vi "TLB Native Dynamic Events ver 0.17g.vi"() -> ()   [LabVIEW 2018]
uses:
  Labview Training Phase 2/Enum Controls/States for Action Engine.ctl
  TLB Type Definitions/State Type Definitions.ctl
  TLB Type Definitions/Intruction Type Definitions.ctl
  TLB Type Definitions/Encoder cluster.ctl
  TLB Type Definitions/PING CLUSTER.ctl
  <vilib>/Studica/Studica Toolkit/NavX/NavX.lvlib
  <vilib>/Studica/Studica Toolkit/Background/DIO Channel.ctl
  Underlying VI's/NavX VI/navX type def.ctl
  <vilib>/Studica/Studica Toolkit/Background/I2C Channel.ctl
  TLB Type Definitions/Vision cluster.ctl
  <vilib>/NI_Real-Time Target Support.lvlib
  TLB Type Definitions/Stepper cluster.ctl
  Experimental VI's/Archived VI's/MOTOR CONTROL NO PID Type Def.ctl
  Underlying VI's/I2C Master VI/I2C MASTER Type Def.ctl
  Underlying VI's/I2C Master VI/I2C_MASTER_WRITE_NEW Type Def.ctl
  <vilib>/userdefined/High Color/IMAQdx.ctl
  Underlying VI's/I2C Master VI/Arduino_Interfacing.ctl
  TLB Type Definitions/Yaw Cluster.ctl
  TLB Type Definitions/Time cluster.ctl
  TLB Type Definitions/Y Stepper cluster.ctl
  Underlying VI's/Modified webcam FGV/Webcam AE.ctl
  Underlying VI's/Elasped Timer/Elapsed timer control.ctl
  Underlying VI's/Motor Control VI with PID/MOTOR CONTROL WITH PID AE DATA MODE TYPE DEF.ctl
  Underlying VI's/Motor Control VI with PID/MOTOR CONTROL WITH PID AE DIRECTION TYPE DEF.ctl
  TLB Type Definitions/IR Sensor Type Def.ctl
  <vilib>/myRIO/Common/Instrument Driver Framework/myRIO v1.0/AI/typedefs/AI Channels Enum.ctl
  <vilib>/myRIO/Common/Instrument Driver Framework/myRIO v1.0/AI/typedefs/AI Channels List.ctl
  TLB Type Definitions/Motor Speed Cluster.ctl
  <vilib>/Utility/RT CPU Load.ctl
panel:
  out "x-y":dbl
  out "Left IR Sensor":dbl
  out "Obstacle detected":bool
  out "Speed & distance":T1
  out "Object Center Coordinates":cluster{"x":sgl, "y":sgl}
  out "Object detection cluster":T2
  out "Time up flag":bool
  out "Task selection":u8
  in  "Object recognition mode":enum16{"Ball", "Soap", "Gel", "Pipe", "None"}(ring)
  out "NavX Readings":T3
  out "Arduino Data":T4
  out "CPU loads":T5[](array[typedef]) {"ISR (%)" format="%#.2f"; "Idle (%)" format="%#.2f"; "Background (%)" format="%#.2f"; "Normal (%)" format="%#.2f"; "Above Normal (%)" format="%#.2f"; "High (%)" format="%#.2g"; "Timed Structures (%)" format="%#.2g"; "Time Critical (%)" format="%#.2g"; "Total (%)" format="%#.2g"}
  out "TASK ENABLE":bool
  out "Rising Edge":bool
  in  "Green LED":bool
  out "I2C Error":errorcluster
  out "State Logic":T6=enum."Startup"
  out "elements":T7[](array[typedef])
  in  "STOP TASK":bool
  in  "OK Button":bool
  in  "STOP":bool
  out "error out":errorcluster
  out "Action Queue Items":i32
  out "State Logic Queue Items":i32
  out "Action Queues items":string[](array[string])=["Hardware reset", "Software reset", ""]
  out "Action State":string
  # "System Health Status Update"
  # "VISION"
  # "TLB FRAMEWORK STATUS"
  # "Test Programme written by Calvin Loke    Dated: 28 Aug 2019\nTest Programme revised by Dr Alex See   Dated 30 Aug 2019\n\nRevision date: 20/03/2020\nProgramme version:   TLB Native Dynamic Events ver 0.14a"
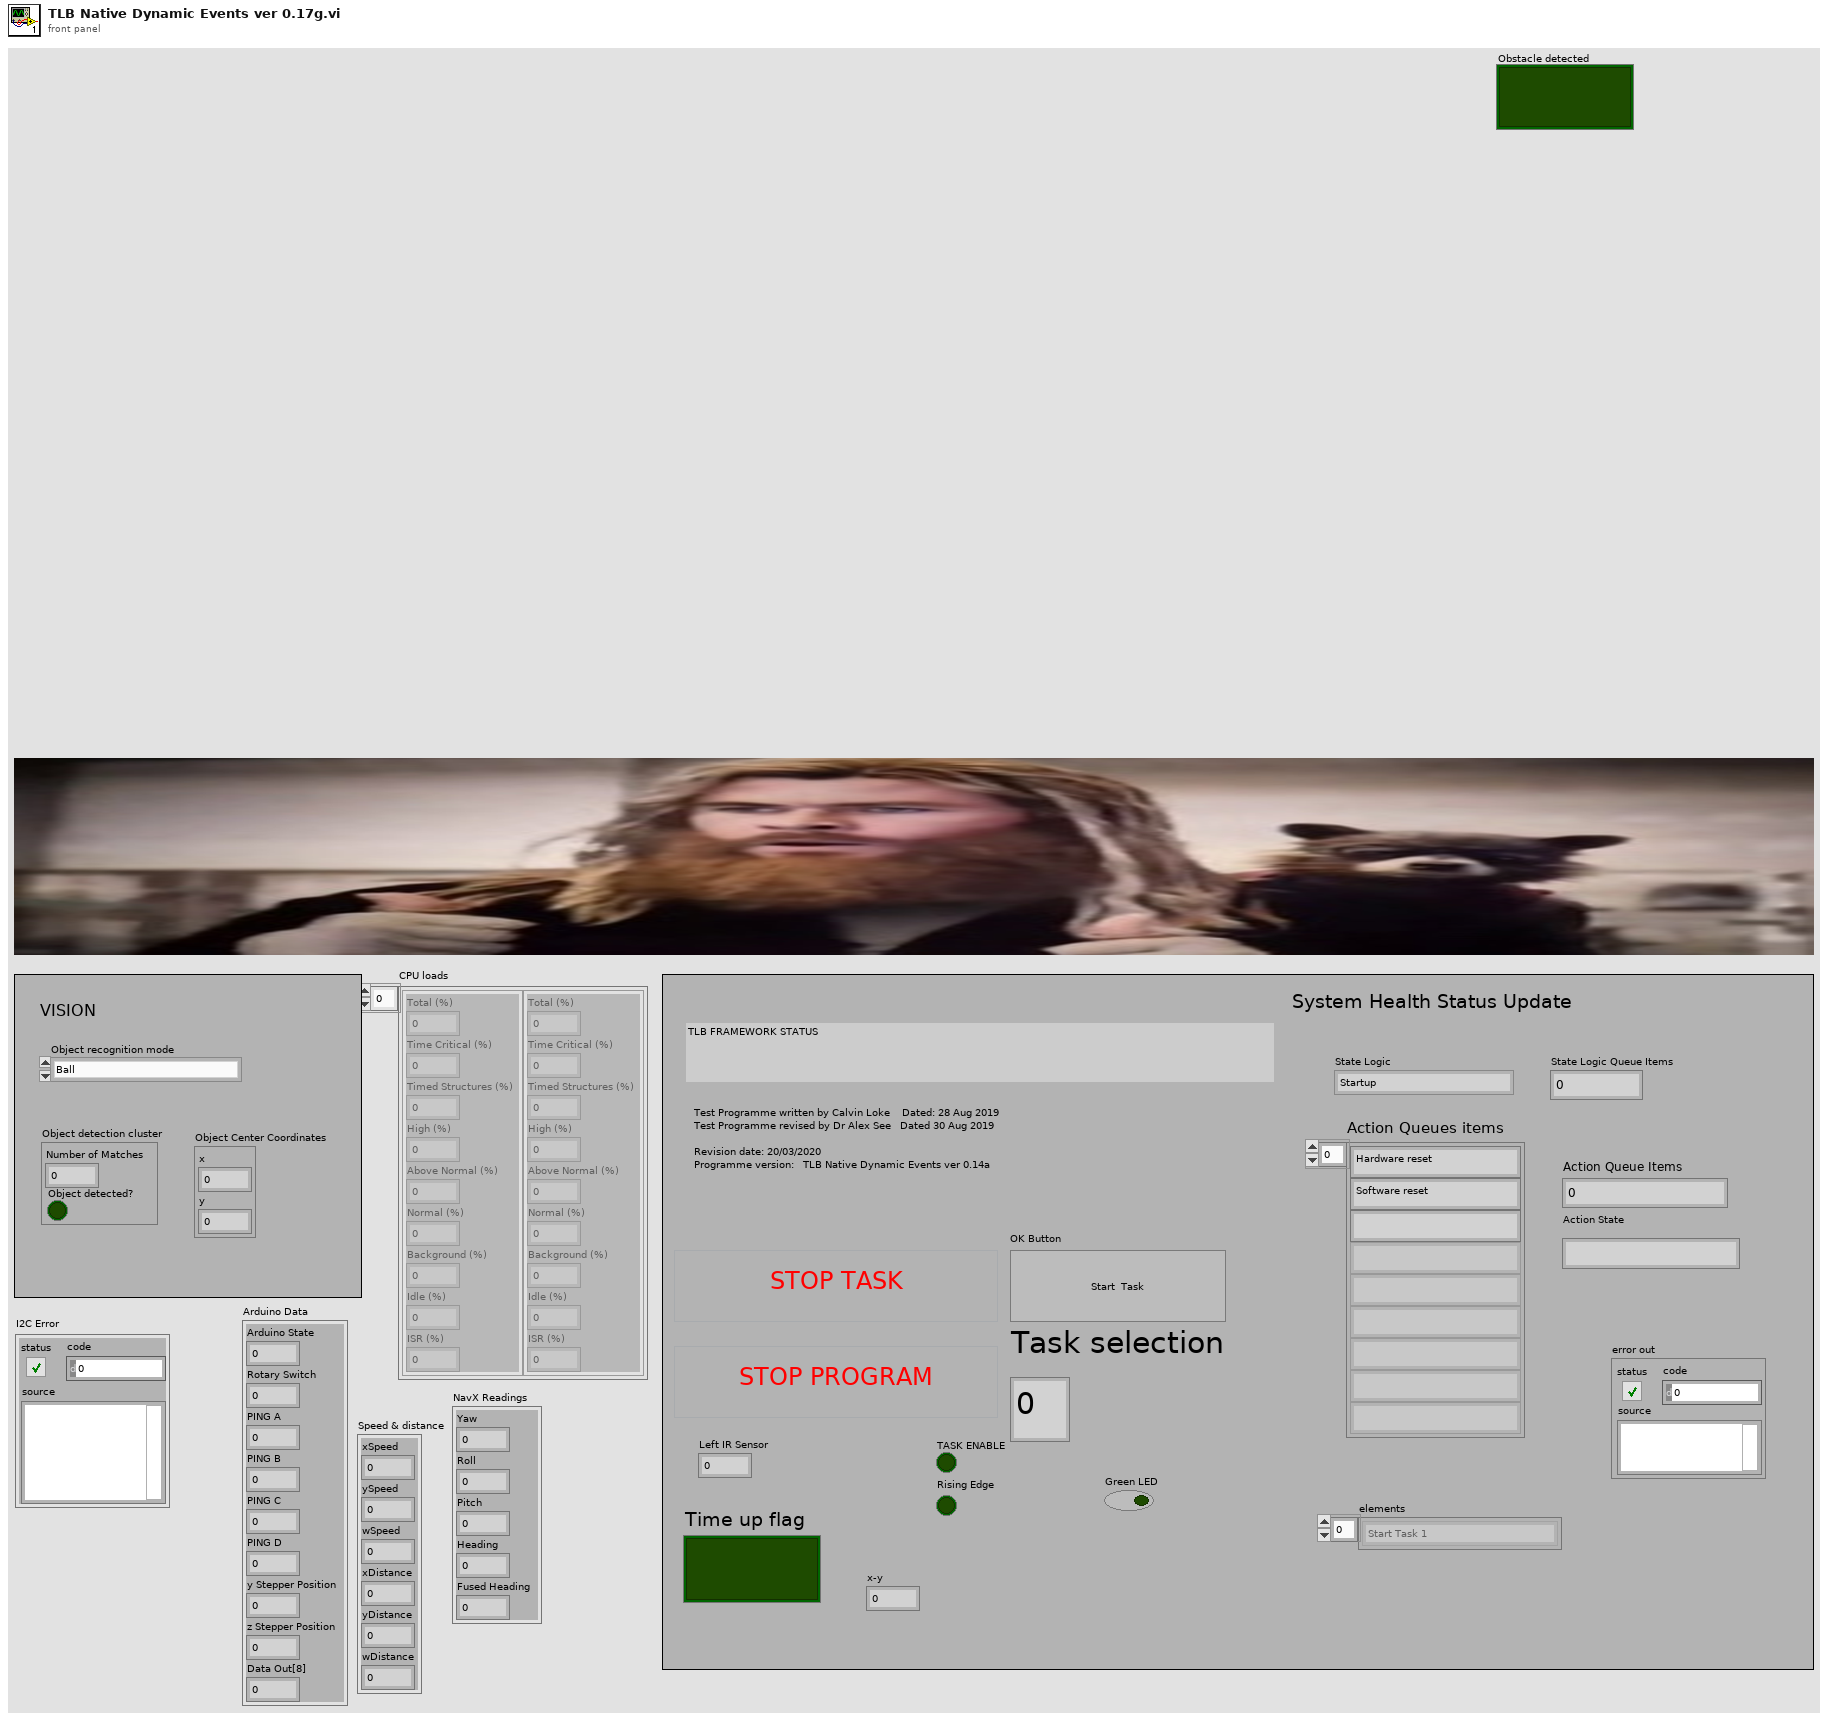
[diagram p1: front panel]
types:
  T1 = cluster{"xSpeed":dbl, "ySpeed":dbl, "wSpeed":dbl, "xDistance":dbl, "yDistance":dbl, "wDistance":dbl}
  T2 = cluster{"Number of Matches":i32, "Object detected?":bool}
  T3 = cluster{"Yaw":dbl, "Roll":dbl, "Pitch":dbl, "Heading":dbl, "Fused Heading":dbl}
  T4 = cluster{"Arduino State":u8, "Rotary Switch":u8, "PING A":u8, "PING B":u8, "PING C":u8, "PING D":u8, "y Stepper Position":u8, "z Stepper Position":u8, "Data Out[8]":u8}
  T5 = typedef "NI_Real-Time Target Support.lvlib/RT CPU Load.ctl" = cluster{"Total (%)":dbl, "Time Critical (%)":dbl, "Timed Structures (%)":dbl, "High (%)":dbl, "Above Normal (%)":dbl, "Normal (%)":dbl, "Background (%)":dbl, "Idle (%)":dbl, "ISR (%)":dbl}
  T6 = typedef "State Type Definitions.ctl" = enum16{"None", "Startup", "Move to Angle", "True Stop", "Idle", "Shutdown", "Task 1A", "Task 1B", "Task 2:Raise Arm", "Task 2:Sensor Mode", "Task 2:Reverse Mode", "Task 3", "Task 4_A", "Task 4_B", "Task 4_C", "Task 4_D", "Task 5A", "Task 5B", "Task 5C", "Task 5D", "Task 5E: POSITION ARM", "Task 5F: ARM GRAB HEIGHT", "Task 5G: CLOSE CLAW", "Task 5H: RAISE ARM", "Task 6_A", "Task 6_B", "Task 7", "Task 8A: RAISE ARM", "Task 8B: MOVE TO BOX", "Task 8C: CAM BURST", "Task 8D: PROCESS IMAGE", "Task 8E: ROBOT ADJUST", "Task 8F: CAM BURST 2", "Task 8G: PROCESS IMAGE 2", "Task 8H: ARM ADJUST", "Task 8I: ARM GRAB HEIGHT", "Task 8J: CLOSE CLAW", "Task 8K: RAISE MY SWORD", "Task 9A: Raise Arm", "Task 9B: Rotate to Angle", "Task 9C: Detect Box", "Task 9D: MOVE FORWARD", "Task 9E: MOVE LEFT", "Task 9F: SCAN IMAGE", "Task 9G: PROCESS COLOUR", "Task 9H: MOVE RIGHT", "Task 9I: SCAN IMAGE", "Task 9J: PROCESS COLOUR", "Task 9K: ROTATE 90 CW", "Task 9L: MOVE FORWARD", "Task 9M: MOVE RIGHT", "Task 9N: SCAN IMAGE", "Task 9O: PROCESS COLOUR", "Task 9P: MOVE RIGHT", "Task 9Q: SCAN IMAGE", "Task 9R: PROCESS COLOUR", "Task A1: Raise Arm", "Task A2: Rotate to Angle", "Task A3: Move Forward", "Task A4: Rotate CW 90"}
  T7 = typedef "Intruction Type Definitions.ctl" = enum16{"None", "Start Task 1", "Start Task 2", "Start Task 3", "Start Task 4", "Start Task 5", "Start Task 6", "Start Task 7", "Start Task 8 - BALL", "Start Task 8 - Gel", "Start Task 8 - Pipe", "Start Task 8 - Soap", "Start Task 9", "Start Task A", "Start Task B", "Exit"}
  T8 = typedef "Motor Speed Cluster.ctl" = cluster{"ySpeed":dbl, "xSpeed":dbl, "wSpeed":dbl}
  T9 = typedef "IR Sensor Type Def.ctl" = cluster{"Left IR Sensor":dbl, "Arm IR Sensor":dbl, "Bottom IR Sensor":dbl}
  T10 = typedef "Y Stepper cluster.ctl" = cluster{"yStepper desired":u8}
  T11 = typedef "Time cluster.ctl" = cluster{"Time up flag":bool, "SET TIME TO CHECK":dbl}
  T12 = typedef "Yaw Cluster.ctl" = cluster{"Yaw":dbl, "Compass":dbl}
  T13 = typedef "Stepper cluster.ctl" = cluster{"y Stepper Position":u8, "z Stepper Position":u8}
  T14 = typedef "DIO Channel.ctl" = enum16{"Not Connected", "A/DIO1", "A/DIO2", "A/DIO3", "A/DIO4", "A/DIO5", "A/DIO6", "A/DIO7", "A/DIO13", "B/DIO1", "B/DIO2", "B/DIO3", "B/DIO4", "B/DIO5", "B/DIO6", "B/DIO7", "B/DIO13", "C/DIO0", "C/DIO1", "C/DIO2", "C/DIO3", "C/DIO4", "C/DIO5", "C/DIO6", "C/DIO7"}
  T15 = typedef "Vision cluster.ctl" = cluster{"Recognized Object":bool, "Object X coordinate":dbl, "Object Y coordinate":dbl}
  T16 = typedef "PING CLUSTER.ctl" = cluster{"PING_A":u8, "PING_B":u8, "PING_C":u8, "PING_D":u8}
  T17 = typedef "Encoder cluster.ctl" = cluster{"xDistance":dbl, "yDistance":dbl, "wDistance":dbl}
  T18 = cluster{"DIO Channel":T14, "FPGA VI Reference Out":refnum<k20>}
  T19 = typedef "navX type def.ctl" = enum16{"Get i2C reference", "Read Values", "Zero Yaw"}
  T20 = typedef "Arduino_Interfacing.ctl" = enum16{"Initialize", "Write to Arduino", "Read From Arduino"}
  T21 = typedef "I2C Channel.ctl" = enum16{"Not Connected", "A", "B"}
  T22 = typedef "States for Action Engine.ctl" = enum16{"Initialize", "Write", "Read"}
  T23 = cluster{"I2C Ref Out":cluster{"I2C Channel":T21, "FPGA VI Reference Out":refnum<k20>}, "Connected":bool, "Slave Address (7-bit)":u8, "Registry":u8[]}
  T24 = typedef "Intruction Type Definitions.ctl" = enum16{"None", "Start Task 1", "Start Task 2", "Start Task 3", "Start Task 4", "Start Task 5", "Start Task 6", "Start Task 7", "Start Task 8", "Start Task 9", "Start Task A", "Start Task B", "Exit"}
  T25 = typedef "IMAQ Image.ctl" = refnum<image>
  T26 = typedef "State Type Definitions.ctl" = enum16{"None", "Startup", "Move to Angle", "True Stop", "Idle", "Shutdown", "Task 1", "Task 2:Raise Arm", "Task 2:Sensor Mode", "Task 2:Reverse Mode", "Task 3", "Task 4_A", "Task 4_B", "Task 4_C", "Task 4_D", "Task 5A: ARM CAM HEIGHT", "Task 5B: MOVE TO BOX", "Task 5C: CAM BURST", "Task 5D: PROCESS IMAGE", "Task 5E: POSITION ARM", "Task 5F: ARM GRAB HEIGHT", "Task 5G: CLOSE CLAW", "Task 5H: RAISE ARM", "Task 6_A", "Task 6_B", "Task 7", "Task 8A: RAISE ARM", "Task 8B: MOVE TO BOX", "Task 8C: CAM BURST", "Task 8D: PROCESS IMAGE", "Task 8E: ROBOT ADJUST", "Task 9A: Raise Arm", "Task 9B: Rotate to Angle", "Task 9C: Rotation alignmnet", "Task B"}
  T27 = typedef "MOTOR CONTROL WITH PID AE DIRECTION TYPE DEF.ctl" = enum16{"y-axis movement", "x-axis movement", "rotation", "stop", "reset encoders"}
  T28 = typedef "MOTOR CONTROL WITH PID AE DATA MODE TYPE DEF.ctl" = enum16{"Init AE", "Write to AE", "Read from AE"}
  T29 = typedef "Elapsed timer control.ctl" = enum16{"Start", "Pause", "Initialize"}
  T30 = typedef "I2C_MASTER_WRITE_NEW Type Def.ctl" = enum16{"Ultrasonic sensors", "Stepper origin", "zStepper 13.3k", "zStepper 13k", "zStepper 12k", "zStepper 11k", "zStepper 10k", "zStepper 9k", "zStepper 8k", "zStepper 7k", "zStepper 6k", "zStepper 5k", "zStepper 4k", "zStepper 3k", "zStepper 2k", "zStepper 1k", "zStepper 900", "zStepper 800", "zStepper 700", "zStepper 600", "zStepper 500", "zStepper 400", "zStepper 300", "zStepper 200", "zStepper 100", "zStepper 0", "yStepper control", "Open Claw", "Close Claw", "Soft Reset"}
  T31 = typedef "Webcam AE.ctl" = enum16{"Initialize Camera", "Open Camera", "Continuous Acquisition", "Close Camera", "Retrieve Image", "Dispose Camera Image Buffer"}
  T32 = typedef "IMAQdx.ctl" = refnum<k21>
  T33 = typedef "Webcam AE.ctl" = enum16{"Initialize Camera", "Open Camera", "Continuous Acquisition", "Close Camera", "Retrieve Image", "Dispose Image Buffers"}
  T34 = typedef "MOTOR CONTROL NO PID Type Def.ctl" = enum16{"Init", "Front Back", "Left Right", "Rotate", "Stop", "Latch"}
  T35 = typedef "AI Channels List.ctl" = T36[]
  T36 = typedef "AI Channels Enum.ctl" = enum16{"Not Connected", "AudioIn/Left", "AudioIn/Right", "C/AI0", "C/AI1", "A/AI0", "A/AI1", "A/AI2", "A/AI3", "A/AI4", "A/AI5", "A/AI6", "A/AI7", "B/AI0", "B/AI1", "B/AI2", "B/AI3", "B/AI4", "B/AI5", "B/AI6", "B/AI7", "AI/AI0", "AI/AI1", "AI/AI2", "AI/AI3", "A/AI0 (DIFF)", "A/AI1 (DIFF)", "A/AI2 (DIFF)", "A/AI3 (DIFF)", "B/AI0 (DIFF)", "B/AI1 (DIFF)", "B/AI2 (DIFF)", "B/AI3 (DIFF)"}
  T37 = typedef "I2C MASTER Type Def.ctl" = enum16{"Last State", "Mode 0", "Mode 1", "Mode 2", "Mode 3", "Mode 4", "Mode 5", "Mode 6", "Mode 7", "Mode 8", "Mode 9", "Mode 10"}
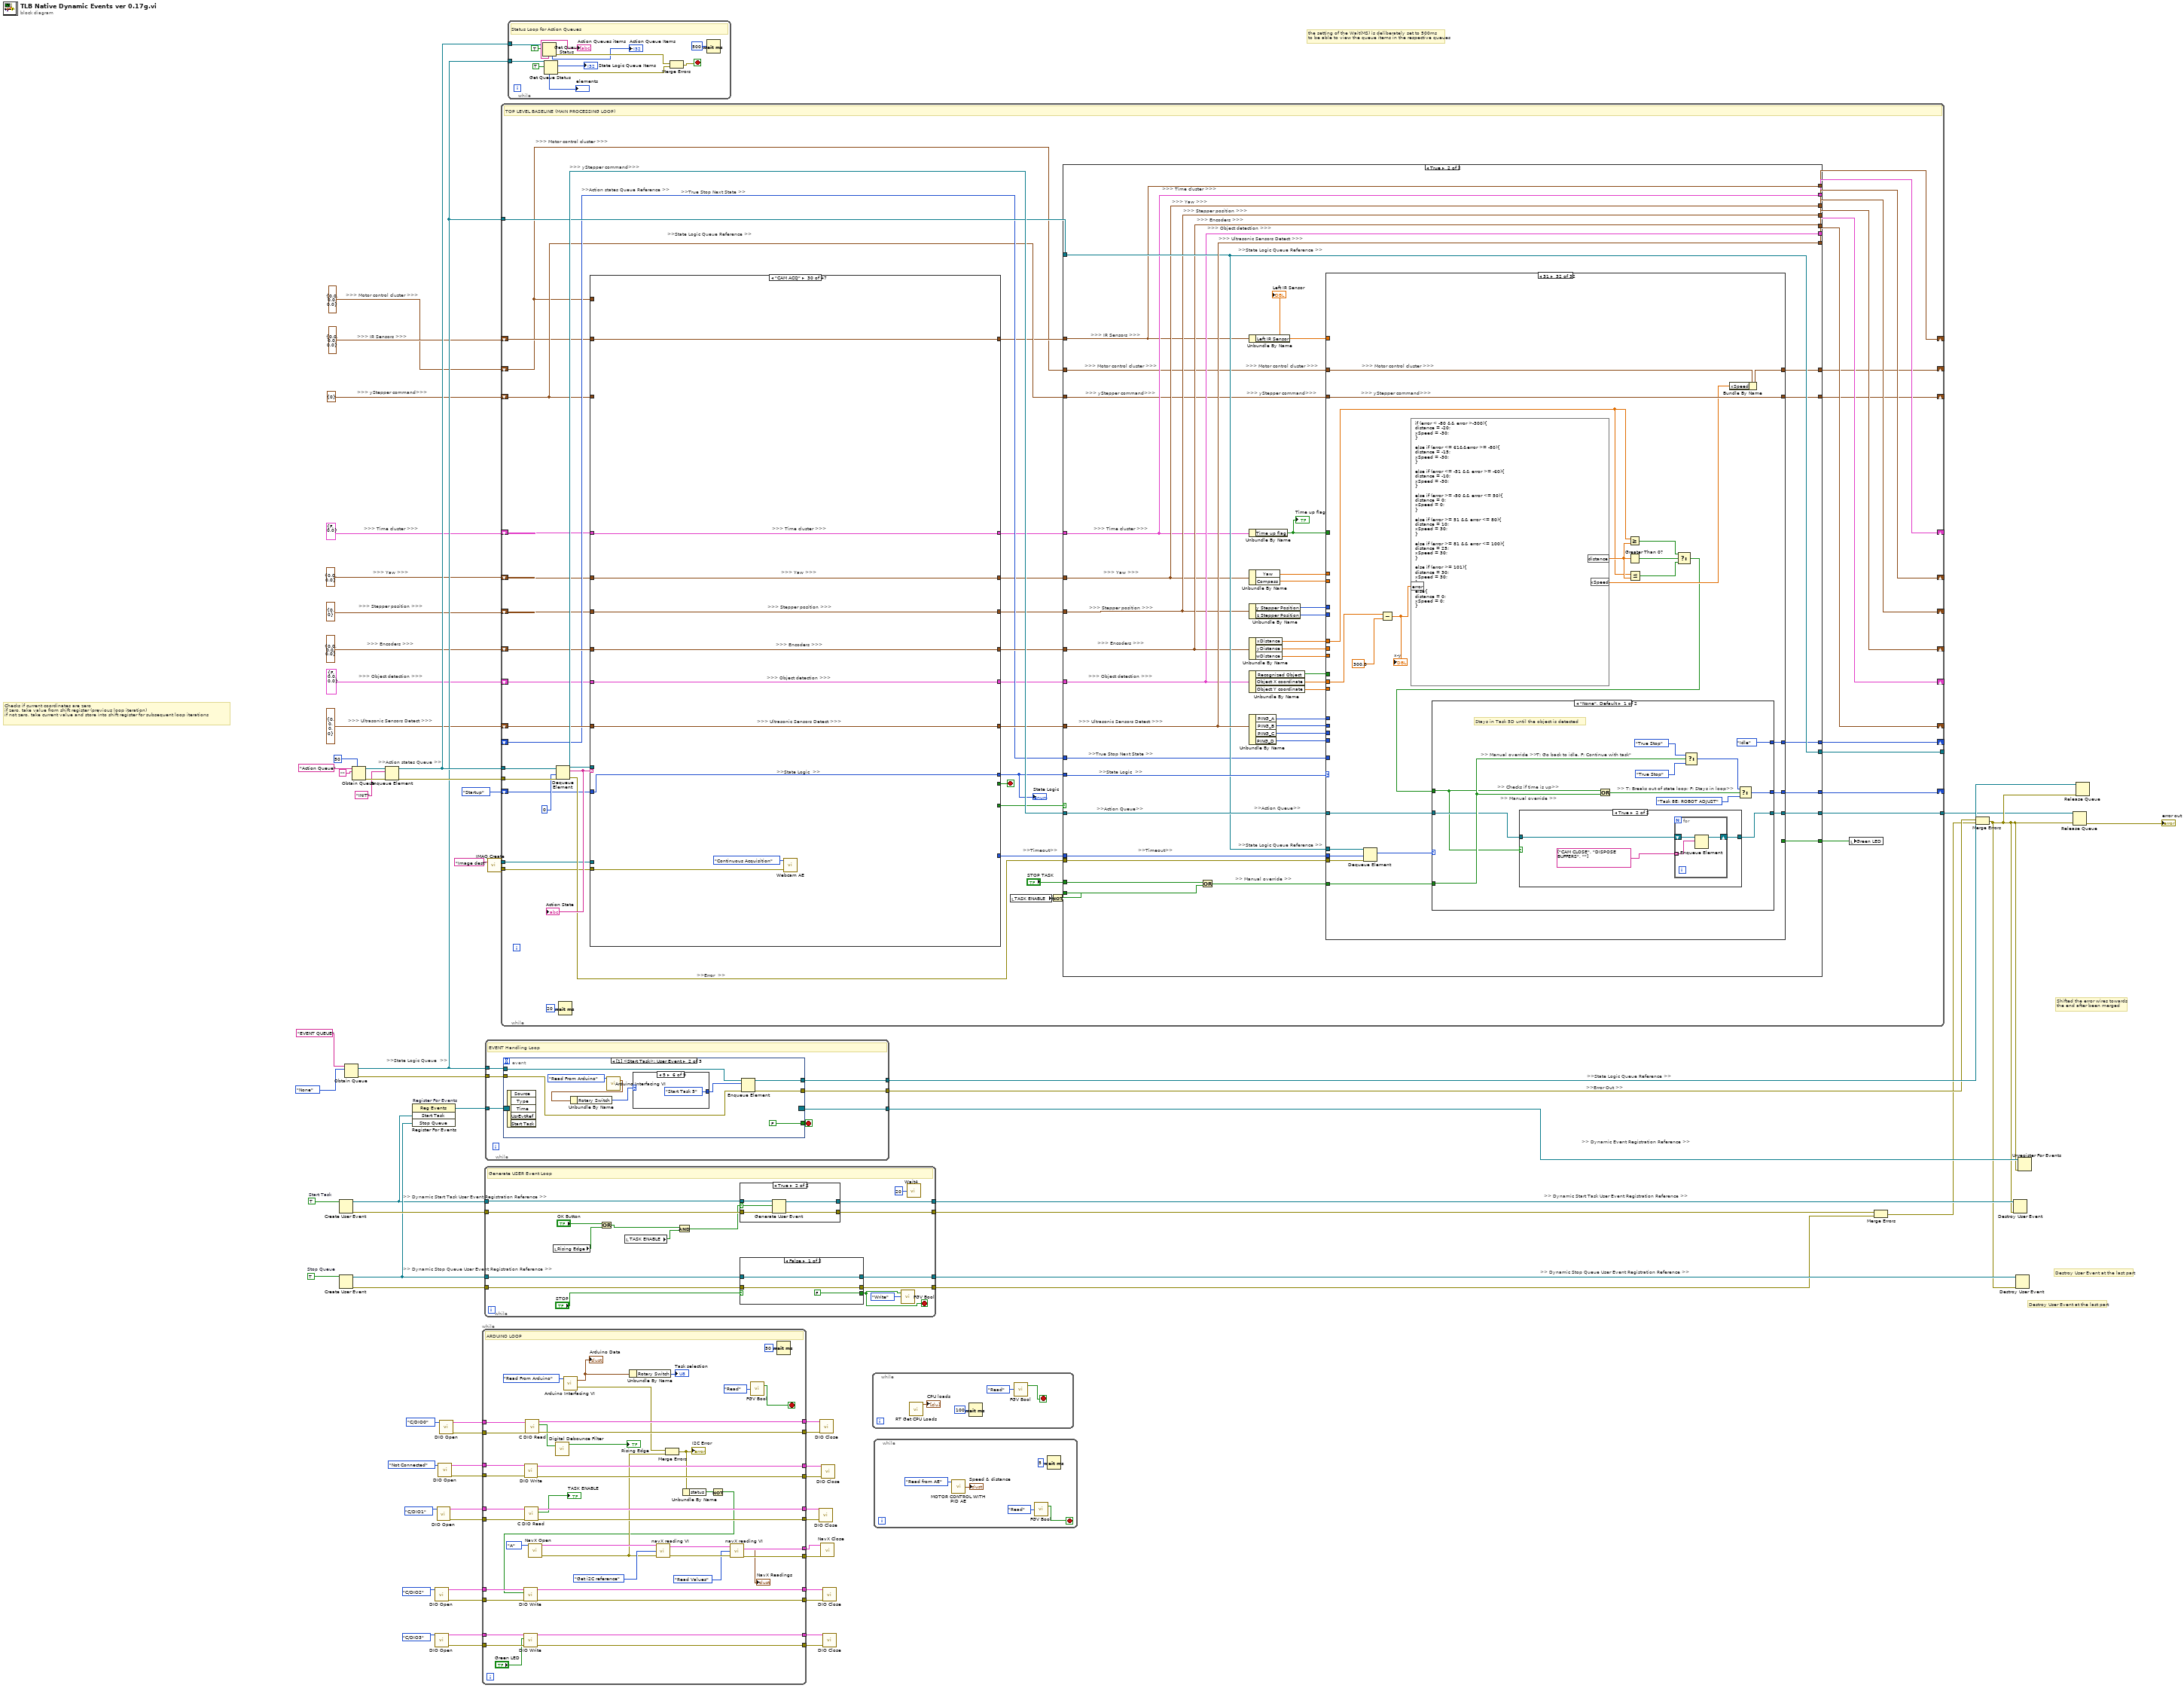
[diagram p0: block diagram]
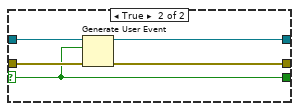
[diagram p2: hidden frame]
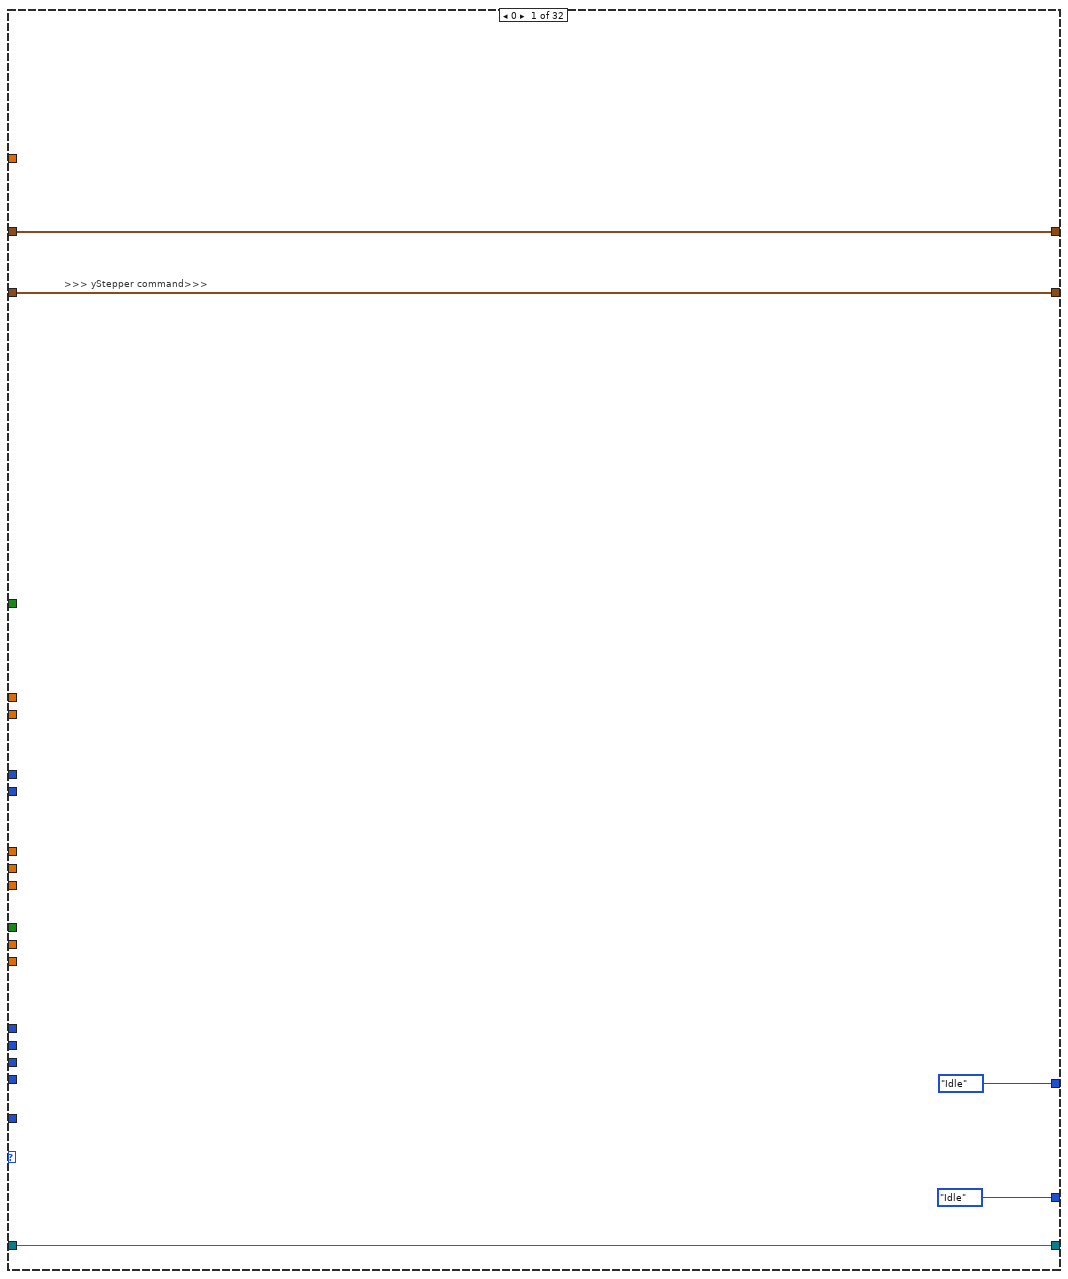
[diagram p5: hidden frame]
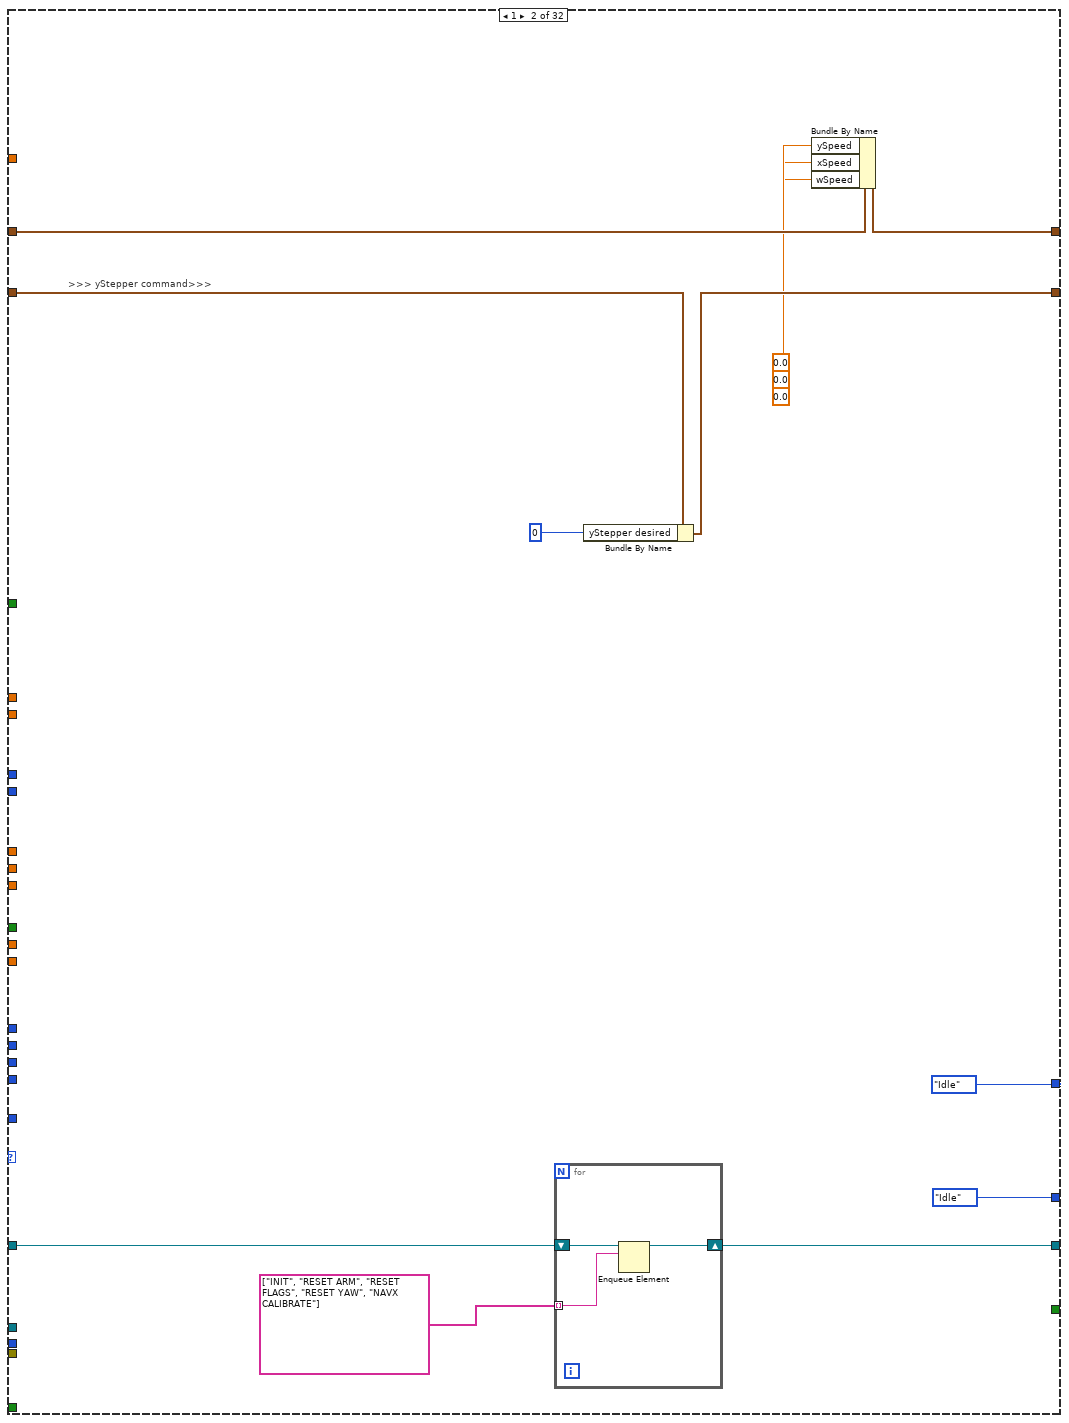
[diagram p6: hidden frame]
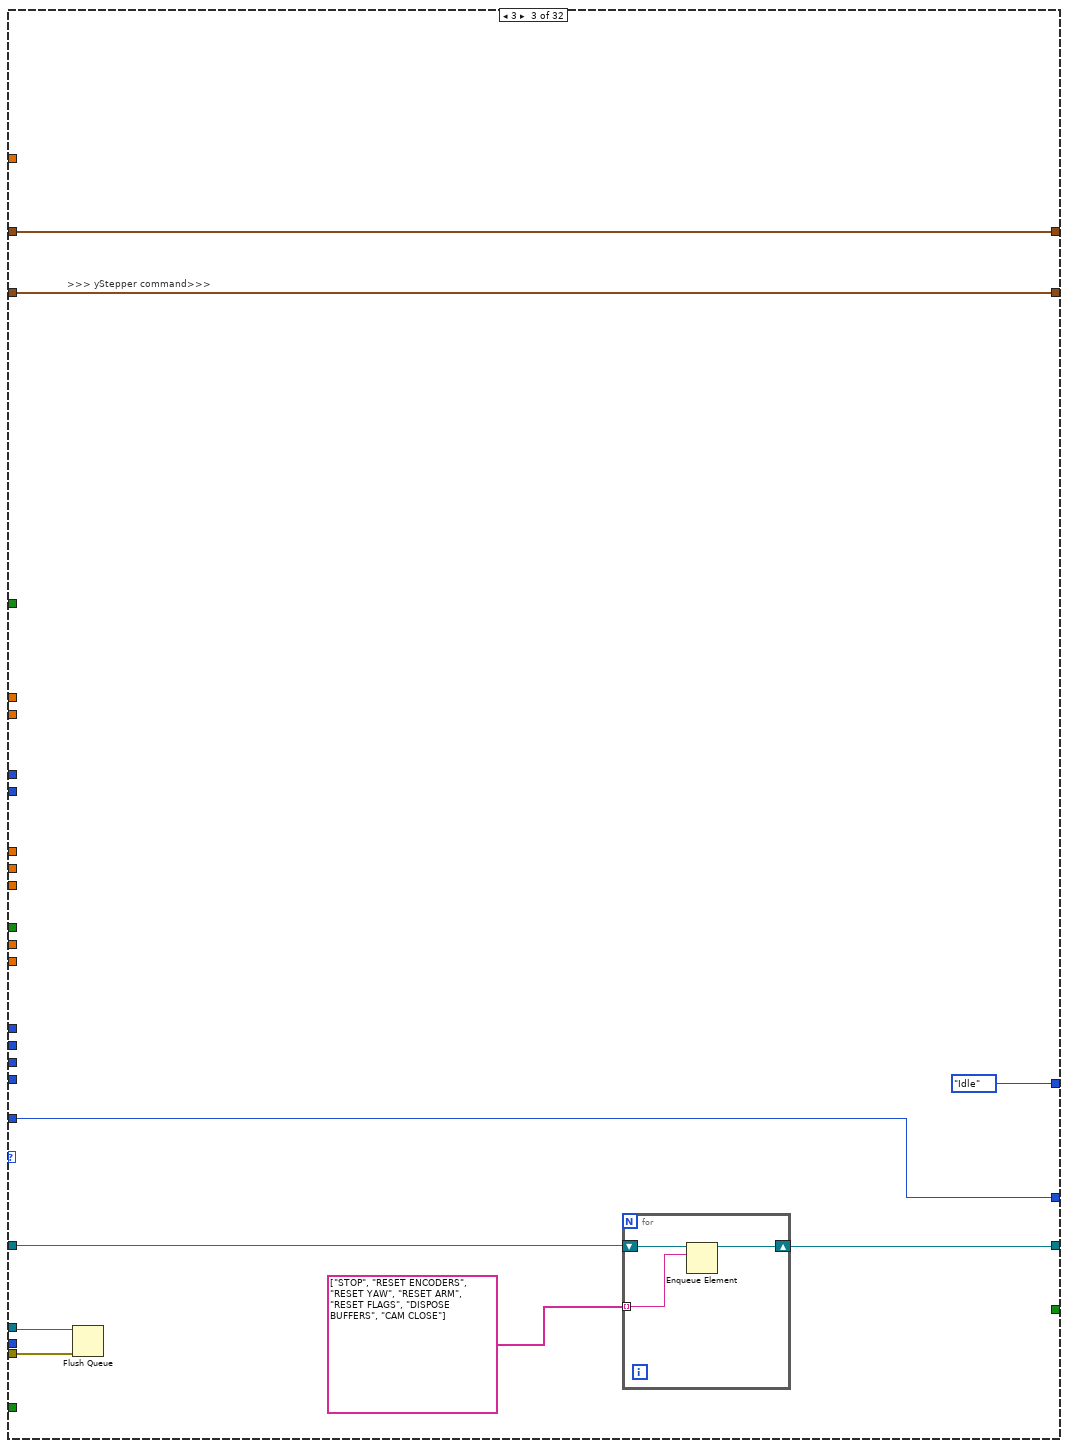
[diagram p7: hidden frame]
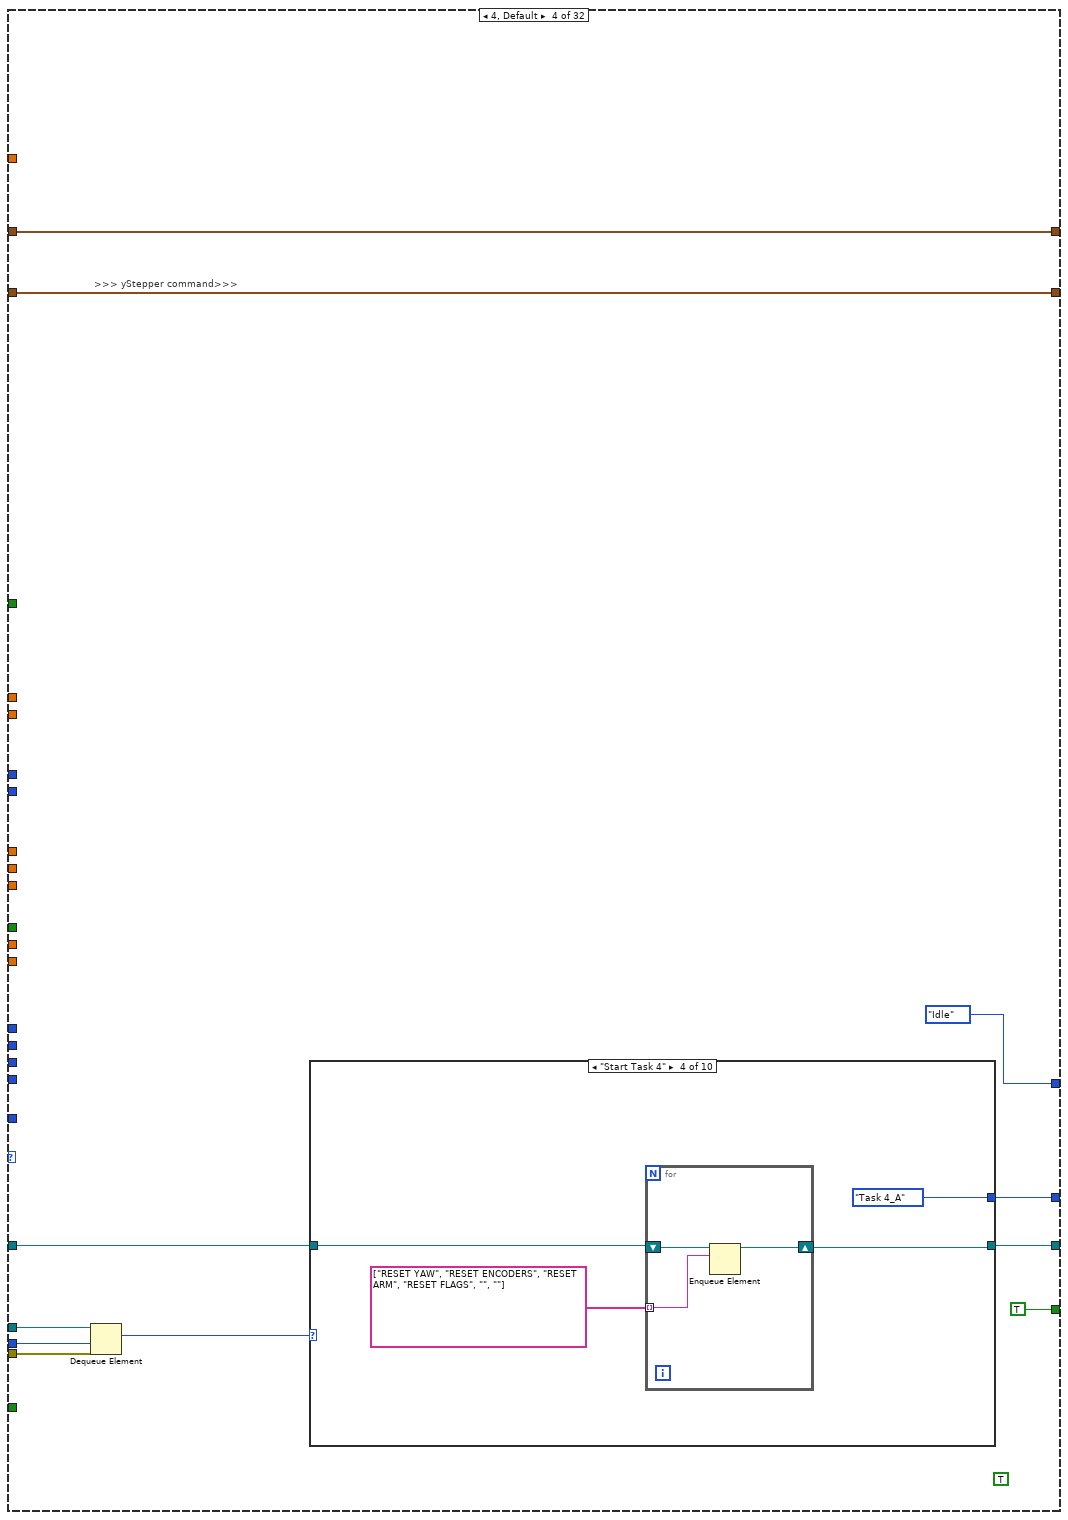
[diagram p8: hidden frame]
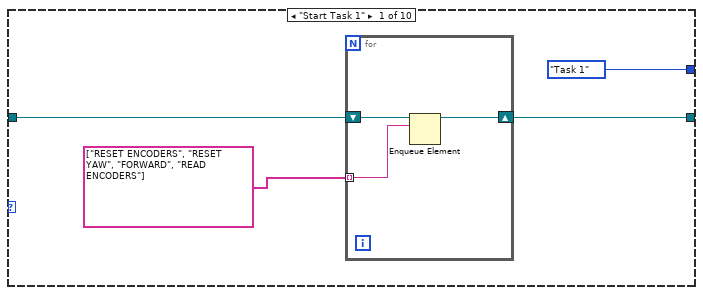
[diagram p9: hidden frame]
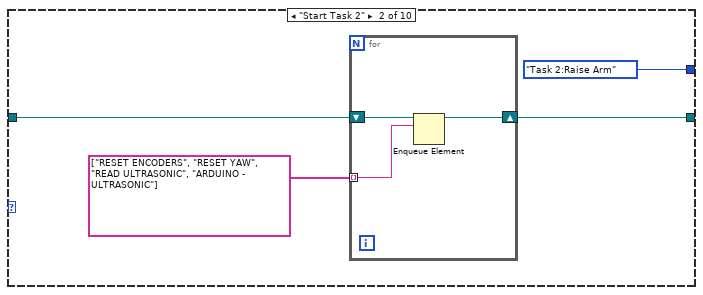
[diagram p10: hidden frame]
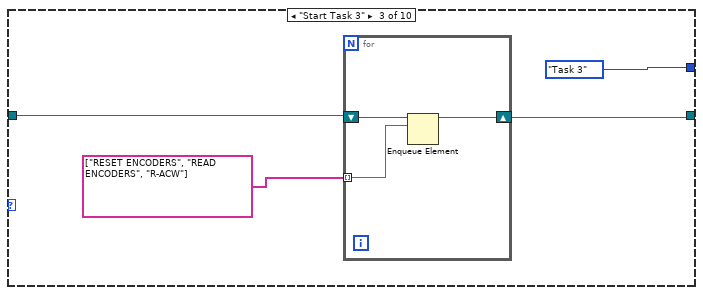
[diagram p11: hidden frame]
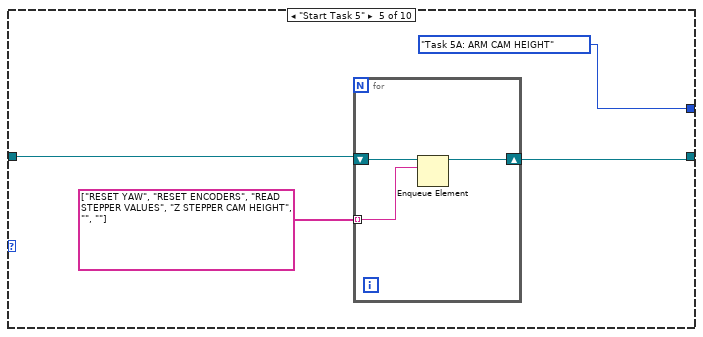
[diagram p12: hidden frame]
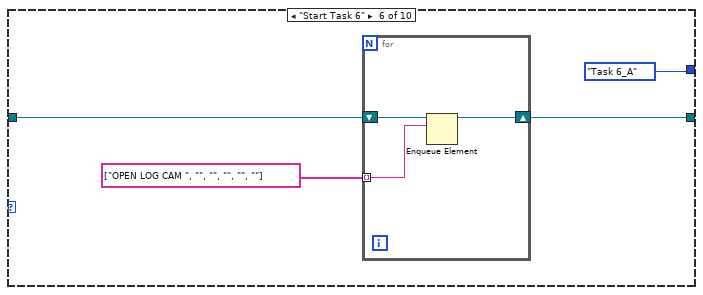
[diagram p13: hidden frame]
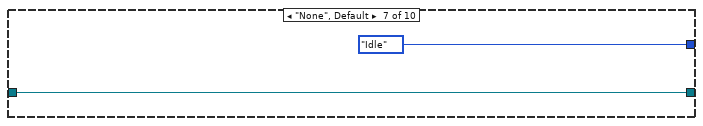
[diagram p14: hidden frame]
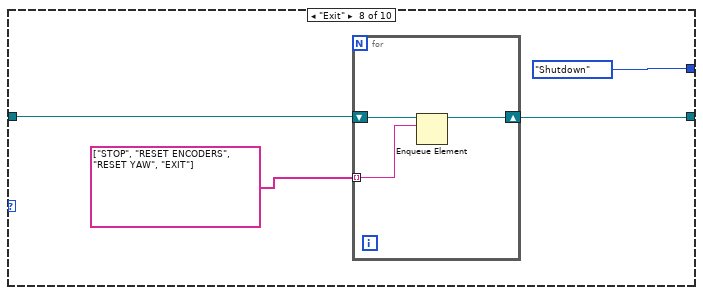
[diagram p15: hidden frame]
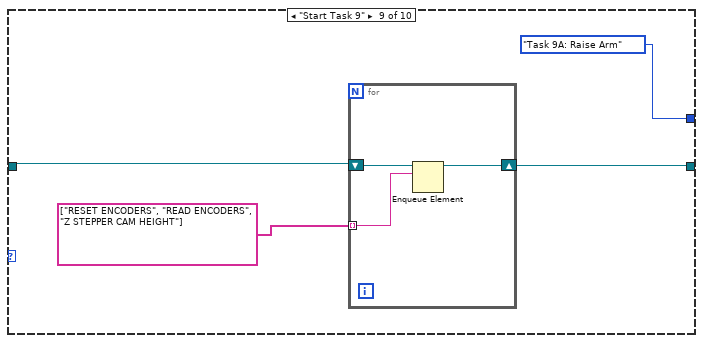
[diagram p16: hidden frame]
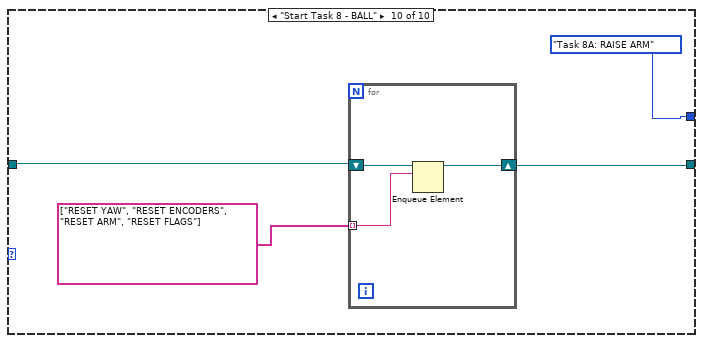
[diagram p17: hidden frame]
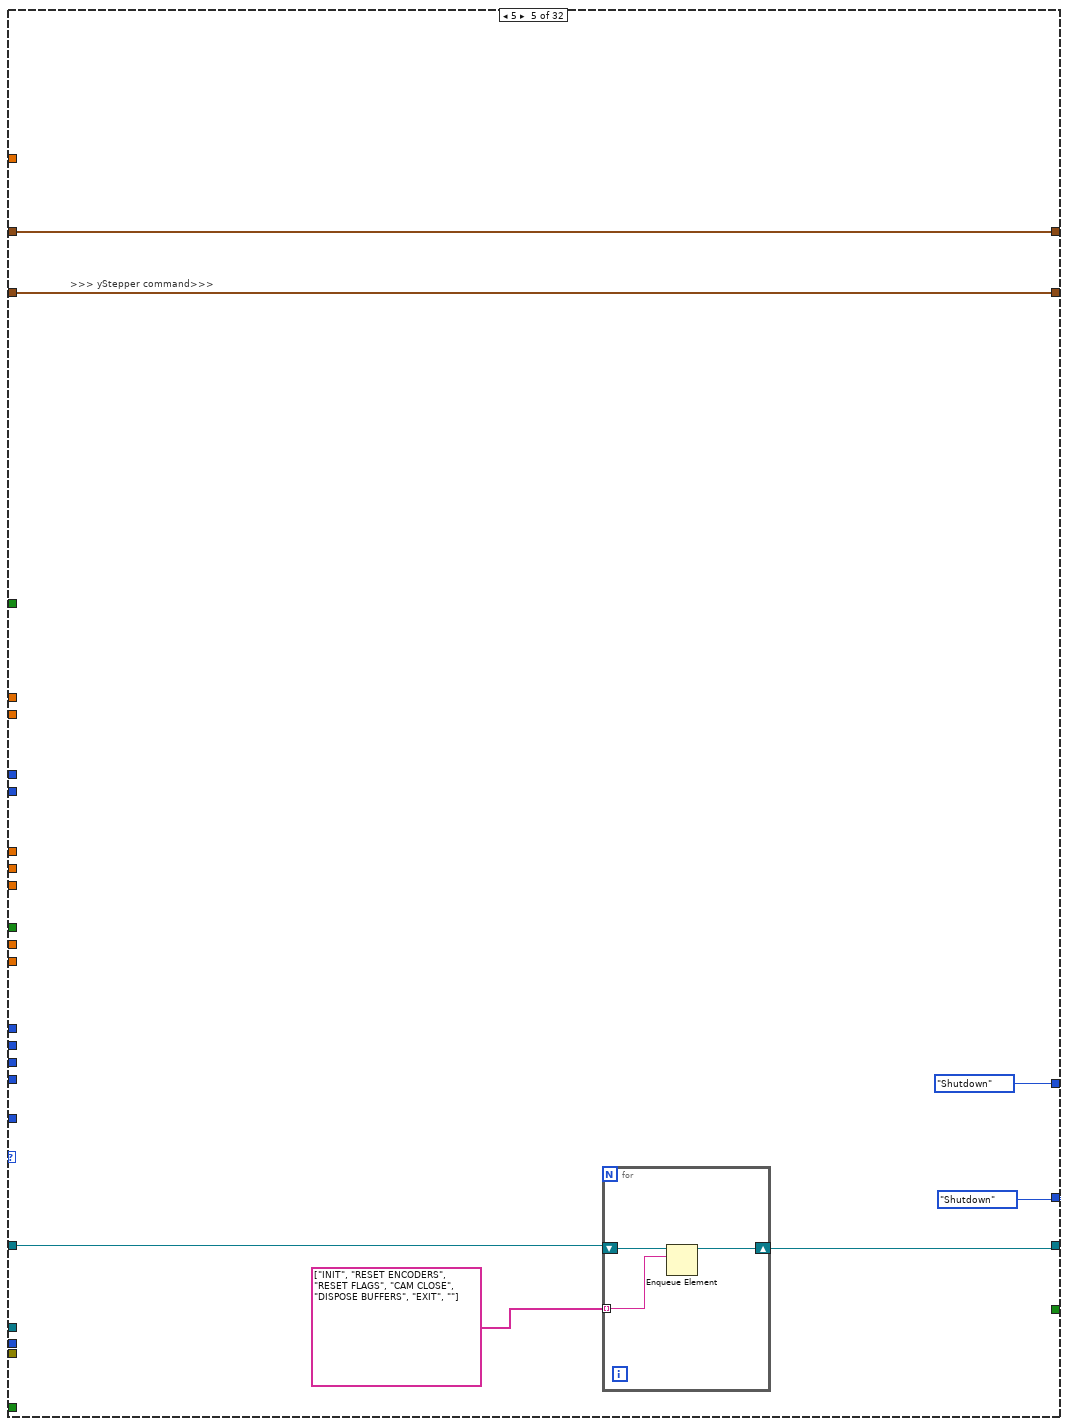
[diagram p18: hidden frame]
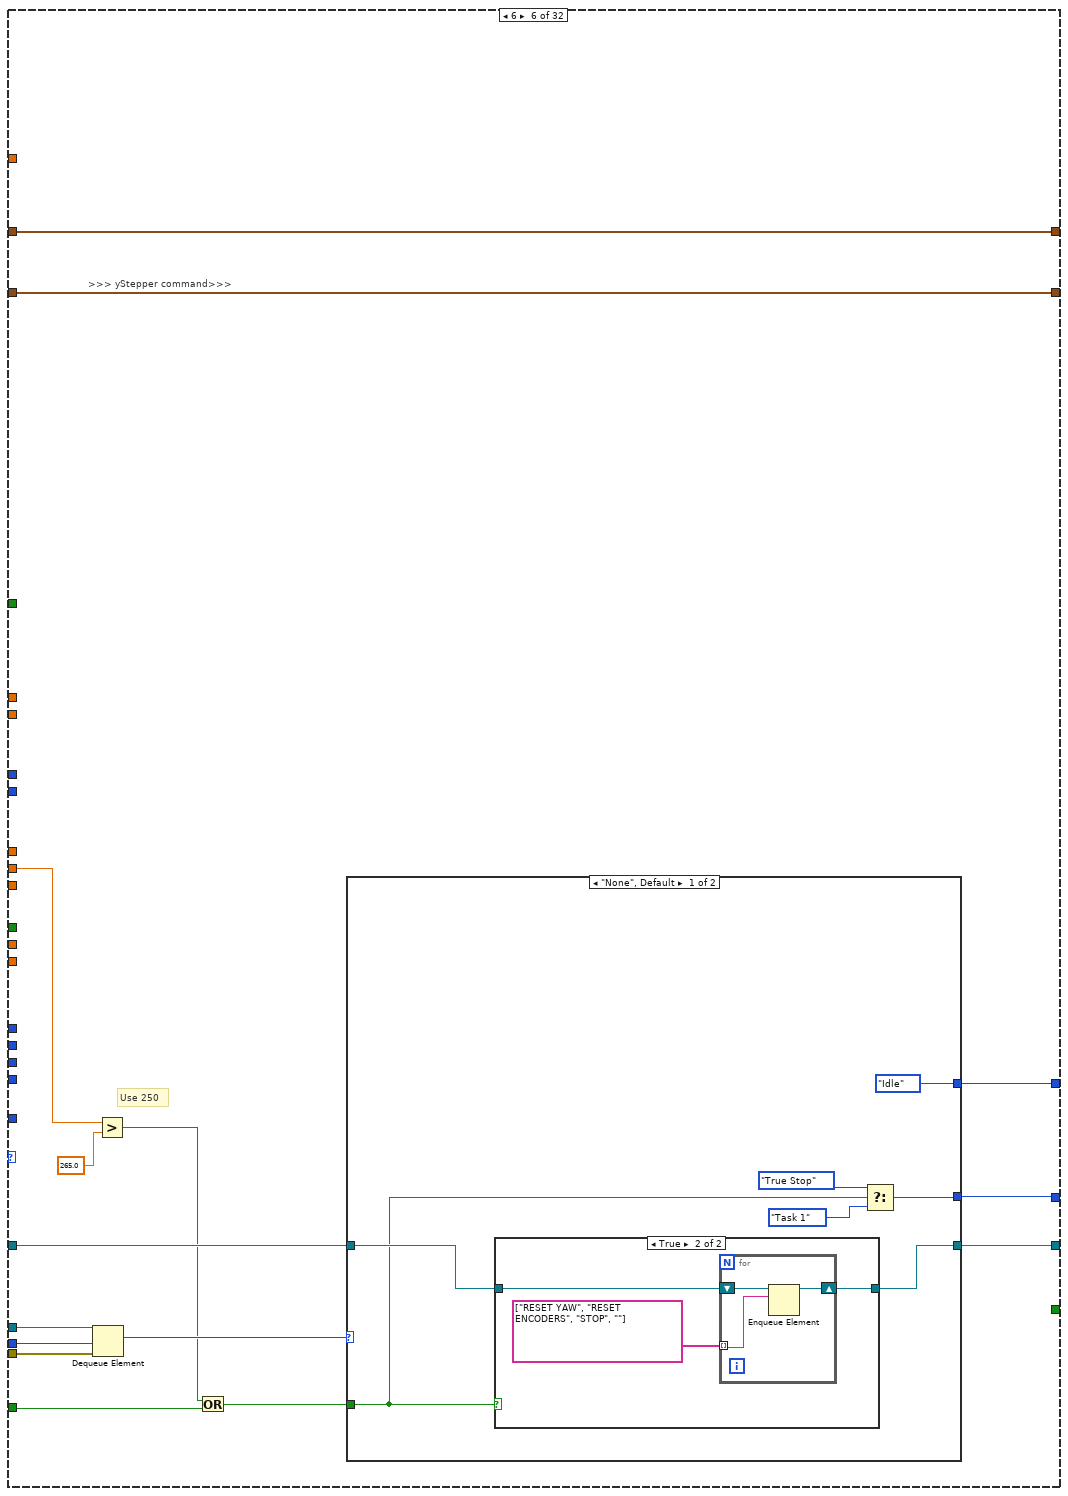
[diagram p19: hidden frame]
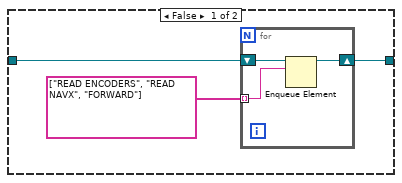
[diagram p20: hidden frame]
diagram:
  w70 = TRUE  # Stop Queue
  w69 = TRUE  # Start Task
  # ">>> Motor control cluster >>>"
  # ">>> IR Sensors >>>"
  # "Checks if current coordinates are zero\nif zero, take value from shift register (previous loop iteration)\nif not zero, take current value and store into shift register for subsequent loop iterations"
  # ">>> yStepper command>>>"
  # ">>> Time cluster >>>"
  # ">>> Yaw >>>"
  # ">>> Stepper position >>>"
  # ">>> Encoders >>>"
  # ">>> Object detection >>>"
  # ">>> Ultrasonic Sensors Detect >>>"
  # "the setting of the Wait(MS) is deliberately set to 500ms\nto be able to view the queue items in the respective queues"
  # ">>Error Out >>"
  # ">> Dynamic Stop Queue User Event Registration Reference >>"
  # ">> Dynamic Start Task User Event Registration Reference >>"
  # ">> Dynamic Stop Queue User Event Registration Reference >>"
  # ">> Dynamic Start Task User Event Registration Reference >>"
  # ">> Dynamic Event Registration Reference >>"
  # ">>Action states Queue >>"
  # ">>State Logic Queue  >>"
  # ">>State Logic Queue Reference >>"
  # "Destroy User Event at the last part"
  # "Destroy User Event at the last part"
  # "Shifted the error wires towards\nthe end after been merged"
  n1 = Create User Event(user event datatype=w69) -> (user event=w61:refnum<user-event>, error out=w66:errorcluster)  [unwired: 1 in]
  n2 = Create User Event(user event datatype=w70) -> (user event=w62:refnum<user-event>, error out=w65:errorcluster)  [unwired: 1 in]
  n3 = Obtain Queue(name (unnamed)="EVENT QUEUE", element data type=Intruction_Type_Definitions."None" ("Enum")) -> (queue out=w47:refnum<queue>, error out=w53:errorcluster)  [unwired: 3 in, 1 out]
  n4 = Obtain Queue(max queue size (-1, unlimited)=50, name (unnamed)="Action Queue", element data type="") -> (queue out=w56:refnum<queue>, error out=w52:errorcluster)  [unwired: 2 in, 1 out]
  n5 = Enqueue Element(queue=w56, element="INIT", error in (no error)=w52) -> (queue out=w48:refnum<queue>, error out=w51:errorcluster)  [unwired: 1 in, 1 out]
  n6 = register-events "Register For Events"(w61, w62) -> (reference out=w60:refnum<event-registration>)  [unwired: 2 in, 1 out]
  n7 = call <vilib>:"DIO Open.vi"("DIO Channel"=DIO_Channel."C/DIO2") -> ("error out"=w17:errorcluster, "DIO Info Out"=w18:T18)  [unwired: 9 in]
  n8 = call <vilib>:"DIO Open.vi"("DIO Channel"=DIO_Channel."C/DIO3") -> ("error out"=w12:errorcluster, "DIO Info Out"=w13:T18)  [unwired: 9 in]
  n9 = call <vilib>:"DIO Open.vi"("DIO Channel"=DIO_Channel."C/DIO1") -> ("error out"=w25:errorcluster, "DIO Info Out"=w26:T18)  [unwired: 9 in]
  n10 = call <vilib>:"DIO Open.vi"("DIO Channel"=DIO_Channel."Not Connected") -> ("error out"=w30:errorcluster, "DIO Info Out"=w32:T18)  [unwired: 9 in]
  n11 = call <vilib>:"DIO Open.vi"("DIO Channel"=DIO_Channel."C/DIO0") -> ("error out"=w35:errorcluster, "DIO Info Out"=w38:T18)  [unwired: 9 in]
  n12 = while {
    tunnel: w38 -> [w111]
    tunnel: [w110] -> w36
    tunnel: w35 -> [w109]
    tunnel: [w108] -> w34
    tunnel: w32 -> [w105]
    tunnel: [w104] -> w31
    tunnel: w30 -> [w103]
    tunnel: [w102] -> w29
    tunnel: [w101] -> w27
    tunnel: w26 -> [w100]
    tunnel: w25 -> [w99]
    tunnel: [w98] -> w24
    tunnel: w18 -> [w92]
    tunnel: w17 -> [w91]
    tunnel: [w90] -> w16
    tunnel: [w89] -> w15
    tunnel: w13 -> [w88]
    tunnel: w12 -> [w87]
    tunnel: [w86] -> w11
    tunnel: [w85] -> w10
    tunnel: [w79] -> w7
    tunnel: [w78] -> w8
    stop <- w113 stop-if-true
    # "ARDUINO LOOP"
    n13 = call <vilib>:"DIO Write.vi"("error in (no error)"=w87, "Input"="Green LED", "DIO Info In"=w88) -> ("error out"=w85:errorcluster, "DIO Info Out"=w86:T18)  [unwired: 7 in]
    n14 = call <vilib>:"DIO Write.vi"("error in (no error)"=w103, "DIO Info In"=w105) -> ("error out"=w102:errorcluster, "DIO Info Out"=w104:T18)  [unwired: 8 in]
    n15 = call <vilib>:"C DIO Read.vi"("error in (no error)"=w99, "DIO Info In in"=w100) -> ("error out"=w98:errorcluster, "IN"=→"TASK ENABLE":bool, "DIO Info In out"=w101:T18)  [unwired: 7 in]
    n16 = call <vilib>:"C DIO Read.vi"("error in (no error)"=w109, "DIO Info In in"=w111) -> ("error out"=w108:errorcluster, "IN"=w107:bool, "DIO Info In out"=w110:T18)  [unwired: 7 in]
    n17 = call <vilib>:"NavX Open.vi"("I2C Channel"=I2C_Channel."A") -> ("error out"=w94:errorcluster, "NavX Info"=w96:T23)  [unwired: 9 in]
    n18 = call "Digital Debounce Filter.vi"("Boolean input"=w107) -> ("Rising Edge"=→"Rising Edge":bool)  [unwired: 1 in, 2 out]
    n19 = call "Arduino Interfacing VI.vi"("AE Mode"=Arduino_Interfacing."Read From Arduino") -> ("error out"=w82:errorcluster, "Arduino Data"=w75:T4)  [unwired: 3 in]
    "Arduino Data" <- w75
    n20 = Unbundle By Name(w75) -> ("Rotary Switch"=→"Task selection":u8)
    n21 = call "navX reading VI.vi"("NavX Info In"=w96, "Mode"=navX_type_def."Get i2C reference", "error in (no error)"=w94) -> ("NavX Info Out"=w81:T23, "Error Out"=w80:errorcluster)  [unwired: 2 out]
    n22 = Merge Errors(w82, w94) -> (w73:errorcluster)
    "I2C Error" <- w73
    n23 = Unbundle By Name(w73) -> ("status"=w72:bool)
    n24 = Not(x=w72) -> (.not. x?=w71:bool)
    n25 = call <vilib>:"DIO Write.vi"("error in (no error)"=w91, "Input"=w71, "DIO Info In"=w92) -> ("error out"=w89:errorcluster, "DIO Info Out"=w90:T18)  [unwired: 7 in]
    n26 = call "navX reading VI.vi"("NavX Info In"=w81, "Mode"=navX_type_def."Read Values", "error in (no error)"=w80) -> ("NavX Info Out"=w79:T23, "NavX Readings"=→"NavX Readings":T3, "Error Out"=w78:errorcluster)  [unwired: 1 out]
    n27 = call "FGV Bool.vi"("Init/Read/Write State"=States_for_Action_Engine."Read") -> ("Output node"=w113:bool)  [unwired: 2 in, 1 out]
    n28 = Wait (ms)(milliseconds to wait=u32 50) -> ()  [unwired: 1 out]
  }
  n29 = while {
    tunnel: w61 -> [w131]
    tunnel: w62 -> [w130]
    tunnel: [w129] -> w68
    tunnel: [w128] -> w67
    tunnel: w66 -> [w127]
    tunnel: [w126] -> w64
    tunnel: w65 -> [w125]
    tunnel: [w124] -> w63
    stop <- w122 stop-if-true
    # "Generate USER Event Loop"
    n30 = local read "Rising Edge"() -> (w118:bool)
    n31 = Or(x="OK Button", y=w118) -> (x .or. y?=w117:bool)
    n32 = local read "TASK ENABLE"() -> (w116:bool)
    n33 = And(x=w117, y=w116) -> (x .and. y?=w115:bool)
    n34 = case shown="True" w115 {
      selector: w115 -> [_ w142]
      tunnel: w131 -> [w141 w146]
      tunnel: [w141 w145] -> w128
      tunnel: w127 -> [w140 w144]
      tunnel: [w140 w143] -> w126
      frame False {
      }
      frame True {
        n35 = Generate User Event(user event=w146, event data cluster=w142, error in=w144) -> (user event out=w145:refnum<user-event>, error out=w143:errorcluster)  [unwired: 1 in]
      }
    }
    n36 = case shown="False" "STOP" {
      selector: "STOP" -> [_ w135]
      tunnel: w130 -> [w134 w139]
      tunnel: [w134 w138] -> w129
      tunnel: w125 -> [w133 w137]
      tunnel: [w133 w136] -> w124
      tunnel: [FALSE w135] -> w122
      frame False {
      }
      frame True {
        n37 = Generate User Event(user event=w139, event data cluster=w135, error in=w137) -> (user event out=w138:refnum<user-event>, error out=w136:errorcluster)  [unwired: 1 in]
      }
    }
    n38 = call "FGV Bool.vi"("Init/Read/Write State"=States_for_Action_Engine."Write", "Input Node"=w122) -> ()  [unwired: 1 in, 2 out]
    n39 = call "Wait4"("Count(uSec)"=u32 20) -> ()  [unwired: 1 out]
  }
  n40 = while {
    tunnel: w60 -> [w153]
    tunnel: [w152] -> w59
    tunnel: w47 -> [w150]
    tunnel: [w149] -> w58
    tunnel: w53 -> [w148]
    tunnel: [w147] -> w50
    stop <- w151 stop-if-true
    # "EVENT Handling Loop"
    n41 = event shown="[1] <Start Task>: User Event" {
      selector: w153 -> [_ _ _]
      dyn-events: [_ _ _] -> w152
      timeout: _ -> [_ _ _]
      tunnel: [FALSE FALSE w183] -> w151
      tunnel: w150 -> [w158 w167 w181]
      tunnel: [w157 w166 w182] -> w149
      tunnel: w148 -> [w156 w165 w180]
      tunnel: [w155 w164 w179] -> w147
      event Timeout {
        n42 = event-data() -> ()  [unwired: 1 in, 3 out]
        n43 = Enqueue Element(queue=w158, element=Intruction_Type_Definitions."None" ("Enum"), error in (no error)=w156) -> (queue out=w157:refnum<queue>, error out=w155:errorcluster)  [unwired: 1 in, 1 out]
      }
      event User Event {
        n44 = event-data() -> ()  [unwired: 1 in, 5 out]
        n45 = call "Arduino Interfacing VI.vi"("AE Mode"=Arduino_Interfacing."Read From Arduino") -> ("Arduino Data"=w161:T4)  [unwired: 3 in, 1 out]
        n46 = Unbundle By Name(w161) -> ("Rotary Switch"=w160:u8)
        n47 = case shown="5" w160 {
          tunnel: [Intruction_Type_Definitions."None" ("Enum") Intruction_Type_Definitions."Start Task 1" ("Enum") Intruction_Type_Definitions."Start Task 2" ("Enum") Intruction_Type_Definitions."Start Task 3" ("Enum") Intruction_Type_Definitions."Start Task 4" ("Enum") Intruction_Type_Definitions."Start Task 5" ("Enum") Intruction_Type_Definitions."Start Task 6" ("Enum") Intruction_Type_Definitions."Start Task 8" ("Enum") Intruction_Type_Definitions."Start Task 9" ("Enum")] -> w163
          frame 0, Default {
          }
          frame 1 {
          }
          frame 2 {
          }
          frame 3 {
          }
          frame 4 {
          }
          frame 5 {
          }
          frame 6 {
          }
          frame 8 {
          }
          frame 9 {
          }
        }
        n48 = Enqueue Element(queue=w167, element=w163, error in (no error)=w165) -> (queue out=w166:refnum<queue>, error out=w164:errorcluster)  [unwired: 1 in, 1 out]
      }
      event User Event {
        n49 = event-data() -> ("Stop Queue"=w183:bool)  [unwired: 1 in, 4 out]
        n50 = Enqueue Element At Opposite End(queue=w181, element=Intruction_Type_Definitions."Exit" ("Enum"), error in (no error)=w180) -> (queue out=w182:refnum<queue>, error out=w179:errorcluster)  [unwired: 1 in, 1 out]
      }
    }
  }
  n51 = call "IMAQ Create"("Image Name"="Image dest") -> ("New Image"=w22:T25, "error out"=w21:errorcluster)  [unwired: 4 in]
  n52 = while {
    tunnel: w47 -> [w220]
    tunnel: w48 -> [w232]
    tunnel: w51 -> [w230]
    tunnel: [w229] -> _
    tunnel: [w228] -> w41
    shift-right: [w221] -> _
    shift-left: T16 {"PING_A"=0, "PING_B"=0, "PING_C"=0, "PING_D"=0} -> [w223]
    shift-right: [w214] -> _
    shift-left: State_Type_Definitions."Startup" ("Enum") -> [w217]
    shift-right: [w210] -> _
    shift-left: T17 {"xDistance"=0.0, "yDistance"=0.0, "wDistance"=0.0} -> [w212]
    shift-right: [w207] -> _
    shift-left: _ -> [w206]
    tunnel: w22 -> [w205]
    tunnel: w21 -> [w204]
    shift-right: [w201] -> _
    shift-left: T15 {"Recognized Object"=FALSE, "Object X coordinate"=0.0, "Object Y coordinate"=0.0} -> [w203]
    shift-right: [w198] -> _
    shift-left: T13 {"y Stepper Position"=0, "z Stepper Position"=0} -> [w200]
    shift-right: [w195] -> _
    shift-left: T12 {"Yaw"=0.0, "Compass"=0.0} -> [w197]
    shift-right: [w192] -> _
    shift-left: T11 {"Time up flag"=FALSE, "SET TIME TO CHECK"=0.0} -> [w194]
    shift-right: [w190] -> _
    shift-left: T10 {"yStepper desired"=0} -> [w191]
    shift-right: [w186] -> _
    shift-left: T9 {"Left IR Sensor"=0.0, "Arm IR Sensor"=0.0, "Bottom IR Sensor"=0.0} -> [w188]
    shift-right: [w184] -> _
    shift-left: T8 {"ySpeed"=0.0, "xSpeed"=0.0, "wSpeed"=0.0} -> [w185]
    stop <- w219 stop-if-true
    # ">>> Motor control cluster >>>"
    # ">>> yStepper command>>>"
    # ">>True Stop Next State >>"
    # ">>Error  >>"
    # ">>Timeout>>"
    # ">>Action states Queue Reference >>"
    # ">>State Logic Queue Reference >>"
    # "TOP LEVEL BASELINE (MAIN PROCESSING LOOP)"
    n53 = Dequeue Element(queue=w232, timeout in ms (-1)=0, error in (no error)=w230) -> (queue out=w224:refnum<queue>, element=w231:string, error out=w225:errorcluster)  [unwired: 1 out]
    "Action State" <- w231
    n54 = Wait (ms)(milliseconds to wait=u32 20) -> ()  [unwired: 1 out]
    n55 = case shown="\"CAM ACQ\"" w231 {
      tunnel: [_ _ _ _ _ _ _ _ _ _ _ _ _ _ _ _ _ _ _ 0 w1878 _ _ _ _ _ _ _ _ _ _ _ _ _ _ _ _ _ _ _ _ _ _ _ _ _ _] -> w227
      tunnel: w224 -> [_ _ _ _ _ _ _ _ _ _ _ _ _ _ _ _ _ _ _ _ _ _ _ _ _ _ _ _ _ _ _ _ _ _ _ _ _ _ _ _ _ _ _ _ _ _ _]
      tunnel: w223 -> [w1636 w1645 w1657 w1668 w1685 w1696 w1707 w1719 w1732 w1744 w1755 w1762 w1777 w1791 w1803 w1811 w1823 w1848 w1858 w1869 w1879 w1888 w1898 w1928 w1939 w1947 w1956 w1969 w1982 w1992 w2001 w2018 w2027 w2038 w2048 w2058 w2068 w2075 w2087 w2103 w2109 w2121 w2133 w2145 w2157 w2169 w2180]
      tunnel: [w1636 w1645 w1657 w1668 w1685 w1696 w1707 w1719 w1732 w1744 w1755 w1762 w1777 w1792 w1803 w1811 w1823 w1849 w1858 w1869 w1879 w1888 w1898 w1927 w1939 w1947 w1956 w1969 w1982 w1992 w2001 w2018 w2027 w2038 w2048 w2058 w2068 w2075 w2087 w2103 w2109 w2121 w2133 w2145 w2157 w2169 w2180] -> w222
      tunnel: [TRUE TRUE _ _ _ _ _ _ _ _ _ _ _ _ _ _ _ _ _ _ _ _ _ _ _ _ _ _ _ _ _ _ _ _ _ _ _ _ _ _ _ _ _ _ _ _ _] -> w219
      tunnel: w217 -> [w1634 w1643 w1656 w1667 w1684 w1695 w1706 w1718 w1731 w1743 w1754 w1761 w1776 w1790 w1802 w1809 w1822 w1847 w1857 w1866 w1876 w1887 w1897 w1926 w1938 w1946 w1955 w1968 w1981 w1991 w2000 w2017 w2026 w2037 w2047 w2057 w2067 w2074 w2086 w2102 w2108 w2120 w2132 w2144 w2156 w2168 w2179]
      tunnel: [_ _ _ _ _ _ _ _ _ _ _ _ _ _ _ _ _ _ _ _ TRUE _ _ _ _ _ _ _ _ _ _ _ _ _ _ _ _ _ _ _ _ _ _ _ _ _ _] -> w216
      tunnel: [w1634 w1643 w1656 w1667 w1684 w1695 w1706 w1718 w1731 w1743 w1754 w1761 w1776 w1790 w1802 w1809 w1822 w1847 w1857 w1866 w1876 w1887 w1897 w1926 w1938 w1946 w1955 w1968 w1981 w1991 w2000 w2017 w2026 w2037 w2047 w2057 w2067 w2074 w2086 w2102 w2108 w2120 w2132 w2144 w2156 w2168 w2179] -> w215
      tunnel: w212 -> [w1633 w1642 w1655 w1670 w1683 w1694 w1705 w1717 w1730 w1742 w1753 w1763 w1775 w1789 w1804 w1813 w1824 w1846 w1859 w1865 w1875 w1889 w1899 w1916 w1937 w1949 w1957 w1970 w1983 w1993 w2002 w2019 w2029 w2040 w2050 w2060 w2070 w2077 w2089 w2105 w2111 w2123 w2135 w2147 w2159 w2171 w2182]
      tunnel: [w1633 w1642 w1655 w1670 w1683 w1694 w1705 w1717 w1730 w1742 w1753 w1763 w1774 w1789 w1804 w1813 w1824 w1845 w1859 w1865 w1875 w1889 w1899 w1915 w1937 w1949 w1957 w1970 w1983 w1993 w2002 w2019 w2029 w2040 w2050 w2060 w2070 w2077 w2089 w2105 w2111 w2123 w2135 w2147 w2159 w2171 w2182] -> w211
      tunnel: w205 -> [w1628 _ _ _ _ _ _ _ _ _ _ _ _ _ _ _ _ _ _ _ _ _ _ _ _ _ _ _ _ _ _ w2013 _ _ _ _ _ _ _ _ _ _ _ _ _ _ _]
      tunnel: w204 -> [_ _ _ _ _ _ _ _ _ _ _ _ _ _ _ _ _ _ _ _ _ _ _ _ _ _ _ _ _ w1985 _ w2015 w2025 _ _ _ _ _ _ _ _ _ _ _ _ _ _]
      tunnel: w203 -> [w1632 w1641 w1654 w1669 w1682 w1693 w1704 w1716 w1729 w1741 w1751 w1760 w1773 w1788 w1797 w1812 w1821 w1837 w1856 w1864 w1874 w1886 w1896 w1921 w1935 w1948 w1954 w1967 w1980 w1987 w1999 w2010 w2028 w2039 w2049 w2059 w2069 w2076 w2088 w2104 w2110 w2122 w2134 w2146 w2158 w2170 w2181]
      tunnel: [w1632 w1641 w1654 w1669 w1682 w1693 w1704 w1716 w1729 w1741 w1751 w1760 w1773 w1788 w1797 w1812 w1821 w1836 w1856 w1864 w1874 w1886 w1896 w1920 w1935 w1948 w1954 w1967 w1980 w1987 w1999 w2009 w2028 w2039 w2049 w2059 w2069 w2076 w2088 w2104 w2110 w2122 w2134 w2146 w2158 w2170 w2181] -> w202
      tunnel: w200 -> [w1631 w1640 w1653 w1671 w1681 w1692 w1703 w1715 w1728 w1740 w1750 w1759 w1772 w1787 w1805 w1814 w1820 w1842 w1855 w1863 w1873 w1885 w1895 w1911 w1934 w1945 w1953 w1966 w1979 w1990 w1998 w2020 w2030 w2036 w2046 w2056 w2066 w2078 w2090 w2101 w2112 w2124 w2136 w2148 w2160 w2172 w2183]
      tunnel: [w1631 w1640 w1653 w1671 w1681 w1692 w1703 w1715 w1728 w1740 w1750 w1759 w1772 w1787 w1805 w1814 w1820 w1841 w1855 w1863 w1873 w1885 w1895 w1910 w1934 w1945 w1953 w1966 w1979 w1990 w1998 w2020 w2030 w2036 w2046 w2056 w2066 w2078 w2090 w2100 w2112 w2124 w2136 w2148 w2160 w2172 w2183] -> w199
      tunnel: w197 -> [w1630 w1639 w1651 w1672 w1679 w1690 w1702 w1713 w1726 w1738 w1749 w1758 w1771 w1780 w1800 w1815 w1819 w1832 w1854 w1862 w1872 w1884 w1894 w1907 w1933 w1942 w1952 w1965 w1978 w1989 w1997 w2021 w2031 w2035 w2043 w2053 w2063 w2079 w2091 w2095 w2113 w2125 w2137 w2149 w2161 w2173 w2184]
      tunnel: [w1630 w1639 w1651 w1672 w1679 w1690 w1702 w1713 w1726 w1738 w1749 w1758 w1771 w1780 w1799 w1815 w1819 w1831 w1854 w1862 w1872 w1884 w1894 w1906 w1933 w1942 w1952 w1965 w1978 w1989 w1997 w2021 w2031 w2035 w2043 w2053 w2063 w2079 w2091 w2095 w2113 w2125 w2137 w2149 w2161 w2173 w2184] -> w196
      tunnel: w194 -> [w1627 w1638 w1652 w1673 w1680 w1691 w1701 w1714 w1727 w1739 w1748 w1757 w1770 w1779 w1796 w1816 w1818 w1828 w1851 w1861 w1871 w1883 w1893 w1904 w1931 w1941 w1951 w1964 w1977 w1988 w1996 w2022 w2032 w2034 w2042 w2052 w2062 w2080 w2092 w2094 w2107 w2119 w2131 w2143 w2155 w2167 w2178]
      tunnel: [w1627 w1638 w1652 w1673 w1680 w1691 w1701 w1714 w1727 w1739 w1748 w1757 w1770 w1779 w1796 w1816 w1818 w1828 w1851 w1861 w1871 w1883 w1893 w1903 w1931 w1941 w1951 w1964 w1977 w1988 w1996 w2022 w2032 w2034 w2042 w2052 w2062 w2080 w2092 w2094 w2107 w2117 w2129 w2141 w2153 w2165 w2177] -> w193
      tunnel: w191 -> [_ _ _ _ _ _ _ _ _ _ _ _ _ _ _ _ _ _ _ _ _ _ _ _ _ _ _ _ _ _ _ _ _ _ _ _ _ _ w2083 _ _ _ _ _ _ _ _]
      tunnel: [w1626 w1637 w1646 w1663 w1674 w1686 w1697 w1708 w1722 w1733 w1745 w1756 w1764 w1778 w1793 w1807 w1817 w1825 w1850 w1860 w1870 w1882 w1890 w1900 w1930 w1940 w1950 w1958 w1971 w1984 w1994 w2003 w2023 w2033 w2041 w2051 w2061 w2071 w2081 w2093 w2106 w2114 w2126 w2138 w2150 w2162 w2174] -> w187
      tunnel: w188 -> [w1626 w1637 w1646 w1663 w1674 w1686 w1697 w1708 w1722 w1733 w1745 w1756 w1764 w1778 w1793 w1808 w1817 w1825 w1850 w1860 w1870 w1882 w1890 w1900 w1930 w1940 w1950 w1958 w1971 w1984 w1994 w2003 w2023 w2033 w2041 w2051 w2061 w2071 w2081 w2093 w2106 w2114 w2126 w2138 w2150 w2162 w2174]
      tunnel: w185 -> [_ _ _ _ _ _ _ _ w1721 _ _ _ _ _ _ _ _ _ _ _ _ _ _ _ _ _ _ _ _ _ _ _ _ _ _ _ _ _ _ _ _ _ _ _ _ _ _]
      frame "Exit" {
        # ">>State Logic  >>"
        # ">>> Time cluster >>>"
        # ">>> Yaw >>>"
        # ">>> Stepper position >>>"
        # ">>> Encoders >>>"
        # ">>> Object detection >>>"
        # ">>> Ultrasonic Sensors Detect >>>"
        n56 = call "Imaq Dispose"("All Images? (No)"=TRUE, "Image"=w1628) -> ()  [unwired: 4 in, 1 out]
      }
      frame "----Movement States----" {
        # ">>State Logic  >>"
        # ">>> Time cluster >>>"
        # ">>> Yaw >>>"
        # ">>> Stepper position >>>"
        # ">>> Encoders >>>"
        # ">>> Object detection >>>"
        # ">>> Ultrasonic Sensors Detect >>>"
      }
      frame "FORWARD" {
        # ">>State Logic  >>"
        # ">>> Time cluster >>>"
        # ">>> Yaw >>>"
        # ">>> Stepper position >>>"
        # ">>> Encoders >>>"
        # ">>> Object detection >>>"
        # ">>> Ultrasonic Sensors Detect >>>"
        n57 = Unbundle By Name(w1651) -> ("Yaw"=w1647:dbl)
        n58 = call "MOTOR CONTROL WITH PID AE.vi"("Yaw"=w1647, "Speed"=50.0, "Direction"=MOTOR_CONTROL_WITH_PID_AE_DIRECTION_TYPE_DEF."y-axis movement", "AE Mode"=MOTOR_CONTROL_WITH_PID_AE_DATA_MODE_TYPE_DEF."Write to AE") -> ()  [unwired: 1 out]
      }
      frame "FORWARD - IR ASSIST" {
        # ">>State Logic  >>"
        # ">>> Time cluster >>>"
        # ">>> Yaw >>>"
        # ">>> Stepper position >>>"
        # ">>> Encoders >>>"
        # ">>> Object detection >>>"
        # ">>> Ultrasonic Sensors Detect >>>"
        n59 = Unbundle By Name(w1663) -> ("Left IR Sensor"=w1662:dbl)
        n60 = Subtract(x=w1662, y=15.0) -> (x-y=w1660:dbl)
        n61 = Multiply(x=w1660, y=0.5) -> (x*y=w1658:dbl)
        n62 = call "MOTOR CONTROL WITH PID AE.vi"("Yaw"=w1658, "Speed"=30.0, "Direction"=MOTOR_CONTROL_WITH_PID_AE_DIRECTION_TYPE_DEF."y-axis movement", "AE Mode"=MOTOR_CONTROL_WITH_PID_AE_DATA_MODE_TYPE_DEF."Write to AE") -> ()  [unwired: 1 out]
      }
      frame "LEFT" {
        # ">>State Logic  >>"
        # ">>> Time cluster >>>"
        # ">>> Yaw >>>"
        # ">>> Stepper position >>>"
        # ">>> Encoders >>>"
        # ">>> Object detection >>>"
        # ">>> Ultrasonic Sensors Detect >>>"
        n63 = Unbundle By Name(w1679) -> ("Yaw"=w1676:dbl)
        n64 = call "MOTOR CONTROL WITH PID AE.vi"("Yaw"=w1676, "Speed"=-25.0, "Direction"=MOTOR_CONTROL_WITH_PID_AE_DIRECTION_TYPE_DEF."x-axis movement", "AE Mode"=MOTOR_CONTROL_WITH_PID_AE_DATA_MODE_TYPE_DEF."Write to AE") -> ()  [unwired: 1 out]
      }
      frame "R-ACW" {
        # ">>> IR Sensors >>>"
        # ">>> Time cluster >>>"
        # ">>> Yaw >>>"
        # ">>> Stepper position >>>"
        # ">>> Encoders >>>"
        # ">>> Object detection >>>"
        # ">>> Ultrasonic Sensors Detect >>>"
        n65 = call "MOTOR CONTROL WITH PID AE.vi"("Speed"=-10.0, "Direction"=MOTOR_CONTROL_WITH_PID_AE_DIRECTION_TYPE_DEF."rotation", "AE Mode"=MOTOR_CONTROL_WITH_PID_AE_DATA_MODE_TYPE_DEF."Write to AE") -> ()  [unwired: 1 in, 1 out]
      }
      frame "R-CW" {
        (unwired) -0.2 ("Speed")
        # ">>> Time cluster >>>"
        # ">>> Yaw >>>"
        # ">>> Stepper position >>>"
        # ">>> Encoders >>>"
        # ">>> Object detection >>>"
        # ">>> Ultrasonic Sensors Detect >>>"
        n66 = call "MOTOR CONTROL WITH PID AE.vi"("Speed"=10.0, "Direction"=MOTOR_CONTROL_WITH_PID_AE_DIRECTION_TYPE_DEF."rotation", "AE Mode"=MOTOR_CONTROL_WITH_PID_AE_DATA_MODE_TYPE_DEF."Write to AE") -> ()  [unwired: 1 in, 1 out]
      }
      frame "RIGHT" {
        # ">>> Time cluster >>>"
        # ">>> Yaw >>>"
        # ">>> Stepper position >>>"
        # ">>> Encoders >>>"
        # ">>> Object detection >>>"
        # ">>> Ultrasonic Sensors Detect >>>"
        n67 = Unbundle By Name(w1713) -> ("Yaw"=w1709:dbl)
        n68 = call "MOTOR CONTROL WITH PID AE.vi"("Yaw"=w1709, "Speed"=50.0, "Direction"=MOTOR_CONTROL_WITH_PID_AE_DIRECTION_TYPE_DEF."x-axis movement", "AE Mode"=MOTOR_CONTROL_WITH_PID_AE_DATA_MODE_TYPE_DEF."Write to AE") -> ()  [unwired: 1 out]
      }
      frame "X AXIS - SLOW" {
        # ">>> IR Sensors >>>"
        # ">>> Time cluster >>>"
        # ">>> Yaw >>>"
        # ">>> Stepper position >>>"
        # ">>> Encoders >>>"
        # ">>> Object detection >>>"
        # ">>> Ultrasonic Sensors Detect >>>"
        n69 = Unbundle By Name(w1721) -> ("xSpeed"=w1720:dbl)
        n70 = Unbundle By Name(w1726) -> ("Yaw"=w1723:dbl)
        n71 = call "MOTOR CONTROL WITH PID AE.vi"("Yaw"=w1723, "Speed"=w1720, "Direction"=MOTOR_CONTROL_WITH_PID_AE_DIRECTION_TYPE_DEF."x-axis movement", "AE Mode"=MOTOR_CONTROL_WITH_PID_AE_DATA_MODE_TYPE_DEF."Write to AE") -> ()  [unwired: 1 out]
      }
      frame "REVERSE" {
        # ">>> Time cluster >>>"
        # ">>> Yaw >>>"
        # ">>> Stepper position >>>"
        # ">>> Encoders >>>"
        # ">>> Object detection >>>"
        # ">>> Ultrasonic Sensors Detect >>>"
        n72 = Unbundle By Name(w1738) -> ("Yaw"=w1734:dbl)
        n73 = call "MOTOR CONTROL WITH PID AE.vi"("Yaw"=w1734, "Speed"=-50.0, "Direction"=MOTOR_CONTROL_WITH_PID_AE_DIRECTION_TYPE_DEF."y-axis movement", "AE Mode"=MOTOR_CONTROL_WITH_PID_AE_DATA_MODE_TYPE_DEF."Write to AE") -> ()  [unwired: 1 out]
      }
      frame "STOP" {
        n74 = Wait (ms)(milliseconds to wait=u32 100) -> ()  [unwired: 1 out]
        n75 = call "MOTOR CONTROL WITH PID AE.vi"("Direction"=MOTOR_CONTROL_WITH_PID_AE_DIRECTION_TYPE_DEF."stop", "AE Mode"=MOTOR_CONTROL_WITH_PID_AE_DATA_MODE_TYPE_DEF."Write to AE") -> ()  [unwired: 2 in, 1 out]
      }
      frame "----SENSOR READING---- " {
      }
      frame "READ ENCODERS" {
        # ">>> Time cluster >>>"
        # ">>> Yaw >>>"
        # ">>> Stepper position >>>"
        # ">>> Object detection >>>"
        # ">>> Current encoder distance >>>"
        # ">>> Ultrasonic Sensors Detect >>>"
        n76 = call "MOTOR CONTROL WITH PID AE.vi"("AE Mode"=MOTOR_CONTROL_WITH_PID_AE_DATA_MODE_TYPE_DEF."Read from AE") -> ("Speed & distance"=w1768:T1)  [unwired: 3 in]
        n77 = Unbundle By Name(w1768) -> ("xDistance"=w1767:dbl, "yDistance"=w1766:dbl, "wDistance"=w1765:dbl)
        n78 = Bundle By Name(cluster=w1775, "xDistance"=w1767, "yDistance"=w1766, "wDistance"=w1765) -> (w1774:T17)
      }
      frame "READ ULTRASONIC" {
        (unwired) navX_type_def."Read Values" ("Mode")
        (unwired) MOTOR_CONTROL_NO_PID_Type_Def."Latch" ("Direction")
        # ">>State Logic  >>"
        # ">>> Time cluster >>>"
        # ">>> Ultrasonic Sensors Detect >>>"
        # ">>> Object detection >>>"
        # ">>> Encoders >>>"
        # ">>> Stepper position >>>"
        # ">>> Yaw >>>"
        n79 = call "Arduino Interfacing VI.vi"("AE Mode"=Arduino_Interfacing."Read From Arduino") -> ("Arduino Data"=w1785:T4)  [unwired: 3 in, 1 out]
        n80 = Unbundle By Name(w1785) -> ("PING A"=w1784:u8, "PING B"=w1783:u8, "PING C"=w1782:u8, "PING D"=w1781:u8)
        n81 = Bundle By Name(cluster=w1791, "PING_A"=w1784, "PING_B"=w1783, "PING_C"=w1782, "PING_D"=w1781) -> (w1792:T16)
      }
      frame "READ NAVX" {
        # ">>> Time cluster >>>"
        # ">>> Yaw >>>"
        # ">>> Ultrasonic Sensors Detect >>>"
        # ">>> Object detection >>>"
        # ">>> Encoders >>>"
        # ">>> Stepper position >>>"
        n82 = call "navX reading VI.vi"("Mode"=navX_type_def."Read Values") -> ("NavX Readings"=w1795:T3)  [unwired: 2 in, 3 out]
        n83 = Unbundle By Name(w1795) -> ("Heading"=w1794:dbl)
        n84 = Unbundle By Name(w1795) -> ("Yaw"=w1798:dbl)
        n85 = Bundle By Name(cluster=w1800, "Yaw"=w1798, "Compass"=w1794) -> (w1799:T12)
      }
      frame "READ IR" {
        w1810 = T35 [enum."A/AI0"] items=["Not Connected", "AudioIn/Left", "AudioIn/Right", "C/AI0", "C/AI1", "A/AI0", "A/AI1", "A/AI2", "A/AI3", "A/AI4", "A/AI5", "A/AI6", "A/AI7", "B/AI0", "B/AI1", "B/AI2", "B/AI3", "B/AI4", "B/AI5", "B/AI6", "B/AI7", "AI/AI0", "AI/AI1", "AI/AI2", "AI/AI3", "A/AI0 (DIFF)", "A/AI1 (DIFF)", "A/AI2 (DIFF)", "A/AI3 (DIFF)", "B/AI0 (DIFF)", "B/AI1 (DIFF)", "B/AI2 (DIFF)", "B/AI3 (DIFF)"] ("AI Channel")
        # ">>State Logic  >>"
        # ">>> Time cluster >>>"
        # ">>> Ultrasonic Sensors Detect >>>"
        # ">>> Object detection >>>"
        # ">>> Encoders >>>"
        # ">>> Stepper position >>>"
        # ">>> Yaw >>>"
        n86 = call <vilib>:"Sharp IR.vi"("AI Channel"=w1810) -> ("Sharp IR Distance"=w1806:dbl)  [unwired: 8 in, 2 out]
        n87 = Bundle By Name(cluster=w1808, "Left IR Sensor"=w1806) -> (w1807:T9)
      }
      frame "----SYSTEM MODES----" {
        (unwired) I2C_MASTER_Type_Def."Last State" ("Arduino Mode")
        # ">>> Object detection >>>"
        # ">>> Yaw >>>"
        # ">>> Ultrasonic Sensors Detect >>>"
        # ">>> Encoders >>>"
        # ">>> Stepper position >>>"
      }
      frame "INIT" {
        w1843 = u8 0
        w1844 = 0.0
        # ">>> Time cluster >>>"
        # ">>> Object detection >>>"
        # ">>> Yaw >>>"
        # ">>> Ultrasonic Sensors Detect >>>"
        # ">>> Encoders >>>"
        # ">>> Stepper position >>>"
        # ">>State Logic  >>"
        n88 = call "Arduino Interfacing VI.vi"("AE Mode"=Arduino_Interfacing."Initialize") -> ()  [unwired: 3 in, 2 out]
        n89 = call "FGV Bool.vi"("Init/Read/Write State"=States_for_Action_Engine."Initialize") -> ()  [unwired: 2 in, 2 out]
        n90 = call "Elasped Timer.vi"("Action"=Elapsed_timer_control."Initialize") -> ()  [unwired: 7 in, 4 out]
        n91 = call "MOTOR CONTROL WITH PID AE.vi"("AE Mode"=MOTOR_CONTROL_WITH_PID_AE_DATA_MODE_TYPE_DEF."Init AE") -> ()  [unwired: 3 in, 1 out]
        n92 = Bundle By Name(cluster=w1837, "Recognized Object"=FALSE, "Object X coordinate"=0.0, "Object Y coordinate"=0.0) -> (w1836:T15)
        n93 = Bundle By Name(cluster=w1842, "y Stepper Position"=u8 0, "z Stepper Position"=u8 0) -> (w1841:T13)
        n94 = Bundle By Name(cluster=w1846, "xDistance"=w1844, "yDistance"=w1844, "wDistance"=w1844) -> (w1845:T17)
        n95 = Bundle By Name(cluster=w1848, "PING_A"=w1843, "PING_B"=w1843, "PING_C"=w1843, "PING_D"=w1843) -> (w1849:T16)
        n96 = Bundle By Name(cluster=w1832, "Yaw"=0.0) -> (w1831:T12)
      }
      frame "ARDUINO - ULTRASONIC" {
        # ">>> Object detection >>>"
        # ">>> Yaw >>>"
        # ">>> Ultrasonic Sensors Detect >>>"
        # ">>> Encoders >>>"
        # ">>> Stepper position >>>"
        # ">>State Logic  >>"
        n97 = call "Arduino Interfacing VI.vi"("Data to Write"=I2C_MASTER_WRITE_NEW_Type_Def."Ultrasonic sensors", "AE Mode"=Arduino_Interfacing."Write to Arduino") -> ()  [unwired: 2 in, 2 out]
      }
      frame "NAVX CALIBRATE" {
        # ">>> Object detection >>>"
        # ">>> Yaw >>>"
        # ">>> Ultrasonic Sensors Detect >>>"
        # ">>> Encoders >>>"
        # ">>> Stepper position >>>"
        # ">>State Logic  >>"
        # "Adds a 15 second delay to the startup process \nfor the NavX to calibrate"
        n98 = Wait (ms)(milliseconds to wait=u32 1000) -> ()  [unwired: 1 out]
      }
      frame "NO ACTION", Default {
        (unwired) u8 0 ("y Stepper value")
        (unwired) TRUE ("Latch")
        (unwired) navX_type_def."Read Values" ("Mode")
        (unwired) MOTOR_CONTROL_NO_PID_Type_Def."Latch" ("Direction")
        # ">>> Object detection >>>"
        # ">>> Yaw >>>"
        # ">>> Ultrasonic Sensors Detect >>>"
        # ">>> Encoders >>>"
        # ">>> Stepper position >>>"
        # ">>State Logic  >>"
        n99 = case shown="4" w1876 {
          tunnel: [0 100] -> w1878
          frame 1, Default {
          }
          frame 4 {
          }
        }
      }
      frame "----RESET CASES----" {
        (unwired) I2C_MASTER_Type_Def."Last State" ("Arduino Mode")
        # ">>> Object detection >>>"
        # ">>> Yaw >>>"
        # ">>> Ultrasonic Sensors Detect >>>"
        # ">>> Encoders >>>"
        # ">>> Stepper position >>>"
        # ">>State Logic  >>"
      }
      frame "RESET ENCODERS" {
        # ">>> Object detection >>>"
        # ">>> Yaw >>>"
        # ">>> Ultrasonic Sensors Detect >>>"
        # ">>> Encoders >>>"
        # ">>> Stepper position >>>"
        # ">>State Logic  >>"
        n100 = call "MOTOR CONTROL WITH PID AE.vi"("Direction"=MOTOR_CONTROL_WITH_PID_AE_DIRECTION_TYPE_DEF."reset encoders", "AE Mode"=MOTOR_CONTROL_WITH_PID_AE_DATA_MODE_TYPE_DEF."Write to AE") -> ()  [unwired: 2 in, 1 out]
      }
      frame "RESET FLAGS" {
        (unwired) I2C_MASTER_Type_Def."Last State" ("Arduino Mode")
        # "Resets any software variables\nand/or non-critical states"
        n101 = Wait (ms)(milliseconds to wait=u32 20) -> ()  [unwired: 1 out]
        n102 = Bundle By Name(cluster=w1904, "Time up flag"=FALSE, "SET TIME TO CHECK"=0.0) -> (w1903:T11)
        n103 = Bundle By Name(cluster=w1921, "Recognized Object"=FALSE, "Object X coordinate"=0.0, "Object Y coordinate"=0.0) -> (w1920:T15)
        n104 = Bundle By Name(cluster=w1911, "y Stepper Position"=u8 0, "z Stepper Position"=u8 0) -> (w1910:T13)
        n105 = Bundle By Name(cluster=w1916, "xDistance"=0.0, "yDistance"=0.0, "wDistance"=0.0) -> (w1915:T17)
        n106 = Bundle By Name(cluster=w1928, "PING_A"=u8 0, "PING_B"=u8 0, "PING_C"=u8 0, "PING_D"=u8 0) -> (w1927:T16)
        n107 = Bundle By Name(cluster=w1907, "Yaw"=0.0) -> (w1906:T12)
      }
      frame "RESET YAW" {
        n108 = Wait (ms)(milliseconds to wait=u32 100) -> ()  [unwired: 1 out]
        n109 = call "navX reading VI.vi"("Mode"=navX_type_def."Zero Yaw") -> ()  [unwired: 2 in, 4 out]
      }
      frame "RESET ARM" {
        n110 = call "Arduino Interfacing VI.vi"("Data to Write"=I2C_MASTER_WRITE_NEW_Type_Def."Soft Reset", "AE Mode"=Arduino_Interfacing."Write to Arduino") -> ()  [unwired: 2 in, 2 out]
      }
      frame "--------CAM STATES-------" {
      }
      frame "OPEN LOG CAM" {
        n111 = call "Webcam AE.vi"("Session In"=T32 "cam0", "Camera states"=Webcam_AE."Initialize Camera") -> ("error out"=w1961:errorcluster, "Session Out"=w1960:T32)  [unwired: 1 in, 1 out]
        n112 = call "Webcam AE.vi"("error in (no error)"=w1961, "Session In"=w1960, "Camera states"=Webcam_AE."Open Camera") -> ()  [unwired: 3 out]
      }
      frame "OPEN LIFE CAM" {
        n113 = call "Webcam AE.vi"("Session In"=T32 "cam1", "Camera states"=Webcam_AE."Initialize Camera") -> ("error out"=w1974:errorcluster, "Session Out"=w1973:T32)  [unwired: 1 in, 1 out]
        n114 = call "Webcam AE.vi"("error in (no error)"=w1974, "Session In"=w1973, "Camera states"=Webcam_AE."Open Camera") -> ()  [unwired: 3 out]
      }
      frame "CAM ACQ" {
        # ">>State Logic  >>"
        # ">>> Time cluster >>>"
        # ">>> Yaw >>>"
        # ">>> Stepper position >>>"
        # ">>> Encoders >>>"
        # ">>> Object detection >>>"
        # ">>> Ultrasonic Sensors Detect >>>"
        n115 = call "Webcam AE.vi"("error in (no error)"=w1985, "Camera states"=Webcam_AE."Continuous Acquisition") -> ()  [unwired: 1 in, 3 out]
      }
      frame "CAM CLOSE" {
        # ">>State Logic  >>"
        # ">>> Time cluster >>>"
        # ">>> Yaw >>>"
        # ">>> Stepper position >>>"
        # ">>> Encoders >>>"
        # ">>> Object detection >>>"
        # ">>> Ultrasonic Sensors Detect >>>"
        n116 = call "Webcam AE.vi"("Camera states"=Webcam_AE."Close Camera") -> ()  [unwired: 2 in, 3 out]
      }
      frame "PROCESS IMAGE" {
        # ">>State Logic  >>"
        # ">>> Time cluster >>>"
        # ">>> Yaw >>>"
        # ">>> Stepper position >>>"
        # ">>> Encoders >>>"
        # ">>> Object detection >>>"
        # ">>> Ultrasonic Sensors Detect >>>"
        n117 = call "Webcam AE.vi"("error in (no error)"=w2015, "Camera states"=Webcam_AE."Retrieve Image") -> ("error out"=w2011:errorcluster, "Image Out"=w2014:T25)  [unwired: 1 in, 1 out]
        n118 = call "Object Detection SubVI.vi"("Error In"=w2011, "Mode"="Object recognition mode", "Image Dest"=w2013, "Image in"=w2014) -> ("Object Center Coordinates"=w2008:cluster{"x":sgl, "y":sgl}, "Object detection cluster"=w2004:T2)  [unwired: 2 out]
        "Object detection cluster" <- w2004
        "Object Center Coordinates" <- w2008
        n119 = Unbundle By Name(w2004) -> ("Object detected?"=w2005:bool)
        n120 = Unbundle By Name(w2008) -> ("x"=w2007:sgl, "y"=w2006:sgl)
        n121 = Bundle By Name(cluster=w2010, "Recognized Object"=w2005, "Object X coordinate"=w2007, "Object Y coordinate"=w2006) -> (w2009:T15)
      }
      frame "DISPOSE BUFFERS" {
        # ">>State Logic  >>"
        # ">>> Time cluster >>>"
        # ">>> Yaw >>>"
        # ">>> Stepper position >>>"
        # ">>> Encoders >>>"
        # ">>> Object detection >>>"
        # ">>> Ultrasonic Sensors Detect >>>"
        n122 = call "Webcam AE.vi"("error in (no error)"=w2025, "Camera states"=Webcam_AE."Dispose Image Buffers") -> ()  [unwired: 1 in, 3 out]
      }
      frame "-----ARM ACTIONS-----" {
      }
      frame "CLOSE CLAW" {
        n123 = call "Arduino Interfacing VI.vi"("Data to Write"=I2C_MASTER_WRITE_NEW_Type_Def."Close Claw", "AE Mode"=Arduino_Interfacing."Write to Arduino") -> ()  [unwired: 2 in, 2 out]
      }
      frame "OPEN CLAW" {
        n124 = call "Arduino Interfacing VI.vi"("Data to Write"=I2C_MASTER_WRITE_NEW_Type_Def."Open Claw", "AE Mode"=Arduino_Interfacing."Write to Arduino") -> ()  [unwired: 2 in, 2 out]
      }
      frame "Z STEPPER CAM HEIGHT" {
        n125 = call "Arduino Interfacing VI.vi"("Data to Write"=I2C_MASTER_WRITE_NEW_Type_Def."zStepper 6k", "AE Mode"=Arduino_Interfacing."Write to Arduino") -> ()  [unwired: 2 in, 2 out]
      }
      frame "Z STEPPER GRAB HEIGHT" {
        # ">>State Logic  >>"
        # ">>> Time cluster >>>"
        # ">>> Yaw >>>"
        # ">>> Stepper position >>>"
        # ">>> Encoders >>>"
        # ">>> Object detection >>>"
        # ">>> Ultrasonic Sensors Detect >>>"
        n126 = call "Arduino Interfacing VI.vi"("Data to Write"=I2C_MASTER_WRITE_NEW_Type_Def."zStepper 100", "AE Mode"=Arduino_Interfacing."Write to Arduino") -> ()  [unwired: 2 in, 2 out]
      }
      frame "Y STEPPER CONTROL" {
        # ">>State Logic  >>"
        # ">>> yStepper command>>>"
        # ">>> Time cluster >>>"
        # ">>> Yaw >>>"
        # ">>> Stepper position >>>"
        # ">>> Encoders >>>"
        # ">>> Object detection >>>"
        # ">>> Ultrasonic Sensors Detect >>>"
        n127 = Unbundle By Name(w2083) -> ("yStepper desired"=w2082:u8)
        n128 = call "Arduino Interfacing VI.vi"("y Stepper value"=w2082, "Data to Write"=I2C_MASTER_WRITE_NEW_Type_Def."yStepper control", "AE Mode"=Arduino_Interfacing."Write to Arduino") -> ()  [unwired: 1 in, 2 out]
      }
      frame "READ STEPPER VALUES" {
        # ">>State Logic  >>"
        # ">>> Time cluster >>>"
        # ">>> Yaw >>>"
        # ">>> Stepper position >>>"
        # ">>> Encoders >>>"
        # ">>> Object detection >>>"
        # ">>> Ultrasonic Sensors Detect >>>"
        n129 = call "Arduino Interfacing VI.vi"("AE Mode"=Arduino_Interfacing."Read From Arduino") -> ("Arduino Data"=w2098:T4)  [unwired: 3 in, 1 out]
        n130 = Unbundle By Name(w2098) -> ("y Stepper Position"=w2097:u8, "z Stepper Position"=w2096:u8)
        n131 = Bundle By Name(cluster=w2101, "y Stepper Position"=w2097, "z Stepper Position"=w2096) -> (w2100:T13)
      }
      frame " -----TIMING-----" {
        # ">>State Logic  >>"
        # ">>> Time cluster >>>"
        # ">>> Yaw >>>"
        # ">>> Stepper position >>>"
        # ">>> Encoders >>>"
        # ">>> Object detection >>>"
        # ">>> Ultrasonic Sensors Detect >>>"
      }
      frame "SET TIMER 1" {
        # ">>State Logic  >>"
        # ">>> Time cluster >>>"
        # ">>> Yaw >>>"
        # ">>> Stepper position >>>"
        # ">>> Encoders >>>"
        # ">>> Object detection >>>"
        # ">>> Ultrasonic Sensors Detect >>>"
        n132 = call "Elasped Timer.vi"("Time Setting"=1.0, "Action"=Elapsed_timer_control."Initialize") -> ()  [unwired: 6 in, 4 out]
        n133 = Bundle By Name(cluster=w2119, "Time up flag"=FALSE) -> (w2117:T11)
      }
      frame "SET TIMER 2" {
        # ">>State Logic  >>"
        # ">>> Time cluster >>>"
        # ">>> Yaw >>>"
        # ">>> Stepper position >>>"
        # ">>> Encoders >>>"
        # ">>> Object detection >>>"
        # ">>> Ultrasonic Sensors Detect >>>"
        n134 = call "Elasped Timer.vi"("Time Setting"=2.0, "Action"=Elapsed_timer_control."Initialize") -> ()  [unwired: 6 in, 4 out]
        n135 = Bundle By Name(cluster=w2131, "Time up flag"=FALSE) -> (w2129:T11)
      }
      frame "SET TIMER 3" {
        # ">>State Logic  >>"
        # ">>> Time cluster >>>"
        # ">>> Yaw >>>"
        # ">>> Stepper position >>>"
        # ">>> Encoders >>>"
        # ">>> Object detection >>>"
        # ">>> Ultrasonic Sensors Detect >>>"
        n136 = call "Elasped Timer.vi"("Time Setting"=3.0, "Action"=Elapsed_timer_control."Initialize") -> ()  [unwired: 6 in, 4 out]
        n137 = Bundle By Name(cluster=w2143, "Time up flag"=FALSE) -> (w2141:T11)
      }
      frame "SET TIMER 4" {
        # ">>State Logic  >>"
        # ">>> Time cluster >>>"
        # ">>> Yaw >>>"
        # ">>> Stepper position >>>"
        # ">>> Encoders >>>"
        # ">>> Object detection >>>"
        # ">>> Ultrasonic Sensors Detect >>>"
        n138 = call "Elasped Timer.vi"("Time Setting"=4.0, "Action"=Elapsed_timer_control."Initialize") -> ()  [unwired: 6 in, 4 out]
        n139 = Bundle By Name(cluster=w2155, "Time up flag"=FALSE) -> (w2153:T11)
      }
      frame "SET TIMER 5" {
        # ">>State Logic  >>"
        # ">>> Time cluster >>>"
        # ">>> Yaw >>>"
        # ">>> Stepper position >>>"
        # ">>> Encoders >>>"
        # ">>> Object detection >>>"
        # ">>> Ultrasonic Sensors Detect >>>"
        n140 = call "Elasped Timer.vi"("Time Setting"=5.0, "Action"=Elapsed_timer_control."Initialize") -> ()  [unwired: 6 in, 4 out]
        n141 = Bundle By Name(cluster=w2167, "Time up flag"=FALSE) -> (w2165:T11)
      }
      frame "START TIMER" {
        # ">>State Logic  >>"
        # ">>> Time cluster >>>"
        # ">>> Yaw >>>"
        # ">>> Stepper position >>>"
        # ">>> Encoders >>>"
        # ">>> Object detection >>>"
        # ">>> Ultrasonic Sensors Detect >>>"
        n142 = call "Elasped Timer.vi"("Action"=Elapsed_timer_control."Start") -> ("Time Out?!"=w2175:bool)  [unwired: 7 in, 3 out]
        n143 = Bundle By Name(cluster=w2178, "Time up flag"=w2175) -> (w2177:T11)
      }
    }
    "State Logic" <- w215
    n144 = local read "TASK ENABLE"() -> (w209:bool)
    n145 = Not(x=w209) -> (.not. x?=w208:bool)
    n146 = case shown="True" w216 {
      tunnel: w220 -> [w245 w280]
      tunnel: w224 -> [w241 w282]
      tunnel: [w245 w280] -> w229
      tunnel: [w241 w283] -> w228
      tunnel: w225 -> [_ w278]
      tunnel: w227 -> [_ w279]
      tunnel: w222 -> [w244 w285]
      tunnel: [w244 w285] -> w221
      tunnel: "STOP TASK" -> [_ w268]
      tunnel: w215 -> [w243 w284]
      tunnel: [w243 w281] -> w214
      tunnel: w211 -> [w242 w274]
      tunnel: [w242 w274] -> w210
      tunnel: w208 -> [_ w269]
      tunnel: [w240 w266] -> w207
      tunnel: w206 -> [w240 w265]
      tunnel: w202 -> [w239 w262]
      tunnel: [w239 w262] -> w201
      tunnel: w199 -> [w238 w258]
      tunnel: [w238 w258] -> w198
      tunnel: w196 -> [w237 w256]
      tunnel: [w237 w256] -> w195
      tunnel: w193 -> [w236 w254]
      tunnel: [w236 w254] -> w192
      tunnel: w191 -> [w235 w253]
      tunnel: [w235 w252] -> w190
      tunnel: [_ w250] -> w189
      tunnel: w187 -> [w234 w248]
      tunnel: [w234 w248] -> w186
      tunnel: w185 -> [w233 w247]
      tunnel: [w233 w246] -> w184
      frame False {
        # ">>> Motor control cluster >>>"
        # ">>> yStepper command>>>"
        # ">>> Motor control cluster >>>"
        # ">>> yStepper command>>>"
        # ">>> Motor control cluster >>>"
        # ">>> IR Sensors >>>"
        # ">>> IR Sensors >>>"
        # ">>> yStepper command>>>"
        # ">>> Time cluster >>>"
        # ">>> Yaw >>>"
        # ">>> Stepper position >>>"
        # ">>> Encoders >>>"
        # ">>> Object detection >>>"
        # ">>> Ultrasonic Sensors Detect >>>"
        # ">>> Time cluster >>>"
        # ">>> Yaw >>>"
        # ">>> Stepper position >>>"
        # ">>> Encoders >>>"
        # ">>> Object detection >>>"
        # ">>> Ultrasonic Sensors Detect >>>"
      }
      frame True {
        # ">>> Motor control cluster >>>"
        # ">>> yStepper command>>>"
        # ">>> IR Sensors >>>"
        # ">>> Motor control cluster >>>"
        # ">>State Logic Queue Reference >>"
        # ">>Timeout>>"
        # ">>> yStepper command>>>"
        # ">>> Time cluster >>>"
        # ">>> Object detection >>>"
        # ">>> Yaw >>>"
        # ">>> Ultrasonic Sensors Detect >>>"
        # ">>> Encoders >>>"
        # ">>> Stepper position >>>"
        # ">>State Logic  >>"
        # ">>True Stop Next State >>"
        # ">>Action Queue>>"
        # ">> Manual override >>"
        # ">>> Time cluster >>>"
        # ">>> Yaw >>>"
        # ">>> Stepper position >>>"
        # ">>> Encoders >>>"
        # ">>> Object detection >>>"
        # ">>> Ultrasonic Sensors Detect >>>"
        # ">>Action Queue>>"
        # ">>State Logic Queue Reference >>"
        n147 = Or(x=w268, y=w269) -> (x .or. y?=w267:bool)
        n148 = Unbundle By Name(w248) -> ("Left IR Sensor"=w249:dbl)
        "Left IR Sensor" <- w249
        n149 = Unbundle By Name(w254) -> ("Time up flag"=w255:bool)
        "Time up flag" <- w255
        n150 = Unbundle By Name(w256) -> ("Yaw"=w257:dbl, "Compass"=w251:dbl)
        n151 = Unbundle By Name(w258) -> ("y Stepper Position"=w260:u8, "z Stepper Position"=w259:u8)
        n152 = Unbundle By Name(w274) -> ("xDistance"=w271:dbl, "yDistance"=w272:dbl, "wDistance"=w273:dbl)
        n153 = Unbundle By Name(w262) -> ("Recognized Object"=w261:bool, "Object X coordinate"=w264:dbl, "Object Y coordinate"=w263:dbl)
        n154 = Unbundle By Name(w285) -> ("PING_A"=w277:u8, "PING_B"=w276:u8, "PING_C"=w275:u8, "PING_D"=w270:u8)
        n155 = case shown="31" w284 {
          tunnel: [w289 w300 w313 w323 w398 w412 w448 w501 w543 w590 w633 w687 w734 w774 w834 w879 w919 w967 w1009 w1061 w1098 w1149 w1192 w1235 w1266 w1314 w1355 w1406 w1451 w1491 w1539 w1592] -> w283
          tunnel: w282 -> [w289 w303 w314 w326 w400 w413 w457 w499 w547 w591 w639 w680 w737 w781 w824 w882 w925 w966 w1012 w1051 w1104 w1139 w1187 w1226 w1270 w1321 w1360 w1396 w1454 w1497 w1538 w1591]
          tunnel: [State_Type_Definitions."Idle" ("Enum") State_Type_Definitions."Idle" ("Enum") w309 w325 State_Type_Definitions."Shutdown" ("Enum") w414 w455 w502 w544 w589 w634 w686 w735 w776 w833 w880 w926 w968 w1011 w1060 w1105 w1148 w1193 w1227 w1267 w1315 w1356 w1405 w1452 w1498 w1540 w1593] -> w281
          tunnel: w280 -> [_ _ w312 w329 _ w419 w451 w498 w548 w598 w638 w684 w738 w780 w831 w877 w924 w964 w1013 w1058 w1103 w1146 w1190 w1234 w1274 w1320 w1363 w1403 w1449 w1496 w1536 w1589]
          tunnel: w279 -> [_ _ _ w328 _ w418 w450 w497 w549 w597 w637 w683 w731 w779 w830 w876 w923 w963 w1014 w1057 w1102 w1145 w1189 w1232 w1269 w1319 w1362 w1402 w1448 w1495 w1535 w1588]
          tunnel: w278 -> [_ _ w311 w324 _ w417 w449 w496 w550 w596 w636 w682 w730 w778 w832 w878 w922 w962 w1015 w1059 w1101 w1147 w1188 w1233 w1273 w1318 w1361 w1404 w1450 w1494 w1534 w1587]
          tunnel: w267 -> [_ _ _ _ _ w411 w456 w495 w551 w593 w632 w685 w736 w782 w825 w883 w920 w965 w1016 w1052 w1099 w1140 w1191 w1230 w1272 w1313 w1359 w1397 w1455 w1492 w1537 w1590]
          tunnel: w277 -> [_ _ _ _ _ _ _ _ _ _ _ _ _ _ _ _ _ _ _ _ _ _ _ _ _ _ _ _ _ _ _ _]
          tunnel: w276 -> [_ _ _ _ _ _ _ w494 _ _ _ w676 w719 w772 _ w869 _ _ _ _ _ _ _ _ _ _ _ _ w1441 _ _ _]
          tunnel: w275 -> [_ _ _ _ _ _ _ w493 _ _ _ w677 w720 w773 _ w870 _ _ _ _ _ _ _ _ _ _ _ _ w1442 _ _ _]
          tunnel: w273 -> [_ _ _ _ _ _ _ _ _ w595 _ _ _ _ _ _ _ _ _ _ _ _ _ _ _ _ _ _ _ _ _ _]
          tunnel: w272 -> [_ _ _ _ _ w410 _ _ w542 _ _ _ _ w777 _ _ _ _ _ _ _ _ _ _ _ _ _ _ _ _ _ _]
          tunnel: w271 -> [_ _ _ _ _ _ _ _ _ _ _ _ w725 _ _ _ _ _ _ _ _ _ _ _ _ _ _ _ _ _ _ w1575]
          tunnel: w270 -> [_ _ _ _ _ _ _ _ _ _ _ _ _ _ _ _ _ _ _ _ _ _ _ _ _ _ _ _ _ _ _ _]
          tunnel: [State_Type_Definitions."Idle" ("Enum") State_Type_Definitions."Idle" ("Enum") State_Type_Definitions."Idle" ("Enum") State_Type_Definitions."Idle" ("Enum") State_Type_Definitions."Shutdown" ("Enum") w407 w454 w500 w545 w586 w631 w679 w733 w775 w835 w881 w918 w969 w1010 w1062 w1097 w1150 w1194 w1228 w1268 w1316 w1358 w1407 w1453 w1490 w1541 w1594] -> w266
          tunnel: w265 -> [_ _ w309 _ _ _ _ _ _ _ _ _ _ _ _ _ _ _ _ _ _ _ _ _ _ _ _ _ _ _ _ _]
          tunnel: w261 -> [_ _ _ _ _ _ _ _ _ _ _ _ _ _ _ _ _ _ _ _ _ _ _ w1229 _ _ _ _ _ _ _ _]
          tunnel: w264 -> [_ _ _ _ _ _ _ _ _ _ _ _ _ _ _ _ _ _ _ _ _ _ _ _ _ _ _ _ _ _ _ w1584]
          tunnel: w263 -> [_ _ _ _ _ _ _ _ _ _ _ _ _ _ _ _ _ _ w1005 _ _ _ _ _ _ _ _ _ _ _ _ _]
          tunnel: w260 -> [_ _ _ _ _ _ _ _ _ _ _ _ _ _ _ _ _ _ w1004 _ _ _ _ _ _ _ _ _ _ _ _ _]
          tunnel: w259 -> [_ _ _ _ _ _ w453 _ _ _ w629 _ _ _ w828 _ _ _ _ w1055 _ w1143 w1186 _ w1271 _ _ w1400 _ _ _ _]
          tunnel: w257 -> [_ _ _ _ _ _ _ _ _ _ _ _ _ _ _ _ _ _ _ _ _ _ _ _ _ _ _ _ _ _ _ _]
          tunnel: w255 -> [_ _ _ _ _ _ _ _ _ _ _ _ _ _ _ _ w916 w959 _ _ w1095 _ _ _ _ _ _ _ _ w1488 w1531 _]
          tunnel: w253 -> [w287 w298 w308 w321 w396 w406 w452 w492 w546 w585 w630 w678 w729 w771 w823 w874 w917 w960 w1007 w1050 w1096 w1138 w1183 w1225 w1265 w1317 w1357 w1395 w1446 w1489 w1532 w1585]
          tunnel: [w287 w297 w308 w321 w396 w406 w452 w492 w546 w585 w630 w678 w729 w771 w823 w874 w917 w960 w1006 w1050 w1096 w1138 w1183 w1225 w1265 w1317 w1357 w1395 w1446 w1489 w1532 w1585] -> w252
          tunnel: w251 -> [_ _ _ _ _ _ _ _ _ _ _ _ _ _ _ _ _ _ _ _ _ _ _ _ _ w1312 _ _ _ _ _ _]
          tunnel: [_ _ _ TRUE _ _ _ _ _ _ _ _ _ _ _ _ _ _ _ _ _ _ _ _ _ _ _ _ _ _ _ _] -> w250
          tunnel: w249 -> [_ _ _ _ _ _ _ _ _ _ _ _ _ _ _ _ _ _ _ _ _ _ _ _ _ _ _ _ _ _ _ _]
          tunnel: w247 -> [w286 w295 w307 w319 w395 w405 w447 w491 w539 w584 w626 w671 w718 w770 w822 w867 w915 w958 w1001 w1049 w1094 w1137 w1182 w1224 w1264 w1308 w1354 w1394 w1439 w1487 w1530 w1581]
          tunnel: [w286 w294 w307 w319 w395 w405 w447 w491 w539 w584 w626 w671 w718 w770 w822 w867 w915 w958 w1001 w1049 w1094 w1137 w1182 w1224 w1264 w1308 w1354 w1394 w1439 w1487 w1530 w1580] -> w246
          frame 0 {
            # ">>> yStepper command>>>"
          }
          frame 1 {
            # ">>> yStepper command>>>"
            n156 = for {
              shift-right: [w306] -> w300
              shift-left: w303 -> [w305]
              tunnel: string[] ["INIT", "RESET ARM", "RESET FLAGS", "RESET YAW", "NAVX CALIBRATE"] -> [w304] mode=indexing
              n157 = Enqueue Element(queue=w305, element=w304) -> (queue out=w306:refnum<queue>)  [unwired: 2 in, 2 out]
            }
            n158 = Bundle By Name(cluster=w298, "yStepper desired"=u8 0) -> (w297:T10)
            n159 = Bundle By Name(cluster=w295, "ySpeed"=0.0, "xSpeed"=0.0, "wSpeed"=0.0) -> (w294:T8)
          }
          frame 3 {
            # ">>> yStepper command>>>"
            n160 = Flush Queue(queue=w312, error in (no error)=w311) -> ()  [unwired: 3 out]
            n161 = for {
              shift-right: [w318] -> w313
              shift-left: w314 -> [w317]
              tunnel: string[] ["STOP", "RESET ENCODERS", "RESET YAW", "RESET ARM", "RESET FLAGS", "DISPOSE BUFFERS", "CAM CLOSE"] -> [w316] mode=indexing
              n162 = Enqueue Element(queue=w317, element=w316) -> (queue out=w318:refnum<queue>)  [unwired: 2 in, 2 out]
            }
          }
          frame 4, Default {
            (unwired) TRUE ("Green LED")
            # ">>> yStepper command>>>"
            n163 = Dequeue Element(queue=w329, timeout in ms (-1)=w328, error in (no error)=w324) -> (element=w327:T7)  [unwired: 3 out]
            n164 = case shown="\"Start Task 4\"" w327 {
              tunnel: [w331 w338 w345 w352 w359 w366 w373 w375 w383 w389] -> w323
              tunnel: w326 -> [w332 w339 w346 w353 w360 w367 w373 w376 w382 w390]
              tunnel: [State_Type_Definitions."Task 1" ("Enum") State_Type_Definitions."Task 2:Raise Arm" ("Enum") State_Type_Definitions."Task 3" ("Enum") State_Type_Definitions."Task 4_A" ("Enum") State_Type_Definitions."Task 5A: ARM CAM HEIGHT" ("Enum") State_Type_Definitions."Task 6_A" ("Enum") State_Type_Definitions."Idle" ("Enum") State_Type_Definitions."Shutdown" ("Enum") State_Type_Definitions."Task 9A: Raise Arm" ("Enum") State_Type_Definitions."Task 8A: RAISE ARM" ("Enum")] -> w325
              frame "Start Task 1" {
                n165 = for {
                  shift-right: [w336] -> w331
                  shift-left: w332 -> [w335]
                  tunnel: string[] ["RESET ENCODERS", "RESET YAW", "FORWARD", "READ ENCODERS"] -> [w334] mode=indexing
                  n166 = Enqueue Element(queue=w335, element=w334) -> (queue out=w336:refnum<queue>)  [unwired: 2 in, 2 out]
                }
              }
              frame "Start Task 2" {
                n167 = for {
                  shift-right: [w343] -> w338
                  shift-left: w339 -> [w342]
                  tunnel: string[] ["RESET ENCODERS", "RESET YAW", "READ ULTRASONIC", "ARDUINO - ULTRASONIC"] -> [w341] mode=indexing
                  n168 = Enqueue Element(queue=w342, element=w341) -> (queue out=w343:refnum<queue>)  [unwired: 2 in, 2 out]
                }
              }
              frame "Start Task 3" {
                n169 = for {
                  shift-right: [w350] -> w345
                  shift-left: w346 -> [w349]
                  tunnel: string[] ["RESET ENCODERS", "READ ENCODERS", "R-ACW"] -> [w348] mode=indexing
                  n170 = Enqueue Element(queue=w349, element=w348) -> (queue out=w350:refnum<queue>)  [unwired: 2 in, 2 out]
                }
              }
              frame "Start Task 4" {
                n171 = for {
                  shift-right: [w357] -> w352
                  shift-left: w353 -> [w356]
                  tunnel: string[] ["RESET YAW", "RESET ENCODERS", "RESET ARM", "RESET FLAGS", "", ""] -> [w355] mode=indexing
                  n172 = Enqueue Element(queue=w356, element=w355) -> (queue out=w357:refnum<queue>)  [unwired: 2 in, 2 out]
                }
              }
              frame "Start Task 5" {
                n173 = for {
                  shift-right: [w364] -> w359
                  shift-left: w360 -> [w363]
                  tunnel: string[] ["RESET YAW", "RESET ENCODERS", "READ STEPPER VALUES", "Z STEPPER CAM HEIGHT", "", ""] -> [w362] mode=indexing
                  n174 = Enqueue Element(queue=w363, element=w362) -> (queue out=w364:refnum<queue>)  [unwired: 2 in, 2 out]
                }
              }
              frame "Start Task 6" {
                n175 = for {
                  shift-right: [w371] -> w366
                  shift-left: w367 -> [w370]
                  tunnel: string[] ["OPEN LOG CAM ", "", "", "", "", ""] -> [w369] mode=indexing
                  n176 = Enqueue Element(queue=w370, element=w369) -> (queue out=w371:refnum<queue>)  [unwired: 2 in, 2 out]
                }
              }
              frame "None", Default {
              }
              frame "Exit" {
                n177 = for {
                  shift-right: [w380] -> w375
                  shift-left: w376 -> [w379]
                  tunnel: string[] ["STOP", "RESET ENCODERS", "RESET YAW", "EXIT"] -> [w378] mode=indexing
                  n178 = Enqueue Element(queue=w379, element=w378) -> (queue out=w380:refnum<queue>)  [unwired: 2 in, 2 out]
                }
              }
              frame "Start Task 9" {
                n179 = for {
                  shift-right: [w387] -> w383
                  shift-left: w382 -> [w386]
                  tunnel: string[] ["RESET ENCODERS", "READ ENCODERS", "Z STEPPER CAM HEIGHT"] -> [w385] mode=indexing
                  n180 = Enqueue Element(queue=w386, element=w385) -> (queue out=w387:refnum<queue>)  [unwired: 2 in, 2 out]
                }
              }
              frame "Start Task 8 - BALL" {
                n181 = for {
                  shift-right: [w394] -> w389
                  shift-left: w390 -> [w393]
                  tunnel: string[] ["RESET YAW", "RESET ENCODERS", "RESET ARM", "RESET FLAGS"] -> [w392] mode=indexing
                  n182 = Enqueue Element(queue=w393, element=w392) -> (queue out=w394:refnum<queue>)  [unwired: 2 in, 2 out]
                }
              }
            }
          }
          frame 5 {
            # ">>> yStepper command>>>"
            n183 = for {
              shift-right: [w404] -> w398
              shift-left: w400 -> [w403]
              tunnel: string[] ["INIT", "RESET ENCODERS", "RESET FLAGS", "CAM CLOSE", "DISPOSE BUFFERS", "EXIT", ""] -> [w402] mode=indexing
              n184 = Enqueue Element(queue=w403, element=w402) -> (queue out=w404:refnum<queue>)  [unwired: 2 in, 2 out]
            }
          }
          frame 6 {
            # ">>> yStepper command>>>"
            # "Use 250"
            n185 = Dequeue Element(queue=w419, timeout in ms (-1)=w418, error in (no error)=w417) -> (element=w416:T7)  [unwired: 3 out]
            n186 = Greater?(x=w410, y=265.0) -> (0:w408:bool)
            n187 = Or(x=w408, y=w411) -> (x .or. y?=w415:bool)
            n188 = case shown="\"None\", Default" w416 {
              tunnel: w415 -> [w422 _]
              tunnel: [w426 State_Type_Definitions."True Stop" ("Enum")] -> w414
              tunnel: w413 -> [w423 w441]
              tunnel: [w421 w440] -> w412
              tunnel: [State_Type_Definitions."Idle" ("Enum") State_Type_Definitions."Shutdown" ("Enum")] -> w407
              frame "None", Default {
                n189 = case shown="True" w422 {
                  tunnel: w423 -> [w429 w435]
                  tunnel: [w428 w433] -> w421
                  frame False {
                    n190 = for {
                      shift-right: [w431] -> w428
                      shift-left: w429 -> [w432]
                      tunnel: string[] ["READ ENCODERS", "READ NAVX", "FORWARD"] ("element") -> [w430] mode=indexing
                      n191 = Enqueue Element(queue=w432, element=w430) -> (queue out=w431:refnum<queue>)  [unwired: 2 in, 2 out]
                    }
                  }
                  frame True {
                    n192 = for {
                      shift-right: [w437] -> w433
                      shift-left: w435 -> [w438]
                      tunnel: string[] ["RESET YAW", "RESET ENCODERS", "STOP", ""] -> [w436] mode=indexing
                      n193 = Enqueue Element(queue=w438, element=w436) -> (queue out=w437:refnum<queue>)  [unwired: 2 in, 2 out]
                    }
                  }
                }
                n194 = Select(t=State_Type_Definitions."True Stop" ("Enum"), s=w422, f=State_Type_Definitions."Task 1" ("Enum")) -> (s? t:f=w426:u16)
              }
              frame "Exit" {
                n195 = for {
                  shift-right: [w445] -> w440
                  shift-left: w441 -> [w446]
                  tunnel: string[] ["STOP", "RESET ENCODERS", "RESET YAW", ""] -> [w444] mode=indexing
                  n196 = Enqueue Element(queue=w446, element=w444) -> (queue out=w445:refnum<queue>)  [unwired: 2 in, 2 out]
                }
              }
            }
          }
          frame 8 {
            # ">> Stepper height reeached >>"
            # ">>> yStepper command>>>"
            # ">> Manual override >>"
            n197 = Dequeue Element(queue=w451, timeout in ms (-1)=w450, error in (no error)=w449) -> (element=w460:T7)  [unwired: 3 out]
            n198 = Equal?(x=w453, y=u8 60) -> (x = y?=w458:bool)
            n199 = case shown="\"None\", Default" w460 {
              tunnel: [w471 State_Type_Definitions."True Stop" ("Enum")] -> w455
              tunnel: [w469 w486] -> w448
              tunnel: w457 -> [w468 _]
              tunnel: w456 -> [w462 _]
              tunnel: [State_Type_Definitions."Idle" ("Enum") State_Type_Definitions."Shutdown" ("Enum")] -> w454
              tunnel: w458 -> [w461 _]
              frame "None", Default {
                # ">> WIill proceed to part ii if not manual override >>"
                # ">>If ENABLE or Trigger is set to true>>"
                n200 = Or(x=w461, y=w462) -> (x .or. y?=w463:bool)
                n201 = case shown="True" w461 {
                  tunnel: [w474 w480] -> w469
                  tunnel: w468 -> [w473 w479]
                  frame False {
                    n202 = for {
                      shift-right: [w476] -> w474
                      shift-left: w473 -> [w477]
                      tunnel: string[] ["Z STEPPER CAM HEIGHT", "READ STEPPER VALUES"] ("element") -> [w475] mode=indexing
                      n203 = Enqueue Element(queue=w477, element=w475) -> (queue out=w476:refnum<queue>)  [unwired: 2 in, 2 out]
                    }
                  }
                  frame True {
                    n204 = for {
                      shift-right: [w482] -> w480
                      shift-left: w479 -> [w483]
                      tunnel: string[] ["ARDUINO - ULTRASONIC", "READ ULTRASONIC", "", "", "", ""] -> [w481] mode=indexing
                      n205 = Enqueue Element(queue=w483, element=w481) -> (queue out=w482:refnum<queue>)  [unwired: 2 in, 2 out]
                    }
                  }
                }
                n206 = Select(t=State_Type_Definitions."True Stop" ("Enum"), s=w462, f=State_Type_Definitions."Task 2:Sensor Mode" ("Enum")) -> (s? t:f=w465:T6)
                n207 = Select(t=w465, s=w463, f=State_Type_Definitions."Task 2:Raise Arm" ("Enum")) -> (s? t:f=w471:T6)
              }
              frame "Exit" {
                n208 = for {
                  shift-right: [w489] -> w486
                  shift-left: _ -> [w490]
                  tunnel: string[] ["STOP", "RESET ENCODERS", "RESET YAW", ""] -> [w488] mode=indexing
                  n209 = Enqueue Element(queue=w490, element=w488) -> (queue out=w489:refnum<queue>)  [unwired: 2 in, 2 out]
                }
              }
            }
          }
          frame 9 {
            w506 = u8 20 ("y")
            # ">>> yStepper command>>>"
            # ">>Object detected>>"
            n210 = Dequeue Element(queue=w498, timeout in ms (-1)=w497, error in (no error)=w496) -> (element=w507:T7)  [unwired: 3 out]
            n211 = Less?(x=w494, y=w506) -> (x < y?=w505:bool)
            n212 = Less?(x=w493, y=w506) -> (x < y?=w504:bool)
            n213 = Or(x=w505, y=w504) -> (x .or. y?=w503:bool)
            "Obstacle detected" <- w503
            n214 = case shown="\"None\", Default" w507 {
              tunnel: w503 -> [w510 _]
              tunnel: [w517 State_Type_Definitions."True Stop" ("Enum")] -> w502
              tunnel: w495 -> [w509 _]
              tunnel: w499 -> [w516 w533]
              tunnel: [w515 w534] -> w501
              tunnel: [State_Type_Definitions."Idle" ("Enum") State_Type_Definitions."Shutdown" ("Enum")] -> w500
              frame "None", Default {
                n215 = case shown="True" w510 {
                  tunnel: w516 -> [w520 w527]
                  tunnel: [w521 w526] -> w515
                  frame False {
                    n216 = for {
                      tunnel: string[] ["READ ULTRASONIC", "STOP"] ("element") -> [w522] mode=indexing
                      shift-right: [w524] -> w521
                      shift-left: w520 -> [w523]
                      n217 = Enqueue Element(queue=w523, element=w522) -> (queue out=w524:refnum<queue>)  [unwired: 2 in, 2 out]
                    }
                  }
                  frame True {
                    n218 = for {
                      shift-right: [w529] -> w526
                      shift-left: w527 -> [w530]
                      tunnel: string[] ["RESET ENCODERS", "READ NAVX", "READ ENCODERS"] -> [w528] mode=indexing
                      n219 = Enqueue Element(queue=w530, element=w528) -> (queue out=w529:refnum<queue>)  [unwired: 2 in, 2 out]
                    }
                  }
                }
                n220 = Or(x=w510, y=w509) -> (x .or. y?=w508:bool)
                n221 = Select(t=State_Type_Definitions."True Stop" ("Enum"), s=w509, f=State_Type_Definitions."Task 2:Reverse Mode" ("Enum")) -> (s? t:f=w511:T6)
                n222 = Select(t=w511, s=w508, f=State_Type_Definitions."Task 2:Sensor Mode" ("Enum")) -> (s? t:f=w517:T6)
              }
              frame "Exit" {
                n223 = for {
                  shift-right: [w537] -> w534
                  shift-left: w533 -> [w538]
                  tunnel: string[] ["STOP", "RESET ENCODERS", "RESET YAW", "ARDUINO MODE 0"] -> [w536] mode=indexing
                  n224 = Enqueue Element(queue=w538, element=w536) -> (queue out=w537:refnum<queue>)  [unwired: 2 in, 2 out]
                }
              }
            }
          }
          frame 10 {
            # ">>> yStepper command>>>"
            n225 = Dequeue Element(queue=w548, timeout in ms (-1)=w549, error in (no error)=w550) -> (element=w552:T7)  [unwired: 3 out]
            n226 = Less?(x=w542, y=-50.0) -> (x < y?=w540:bool)
            n227 = case shown="\"None\", Default" w552 {
              tunnel: [w562 State_Type_Definitions."True Stop" ("Enum")] -> w544
              tunnel: w551 -> [w555 _]
              tunnel: w547 -> [w561 w578]
              tunnel: [w560 w579] -> w543
              tunnel: [State_Type_Definitions."Idle" ("Enum") State_Type_Definitions."Shutdown" ("Enum")] -> w545
              tunnel: w540 -> [w553 _]
              frame "None", Default {
                n228 = case shown="False" w553 {
                  tunnel: w561 -> [w565 w572]
                  tunnel: [w566 w571] -> w560
                  frame False {
                    n229 = for {
                      tunnel: string[] ["READ ENCODERS", "REVERSE", "READ NAVX"] ("element") -> [w567] mode=indexing
                      shift-right: [w569] -> w566
                      shift-left: w565 -> [w568]
                      n230 = Enqueue Element(queue=w568, element=w567) -> (queue out=w569:refnum<queue>)  [unwired: 2 in, 2 out]
                    }
                  }
                  frame True {
                    n231 = for {
                      shift-right: [w574] -> w571
                      shift-left: w572 -> [w575]
                      tunnel: string[] ["STOP", "ARDUINO - ULTRASONIC", "READ ULTRASONIC", "RESET ENCODERS"] -> [w573] mode=indexing
                      n232 = Enqueue Element(queue=w575, element=w573) -> (queue out=w574:refnum<queue>)  [unwired: 2 in, 2 out]
                    }
                  }
                }
                n233 = Or(x=w553, y=w555) -> (x .or. y?=w554:bool)
                n234 = Select(t=State_Type_Definitions."True Stop" ("Enum"), s=w555, f=State_Type_Definitions."Task 2:Sensor Mode" ("Enum")) -> (s? t:f=w556:T6)
                n235 = Select(t=w556, s=w554, f=State_Type_Definitions."Task 2:Reverse Mode" ("Enum")) -> (s? t:f=w562:T6)
              }
              frame "Exit" {
                n236 = for {
                  shift-right: [w582] -> w579
                  shift-left: w578 -> [w583]
                  tunnel: string[] ["STOP", "RESET ENCODERS", "RESET YAW", "ARDUINO MODE 0"] -> [w581] mode=indexing
                  n237 = Enqueue Element(queue=w583, element=w581) -> (queue out=w582:refnum<queue>)  [unwired: 2 in, 2 out]
                }
              }
            }
          }
          frame 11 {
            # ">>> yStepper command>>>"
            n238 = Dequeue Element(queue=w598, timeout in ms (-1)=w597, error in (no error)=w596) -> (element=w587:T7)  [unwired: 3 out]
            n239 = Greater?(x=w595, y=160.0) -> (0:w592:bool)
            n240 = Or(x=w592, y=w593) -> (x .or. y?=w588:bool)
            n241 = case shown="\"None\", Default" w587 {
              tunnel: w588 -> [w601 _]
              tunnel: [w605 State_Type_Definitions."True Stop" ("Enum")] -> w589
              tunnel: w591 -> [w602 w621]
              tunnel: [w600 w620] -> w590
              tunnel: [State_Type_Definitions."Idle" ("Enum") State_Type_Definitions."Shutdown" ("Enum")] -> w586
              frame "None", Default {
                n242 = case shown="False" w601 {
                  tunnel: w602 -> [w608 w614]
                  tunnel: [w607 w612] -> w600
                  frame False {
                    n243 = for {
                      shift-right: [w610] -> w607
                      shift-left: w608 -> [w611]
                      tunnel: string[] ["READ ENCODERS", "R-CW"] ("element") -> [w609] mode=indexing
                      n244 = Enqueue Element(queue=w611, element=w609) -> (queue out=w610:refnum<queue>)  [unwired: 2 in, 2 out]
                    }
                  }
                  frame True {
                    n245 = for {
                      shift-right: [w616] -> w612
                      shift-left: w614 -> [w617]
                      tunnel: string[] ["RESET YAW", "RESET ENCODERS", "STOP", "ARDUINO MODE 0"] -> [w615] mode=indexing
                      n246 = Enqueue Element(queue=w617, element=w615) -> (queue out=w616:refnum<queue>)  [unwired: 2 in, 2 out]
                    }
                  }
                }
                n247 = Select(t=State_Type_Definitions."True Stop" ("Enum"), s=w601, f=State_Type_Definitions."Task 3" ("Enum")) -> (s? t:f=w605:T6)
              }
              frame "Exit" {
                n248 = for {
                  shift-right: [w624] -> w620
                  shift-left: w621 -> [w625]
                  tunnel: string[] ["STOP", "RESET ENCODERS", "RESET YAW", ""] -> [w623] mode=indexing
                  n249 = Enqueue Element(queue=w625, element=w623) -> (queue out=w624:refnum<queue>)  [unwired: 2 in, 2 out]
                }
              }
            }
          }
          frame 12 {
            # ">> Stepper height reeached >>"
            # ">>> yStepper command>>>"
            # ">> Manual override >>"
            n250 = Dequeue Element(queue=w638, timeout in ms (-1)=w637, error in (no error)=w636) -> (element=w635:T7)  [unwired: 3 out]
            n251 = Equal?(x=w629, y=u8 60) -> (x = y?=w627:bool)
            n252 = case shown="\"Exit\"" w635 {
              tunnel: [w650 State_Type_Definitions."True Stop" ("Enum")] -> w634
              tunnel: [w648 w666] -> w633
              tunnel: w639 -> [w647 w663]
              tunnel: w632 -> [w641 _]
              tunnel: [State_Type_Definitions."Idle" ("Enum") State_Type_Definitions."Shutdown" ("Enum")] -> w631
              tunnel: w627 -> [w640 _]
              frame "None", Default {
                # ">> WIill proceed to part ii if not manual override >>"
                # ">>If ENABLE or Trigger is set to true>>"
                n253 = Or(x=w640, y=w641) -> (x .or. y?=w642:bool)
                n254 = case shown="False" w640 {
                  tunnel: [w653 w659] -> w648
                  tunnel: w647 -> [w652 w658]
                  frame False {
                    n255 = for {
                      shift-right: [w655] -> w653
                      shift-left: w652 -> [w656]
                      tunnel: string[] ["Z STEPPER CAM HEIGHT", "READ STEPPER VALUES"] ("element") -> [w654] mode=indexing
                      n256 = Enqueue Element(queue=w656, element=w654) -> (queue out=w655:refnum<queue>)  [unwired: 2 in, 2 out]
                    }
                  }
                  frame True {
                    n257 = for {
                      shift-right: [w661] -> w659
                      shift-left: w658 -> [w662]
                      tunnel: string[] ["ARDUINO - ULTRASONIC", "READ ULTRASONIC", "FORWARD", "", "", ""] -> [w660] mode=indexing
                      n258 = Enqueue Element(queue=w662, element=w660) -> (queue out=w661:refnum<queue>)  [unwired: 2 in, 2 out]
                    }
                  }
                }
                n259 = Select(t=State_Type_Definitions."True Stop" ("Enum"), s=w641, f=State_Type_Definitions."Task 4_B" ("Enum")) -> (s? t:f=w644:T6)
                n260 = Select(t=w644, s=w642, f=State_Type_Definitions."Task 4_A" ("Enum")) -> (s? t:f=w650:T6)
              }
              frame "Exit" {
                n261 = for {
                  shift-right: [w669] -> w666
                  shift-left: w663 -> [w670]
                  tunnel: string[] ["STOP", "RESET ENCODERS", "RESET YAW", ""] -> [w668] mode=indexing
                  n262 = Enqueue Element(queue=w670, element=w668) -> (queue out=w669:refnum<queue>)  [unwired: 2 in, 2 out]
                }
              }
            }
          }
          frame 13 {
            w675 = u8 20
            # ">> Path blocked >>"
            # ">>> yStepper command>>>"
            # ">> Manual override >>"
            n263 = Dequeue Element(queue=w684, timeout in ms (-1)=w683, error in (no error)=w682) -> (element=w681:T7)  [unwired: 3 out]
            n264 = Less?(x=w677, y=w675) -> (x < y?=w672:bool)
            n265 = Less?(x=w676, y=w675) -> (x < y?=w673:bool)
            n266 = And(x=w673, y=w672) -> (x .and. y?=w674:bool)
            n267 = case shown="\"None\", Default" w681 {
              tunnel: [w698 State_Type_Definitions."True Stop" ("Enum")] -> w686
              tunnel: [w696 w713] -> w687
              tunnel: w680 -> [w695 _]
              tunnel: w685 -> [w689 _]
              tunnel: [State_Type_Definitions."Idle" ("Enum") State_Type_Definitions."Shutdown" ("Enum")] -> w679
              tunnel: w674 -> [w688 _]
              frame "None", Default {
                # ">> Manual override forces program to true stop >>"
                # ">>If ENABLE or Trigger is set to true>>"
                n268 = Or(x=w688, y=w689) -> (x .or. y?=w694:bool)
                n269 = case shown="True" w688 {
                  tunnel: [w701 w706] -> w696
                  tunnel: w695 -> [w700 w705]
                  frame False {
                    n270 = for {
                      shift-right: [w703] -> w701
                      shift-left: w700 -> [w704]
                      tunnel: string[] ["FORWARD", "READ ULTRASONIC", "READ NAVX"] ("element") -> [w702] mode=indexing
                      n271 = Enqueue Element(queue=w704, element=w702) -> (queue out=w703:refnum<queue>)  [unwired: 2 in, 2 out]
                    }
                  }
                  frame True {
                    n272 = for {
                      shift-right: [w709] -> w706
                      shift-left: w705 -> [w710]
                      tunnel: string[] ["STOP", "RESET YAW", "RESET ENCODERS", "RESET FLAGS"] -> [w708] mode=indexing
                      n273 = Enqueue Element(queue=w710, element=w708) -> (queue out=w709:refnum<queue>)  [unwired: 2 in, 2 out]
                    }
                  }
                }
                n274 = Select(t=State_Type_Definitions."True Stop" ("Enum"), s=w689, f=State_Type_Definitions."Task 4_C" ("Enum")) -> (s? t:f=w691:T6)
                n275 = Select(t=w691, s=w694, f=State_Type_Definitions."Task 4_B" ("Enum")) -> (s? t:f=w698:T6)
              }
              frame "Exit" {
                n276 = for {
                  shift-right: [w716] -> w713
                  shift-left: _ -> [w717]
                  tunnel: string[] ["STOP", "RESET ENCODERS", "RESET YAW", ""] -> [w715] mode=indexing
                  n277 = Enqueue Element(queue=w717, element=w715) -> (queue out=w716:refnum<queue>)  [unwired: 2 in, 2 out]
                }
              }
            }
          }
          frame 14 {
            w728 = u8 20
            # ">> xDistance travelled>>"
            # ">> Path NOT blocked >>"
            # ">>> yStepper command>>>"
            # ">> Manual override >>"
            n278 = Dequeue Element(queue=w738, timeout in ms (-1)=w731, error in (no error)=w730) -> (element=w732:T7)  [unwired: 3 out]
            n279 = Greater?(x=w720, y=w728) -> (0:w726:bool)
            n280 = Greater?(x=w725, y=80.0) -> (0:w723:bool)
            n281 = Greater?(x=w719, y=w728) -> (0:w727:bool)
            n282 = And(x=w727, y=w726) -> (x .and. y?=w722:bool)
            n283 = And(x=w723, y=w722) -> (x .and. y?=w721:bool)
            n284 = case shown="\"Exit\"" w732 {
              tunnel: [w749 State_Type_Definitions."True Stop" ("Enum")] -> w735
              tunnel: [w747 w765] -> w734
              tunnel: w737 -> [w746 w762]
              tunnel: w736 -> [w740 _]
              tunnel: [State_Type_Definitions."Idle" ("t") State_Type_Definitions."Shutdown" ("Enum")] -> w733
              tunnel: w721 -> [w739 _]
              frame "None", Default {
                # ">> Manual override forces program to true stop >>"
                # ">>If ENABLE or Trigger is set to true>>"
                n285 = Or(x=w739, y=w740) -> (x .or. y?=w745:bool)
                n286 = case shown="False" w739 {
                  tunnel: [w752 w757] -> w747
                  tunnel: w746 -> [w750 w756]
                  frame False {
                    n287 = for {
                      shift-right: [w754] -> w752
                      shift-left: w750 -> [w755]
                      tunnel: string[] ["RIGHT", "READ NAVX", "READ ENCODERS", "READ ULTRASONIC"] ("element") -> [w753] mode=indexing
                      n288 = Enqueue Element(queue=w755, element=w753) -> (queue out=w754:refnum<queue>)  [unwired: 2 in, 2 out]
                    }
                  }
                  frame True {
                    n289 = for {
                      shift-right: [w760] -> w757
                      shift-left: w756 -> [w761]
                      tunnel: string[] ["STOP", "RESET YAW", "RESET ENCODERS", "ARDUINO - ULTRASONIC"] -> [w759] mode=indexing
                      n290 = Enqueue Element(queue=w761, element=w759) -> (queue out=w760:refnum<queue>)  [unwired: 2 in, 2 out]
                    }
                  }
                }
                n291 = Select(t=State_Type_Definitions."True Stop" ("Enum"), s=w740, f=State_Type_Definitions."Task 4_D" ("Enum")) -> (s? t:f=w741:T6)
                n292 = Select(t=w741, s=w745, f=State_Type_Definitions."Task 4_C" ("Enum")) -> (s? t:f=w749:T6)
              }
              frame "Exit" {
                n293 = for {
                  shift-right: [w768] -> w765
                  shift-left: w762 -> [w769]
                  tunnel: string[] ["STOP", "RESET ENCODERS", "RESET YAW", ""] -> [w767] mode=indexing
                  n294 = Enqueue Element(queue=w769, element=w767) -> (queue out=w768:refnum<queue>)  [unwired: 2 in, 2 out]
                }
              }
            }
          }
          frame 15 {
            w789 = u8 20
            # ">> yDistance travelled>>"
            # ">> Path blocked >>"
            # ">>> yStepper command>>>"
            # ">> Manual override >>"
            n295 = Dequeue Element(queue=w780, timeout in ms (-1)=w779, error in (no error)=w778) -> (element=w790:T7)  [unwired: 3 out]
            n296 = Less?(x=w773, y=w789) -> (x < y?=w787:bool)
            n297 = Greater?(x=w777, y=200.0) -> (0:w785:bool)
            n298 = Less?(x=w772, y=w789) -> (x < y?=w788:bool)
            n299 = And(x=w788, y=w787) -> (x .and. y?=w784:bool)
            n300 = Or(x=w785, y=w784) -> (x .or. y?=w783:bool)
            n301 = case shown="\"None\", Default" w790 {
              tunnel: [w801 State_Type_Definitions."True Stop" ("Enum")] -> w776
              tunnel: [w799 w817] -> w774
              tunnel: w781 -> [w798 w814]
              tunnel: w782 -> [w792 _]
              tunnel: [State_Type_Definitions."Idle" ("t") State_Type_Definitions."Shutdown" ("Enum")] -> w775
              tunnel: w783 -> [w791 _]
              frame "None", Default {
                # ">> Manual override forces program to true stop >>"
                # ">>If ENABLE or Trigger is set to true>>"
                n302 = Or(x=w791, y=w792) -> (x .or. y?=w797:bool)
                n303 = case shown="True" w791 {
                  tunnel: [w804 w809] -> w799
                  tunnel: w798 -> [w802 w808]
                  frame False {
                    n304 = for {
                      shift-right: [w806] -> w804
                      shift-left: w802 -> [w807]
                      tunnel: string[] ["FORWARD", "READ NAVX", "READ ENCODERS", "READ ULTRASONIC"] ("element") -> [w805] mode=indexing
                      n305 = Enqueue Element(queue=w807, element=w805) -> (queue out=w806:refnum<queue>)  [unwired: 2 in, 2 out]
                    }
                  }
                  frame True {
                    n306 = for {
                      shift-right: [w812] -> w809
                      shift-left: w808 -> [w813]
                      tunnel: string[] ["STOP", "RESET YAW", "RESET ENCODERS", "RESET FLAGS"] -> [w811] mode=indexing
                      n307 = Enqueue Element(queue=w813, element=w811) -> (queue out=w812:refnum<queue>)  [unwired: 2 in, 2 out]
                    }
                  }
                }
                n308 = Select(t=State_Type_Definitions."True Stop" ("Enum"), s=w792, f=State_Type_Definitions."True Stop" ("Enum")) -> (s? t:f=w793:T6)
                n309 = Select(t=w793, s=w797, f=State_Type_Definitions."Task 4_D" ("Enum")) -> (s? t:f=w801:T6)
              }
              frame "Exit" {
                n310 = for {
                  shift-right: [w820] -> w817
                  shift-left: w814 -> [w821]
                  tunnel: string[] ["STOP", "RESET ENCODERS", "RESET YAW", ""] -> [w819] mode=indexing
                  n311 = Enqueue Element(queue=w821, element=w819) -> (queue out=w820:refnum<queue>)  [unwired: 2 in, 2 out]
                }
              }
            }
          }
          frame 15 {
            # ">>> yStepper command>>>"
            # ">> Manual override >>"
            n312 = Dequeue Element(queue=w831, timeout in ms (-1)=w830, error in (no error)=w832) -> (element=w829:T7)  [unwired: 3 out]
            n313 = Equal?(x=w828, y=u8 60) -> (x = y?=w826:bool)
            n314 = case shown="\"None\", Default" w829 {
              tunnel: [w842 State_Type_Definitions."True Stop" ("Enum")] -> w833
              tunnel: [w845 w862] -> w834
              tunnel: [State_Type_Definitions."Idle" ("Enum") State_Type_Definitions."Shutdown" ("Enum")] -> w835
              tunnel: w826 -> [w841 _]
              tunnel: w825 -> [w840 _]
              tunnel: w824 -> [w836 w859]
              frame "None", Default {
                # "Stays in Task 5_A until stepper reaches desired \nheight"
                # "T: Go back to idle, F: Continue with task\""
                # ">> Manual override >>"
                n315 = case shown="True" w841 {
                  tunnel: [w849 w855] -> w845
                  tunnel: w836 -> [w847 w853]
                  frame False {
                    n316 = for {
                      tunnel: string[] ["Z STEPPER CAM HEIGHT", "READ STEPPER VALUES"] ("element") -> [w850] mode=indexing
                      shift-right: [w852] -> w849
                      shift-left: w847 -> [w851]
                      n317 = Enqueue Element(queue=w851, element=w850) -> (queue out=w852:refnum<queue>)  [unwired: 2 in, 2 out]
                    }
                  }
                  frame True {
                    n318 = for {
                      shift-right: [w857] -> w855
                      shift-left: w853 -> [w858]
                      tunnel: string[] ["ARDUINO - ULTRASONIC", "READ ULTRASONIC", ""] -> [w856] mode=indexing
                      n319 = Enqueue Element(queue=w858, element=w856) -> (queue out=w857:refnum<queue>)  [unwired: 2 in, 2 out]
                    }
                  }
                }
                n320 = Or(x=w841, y=w840) -> (x .or. y?=w843:bool)
                n321 = Select(t=State_Type_Definitions."True Stop" ("Enum"), s=w840, f=State_Type_Definitions."Task 5B: MOVE TO BOX" ("Enum")) -> (s? t:f=w837:u16)
                n322 = Select(t=w837, s=w843, f=State_Type_Definitions."Task 5A: ARM CAM HEIGHT" ("Enum")) -> (s? t:f=w842:u16)
              }
              frame "Exit" {
                n323 = for {
                  shift-right: [w865] -> w862
                  shift-left: w859 -> [w866]
                  tunnel: string[] ["STOP", "RESET ENCODERS", "RESET YAW", "ARDUINO MODE 0"] -> [w864] mode=indexing
                  n324 = Enqueue Element(queue=w866, element=w864) -> (queue out=w865:refnum<queue>)  [unwired: 2 in, 2 out]
                }
              }
            }
          }
          frame 16 {
            w873 = u8 20 ("y")
            # ">>> yStepper command>>>"
            n325 = Less?(x=w870, y=w873) -> (x < y?=w871:bool)
            n326 = Dequeue Element(queue=w877, timeout in ms (-1)=w876, error in (no error)=w878) -> (element=w875:T7)  [unwired: 3 out]
            n327 = Less?(x=w869, y=w873) -> (x < y?=w872:bool)
            n328 = And(x=w872, y=w871) -> (x .and. y?=w868:bool)
            n329 = case shown="\"None\", Default" w875 {
              tunnel: [w890 State_Type_Definitions."True Stop" ("Enum")] -> w880
              tunnel: [w893 w910] -> w879
              tunnel: [State_Type_Definitions."Idle" ("Enum") State_Type_Definitions."Shutdown" ("Enum")] -> w881
              tunnel: w883 -> [w889 _]
              tunnel: w882 -> [w885 w907]
              tunnel: w868 -> [w884 _]
              frame "None", Default {
                # "Stays in Task 5_B to capture image over 5 seconds"
                # "T: Go back to idle, F: Continue with task\""
                # ">> Manual override >>"
                n330 = case shown="True" w884 {
                  tunnel: [w897 w903] -> w893
                  tunnel: w885 -> [w895 w901]
                  frame False {
                    n331 = for {
                      tunnel: string[] ["FORWARD", "READ ULTRASONIC", "READ NAVX"] ("element") -> [w898] mode=indexing
                      shift-right: [w900] -> w897
                      shift-left: w895 -> [w899]
                      n332 = Enqueue Element(queue=w899, element=w898) -> (queue out=w900:refnum<queue>)  [unwired: 2 in, 2 out]
                    }
                  }
                  frame True {
                    n333 = for {
                      shift-right: [w905] -> w903
                      shift-left: w901 -> [w906]
                      tunnel: string[] ["STOP", "RESET ENCODERS", "OPEN LOG CAM", "SET TIMER 5"] -> [w904] mode=indexing
                      n334 = Enqueue Element(queue=w906, element=w904) -> (queue out=w905:refnum<queue>)  [unwired: 2 in, 2 out]
                    }
                  }
                }
                n335 = Or(x=w884, y=w889) -> (x .or. y?=w891:bool)
                n336 = Select(t=State_Type_Definitions."True Stop" ("Enum"), s=w889, f=State_Type_Definitions."Task 5C: CAM BURST" ("Enum")) -> (s? t:f=w886:u16)
                n337 = Select(t=w886, s=w891, f=State_Type_Definitions."Task 5B: MOVE TO BOX" ("Enum")) -> (s? t:f=w890:u16)
              }
              frame "Exit" {
                n338 = for {
                  shift-right: [w913] -> w910
                  shift-left: w907 -> [w914]
                  tunnel: string[] ["STOP", "RESET ENCODERS", "RESET YAW", "ARDUINO MODE 0"] -> [w912] mode=indexing
                  n339 = Enqueue Element(queue=w914, element=w912) -> (queue out=w913:refnum<queue>)  [unwired: 2 in, 2 out]
                }
              }
            }
          }
          frame 17 {
            # ">>> yStepper command>>>"
            # ">> Manual override >>"
            n340 = Dequeue Element(queue=w924, timeout in ms (-1)=w923, error in (no error)=w922) -> (element=w921:T7)  [unwired: 3 out]
            n341 = case shown="\"None\", Default" w921 {
              tunnel: [w933 State_Type_Definitions."True Stop" ("Enum")] -> w926
              tunnel: [w936 w953] -> w919
              tunnel: [State_Type_Definitions."Idle" ("Enum") State_Type_Definitions."Shutdown" ("Enum")] -> w918
              tunnel: w920 -> [w927 _]
              tunnel: w925 -> [w932 w950]
              tunnel: w916 -> [w931 _]
              frame "None", Default {
                # ">> Is time up? >>"
                # "Determines if object is in range to pick up"
                # ">> Manual override >>"
                n342 = case shown="True" w931 {
                  tunnel: [w940 w946] -> w936
                  tunnel: w932 -> [w938 w944]
                  frame False {
                    n343 = for {
                      tunnel: string[] ["CAM ACQ", "START TIMER"] ("element") -> [w941] mode=indexing
                      shift-right: [w943] -> w940
                      shift-left: w938 -> [w942]
                      n344 = Enqueue Element(queue=w942, element=w941) -> (queue out=w943:refnum<queue>)  [unwired: 2 in, 2 out]
                    }
                  }
                  frame True {
                    n345 = for {
                      shift-right: [w948] -> w946
                      shift-left: w944 -> [w949]
                      tunnel: string[] ["CAM CLOSE", "PROCESS IMAGE", "SET TIMER 5"] -> [w947] mode=indexing
                      n346 = Enqueue Element(queue=w949, element=w947) -> (queue out=w948:refnum<queue>)  [unwired: 2 in, 2 out]
                    }
                  }
                }
                n347 = Or(x=w931, y=w927) -> (x .or. y?=w934:bool)
                n348 = Select(t=State_Type_Definitions."True Stop" ("Enum"), s=w927, f=State_Type_Definitions."Task 5D: PROCESS IMAGE" ("Enum")) -> (s? t:f=w929:u16)
                n349 = Select(t=w929, s=w934, f=State_Type_Definitions."Task 5C: CAM BURST" ("Enum")) -> (s? t:f=w933:u16)
              }
              frame "Exit" {
                n350 = for {
                  shift-right: [w956] -> w953
                  shift-left: w950 -> [w957]
                  tunnel: string[] ["STOP", "RESET ENCODERS", "RESET YAW", "ARDUINO MODE 0"] -> [w955] mode=indexing
                  n351 = Enqueue Element(queue=w957, element=w955) -> (queue out=w956:refnum<queue>)  [unwired: 2 in, 2 out]
                }
              }
            }
          }
          frame 18 {
            # ">>> yStepper command>>>"
            n352 = Dequeue Element(queue=w964, timeout in ms (-1)=w963, error in (no error)=w962) -> (element=w961:T7)  [unwired: 3 out]
            n353 = case shown="\"None\", Default" w961 {
              tunnel: [w976 State_Type_Definitions."True Stop" ("Enum")] -> w968
              tunnel: [w979 w996] -> w967
              tunnel: [State_Type_Definitions."Idle" ("Enum") State_Type_Definitions."Shutdown" ("Enum")] -> w969
              tunnel: w965 -> [w975 _]
              tunnel: w966 -> [w971 w993]
              tunnel: w959 -> [w970 _]
              frame "None", Default {
                # ">> T: Breaks out of state loop; F: Stays in loop>>"
                # ">> Manual override >>"
                # ">> Checks if time is up>>"
                # "Stays in Task 5D until the object is detected"
                # "T: Go back to idle, F: Continue with task\""
                # ">> Manual override >>"
                n354 = case shown="True" w970 {
                  tunnel: [w983 w989] -> w979
                  tunnel: w971 -> [w981 w987]
                  frame False {
                    n355 = for {
                      tunnel: string[] ["START TIMER", "PROCESS IMAGE", ""] ("element") -> [w984] mode=indexing
                      shift-right: [w986] -> w983
                      shift-left: w981 -> [w985]
                      n356 = Enqueue Element(queue=w985, element=w984) -> (queue out=w986:refnum<queue>)  [unwired: 2 in, 2 out]
                    }
                  }
                  frame True {
                    n357 = for {
                      shift-right: [w991] -> w989
                      shift-left: w987 -> [w992]
                      tunnel: string[] ["CAM CLOSE", "", ""] -> [w990] mode=indexing
                      n358 = Enqueue Element(queue=w992, element=w990) -> (queue out=w991:refnum<queue>)  [unwired: 2 in, 2 out]
                    }
                  }
                }
                n359 = Or(x=w970, y=w975) -> (x .or. y?=w977:bool)
                n360 = Select(t=State_Type_Definitions."True Stop" ("Enum"), s=w975, f=State_Type_Definitions."Task 5E: POSITION ARM" ("Enum")) -> (s? t:f=w972:T6)
                n361 = Select(t=w972, s=w977, f=State_Type_Definitions."Task 5D: PROCESS IMAGE" ("Enum")) -> (s? t:f=w976:u16)
              }
              frame "Exit" {
                n362 = for {
                  shift-right: [w999] -> w996
                  shift-left: w993 -> [w1000]
                  tunnel: string[] ["STOP", "RESET ENCODERS", "RESET YAW", "ARDUINO MODE 0"] -> [w998] mode=indexing
                  n363 = Enqueue Element(queue=w1000, element=w998) -> (queue out=w999:refnum<queue>)  [unwired: 2 in, 2 out]
                }
              }
            }
          }
          frame 20 {
            # ">>> yStepper command>>>"
            n364 = Dequeue Element(queue=w1013, timeout in ms (-1)=w1014, error in (no error)=w1015) -> (element=w1017:T7)  [unwired: 3 out]
            n365 = formula code="if (pos < 100)\ny = 41;\n\nelse if (pos >= 100 && pos <= 140)\ny = 30;\n\nelse if (pos >= 141 && pos <= 170)\ny = 25;\n\nelse if (pos >= 171 &&pos <= 180) \ny = 20;\n\nelse if (pos >= 181&& pos <= 200)\ny = 15;\n\nelse if (pos >= 201 && pos <= 230)\ny = 10;\n\nelse if (pos >= 231 && pos <= 320)\ny = 8;\n\nelse if (pos > 320)\ny = 0;"("pos"=w1005) -> ("y"=w1008:dbl)
            n366 = To Unsigned Byte Integer(number=w1008) -> (unsigned 8bit integer=w1003:u8)
            n367 = Equal?(x=w1004, y=w1003) -> (x = y?=w1002:bool)
            n368 = case shown="\"None\", Default" w1017 {
              tunnel: [w1024 State_Type_Definitions."True Stop" ("Enum")] -> w1011
              tunnel: [w1027 w1044] -> w1009
              tunnel: [State_Type_Definitions."Idle" ("Enum") State_Type_Definitions."Shutdown" ("Enum")] -> w1010
              tunnel: w1016 -> [w1023 _]
              tunnel: w1012 -> [w1019 w1041]
              tunnel: w1002 -> [w1018 _]
              frame "None", Default {
                # ">> T: Breaks out of state loop; F: Stays in loop>>"
                # ">> Manual override >>"
                # ">> Checks if time is up>>"
                # "Stays in Task 5D until the object is detected"
                # "T: Go back to idle, F: Continue with task\""
                # ">> Manual override >>"
                n369 = case shown="False" w1018 {
                  tunnel: [w1031 w1037] -> w1027
                  tunnel: w1019 -> [w1029 w1035]
                  frame False {
                    n370 = for {
                      tunnel: string[] ["READ STEPPER VALUES", "Y STEPPER CONTROL", ""] ("element") -> [w1032] mode=indexing
                      shift-right: [w1034] -> w1031
                      shift-left: w1029 -> [w1033]
                      n371 = Enqueue Element(queue=w1033, element=w1032) -> (queue out=w1034:refnum<queue>)  [unwired: 2 in, 2 out]
                    }
                  }
                  frame True {
                    n372 = for {
                      shift-right: [w1039] -> w1037
                      shift-left: w1035 -> [w1040]
                      tunnel: string[] ["CAM CLOSE", "DISPOSE BUFFERS", ""] -> [w1038] mode=indexing
                      n373 = Enqueue Element(queue=w1040, element=w1038) -> (queue out=w1039:refnum<queue>)  [unwired: 2 in, 2 out]
                    }
                  }
                }
                n374 = Or(x=w1018, y=w1023) -> (x .or. y?=w1025:bool)
                n375 = Select(t=State_Type_Definitions."True Stop" ("Enum"), s=w1023, f=State_Type_Definitions."Task 5F: ARM GRAB HEIGHT" ("Enum")) -> (s? t:f=w1020:T6)
                n376 = Select(t=w1020, s=w1025, f=State_Type_Definitions."Task 5E: POSITION ARM" ("Enum")) -> (s? t:f=w1024:T6)
              }
              frame "Exit" {
                n377 = for {
                  shift-right: [w1047] -> w1044
                  shift-left: w1041 -> [w1048]
                  tunnel: string[] ["STOP", "RESET ENCODERS", "RESET YAW", "ARDUINO MODE 0"] -> [w1046] mode=indexing
                  n378 = Enqueue Element(queue=w1048, element=w1046) -> (queue out=w1047:refnum<queue>)  [unwired: 2 in, 2 out]
                }
              }
            }
            n379 = Bundle By Name(cluster=w1007, "yStepper desired"=w1003) -> (w1006:T10)
          }
          frame 21 {
            # ">>> yStepper command>>>"
            # ">> Manual override >>"
            n380 = Dequeue Element(queue=w1058, timeout in ms (-1)=w1057, error in (no error)=w1059) -> (element=w1056:T7)  [unwired: 3 out]
            n381 = Equal?(x=w1055, y=u8 1) -> (x = y?=w1053:bool)
            n382 = case shown="\"None\", Default" w1056 {
              tunnel: [w1069 State_Type_Definitions."True Stop" ("Enum")] -> w1060
              tunnel: [w1072 w1089] -> w1061
              tunnel: [State_Type_Definitions."Idle" ("Enum") State_Type_Definitions."Shutdown" ("Enum")] -> w1062
              tunnel: w1053 -> [w1068 _]
              tunnel: w1052 -> [w1067 _]
              tunnel: w1051 -> [w1063 w1086]
              frame "None", Default {
                # "Stays in Task 5F until stepper reaches desired \nheight"
                # "T: Go back to idle, F: Continue with task\""
                # ">> Manual override >>"
                n383 = case shown="True" w1068 {
                  tunnel: [w1076 w1082] -> w1072
                  tunnel: w1063 -> [w1074 w1080]
                  frame False {
                    n384 = for {
                      tunnel: string[] ["Z STEPPER GRAB HEIGHT", "READ STEPPER VALUES"] ("element") -> [w1077] mode=indexing
                      shift-right: [w1079] -> w1076
                      shift-left: w1074 -> [w1078]
                      n385 = Enqueue Element(queue=w1078, element=w1077) -> (queue out=w1079:refnum<queue>)  [unwired: 2 in, 2 out]
                    }
                  }
                  frame True {
                    n386 = for {
                      shift-right: [w1084] -> w1082
                      shift-left: w1080 -> [w1085]
                      tunnel: string[] ["SET TIMER 5", "CLOSE CLAW", ""] -> [w1083] mode=indexing
                      n387 = Enqueue Element(queue=w1085, element=w1083) -> (queue out=w1084:refnum<queue>)  [unwired: 2 in, 2 out]
                    }
                  }
                }
                n388 = Or(x=w1068, y=w1067) -> (x .or. y?=w1070:bool)
                n389 = Select(t=State_Type_Definitions."True Stop" ("Enum"), s=w1067, f=State_Type_Definitions."Task 5G: CLOSE CLAW" ("Enum")) -> (s? t:f=w1064:T6)
                n390 = Select(t=w1064, s=w1070, f=State_Type_Definitions."Task 5F: ARM GRAB HEIGHT" ("Enum")) -> (s? t:f=w1069:T6)
              }
              frame "Exit" {
                n391 = for {
                  shift-right: [w1092] -> w1089
                  shift-left: w1086 -> [w1093]
                  tunnel: string[] ["STOP", "RESET ENCODERS", "RESET YAW", "ARDUINO MODE 0"] -> [w1091] mode=indexing
                  n392 = Enqueue Element(queue=w1093, element=w1091) -> (queue out=w1092:refnum<queue>)  [unwired: 2 in, 2 out]
                }
              }
            }
          }
          frame 22 {
            # ">>> yStepper command>>>"
            # ">> Manual override >>"
            n393 = Dequeue Element(queue=w1103, timeout in ms (-1)=w1102, error in (no error)=w1101) -> (element=w1100:T7)  [unwired: 3 out]
            n394 = case shown="\"None\", Default" w1100 {
              tunnel: [w1112 State_Type_Definitions."True Stop" ("Enum")] -> w1105
              tunnel: [w1115 w1132] -> w1098
              tunnel: [State_Type_Definitions."Idle" ("Enum") State_Type_Definitions."Shutdown" ("Enum")] -> w1097
              tunnel: w1099 -> [w1106 _]
              tunnel: w1104 -> [w1111 w1129]
              tunnel: w1095 -> [w1110 _]
              frame "None", Default {
                # ">> Is time up? >>"
                # "Determines if object is in range to pick up"
                # ">> Manual override >>"
                n395 = case shown="True" w1110 {
                  tunnel: [w1119 w1125] -> w1115
                  tunnel: w1111 -> [w1117 w1123]
                  frame False {
                    n396 = for {
                      tunnel: string[] ["CLOSE CLAW", "START TIMER"] ("element") -> [w1120] mode=indexing
                      shift-right: [w1122] -> w1119
                      shift-left: w1117 -> [w1121]
                      n397 = Enqueue Element(queue=w1121, element=w1120) -> (queue out=w1122:refnum<queue>)  [unwired: 2 in, 2 out]
                    }
                  }
                  frame True {
                    n398 = for {
                      shift-right: [w1127] -> w1125
                      shift-left: w1123 -> [w1128]
                      tunnel: string[] ["READ STEPPER VALUES", "", ""] -> [w1126] mode=indexing
                      n399 = Enqueue Element(queue=w1128, element=w1126) -> (queue out=w1127:refnum<queue>)  [unwired: 2 in, 2 out]
                    }
                  }
                }
                n400 = Or(x=w1110, y=w1106) -> (x .or. y?=w1113:bool)
                n401 = Select(t=State_Type_Definitions."True Stop" ("Enum"), s=w1106, f=State_Type_Definitions."Task 5H: RAISE ARM" ("Enum")) -> (s? t:f=w1108:T6)
                n402 = Select(t=w1108, s=w1113, f=State_Type_Definitions."Task 5G: CLOSE CLAW" ("Enum")) -> (s? t:f=w1112:T6)
              }
              frame "Exit" {
                n403 = for {
                  shift-right: [w1135] -> w1132
                  shift-left: w1129 -> [w1136]
                  tunnel: string[] ["STOP", "RESET ENCODERS", "RESET YAW", "ARDUINO MODE 0"] -> [w1134] mode=indexing
                  n404 = Enqueue Element(queue=w1136, element=w1134) -> (queue out=w1135:refnum<queue>)  [unwired: 2 in, 2 out]
                }
              }
            }
          }
          frame 23 {
            # ">>> yStepper command>>>"
            # ">> Manual override >>"
            n405 = Dequeue Element(queue=w1146, timeout in ms (-1)=w1145, error in (no error)=w1147) -> (element=w1144:T7)  [unwired: 3 out]
            n406 = Equal?(x=w1143, y=u8 60) -> (x = y?=w1141:bool)
            n407 = case shown="\"None\", Default" w1144 {
              tunnel: [w1157 State_Type_Definitions."True Stop" ("Enum")] -> w1148
              tunnel: [w1160 w1177] -> w1149
              tunnel: [State_Type_Definitions."Idle" ("Enum") State_Type_Definitions."Shutdown" ("Enum")] -> w1150
              tunnel: w1141 -> [w1156 _]
              tunnel: w1140 -> [w1155 _]
              tunnel: w1139 -> [w1151 w1174]
              frame "None", Default {
                # "Stays in Task 5_A until stepper reaches desired \nheight"
                # "T: Go back to idle, F: Continue with task\""
                # ">> Manual override >>"
                n408 = case shown="False" w1156 {
                  tunnel: [w1164 w1170] -> w1160
                  tunnel: w1151 -> [w1162 w1168]
                  frame False {
                    n409 = for {
                      tunnel: string[] ["Z STEPPER CAM HEIGHT", "READ STEPPER VALUES"] ("element") -> [w1165] mode=indexing
                      shift-right: [w1167] -> w1164
                      shift-left: w1162 -> [w1166]
                      n410 = Enqueue Element(queue=w1166, element=w1165) -> (queue out=w1167:refnum<queue>)  [unwired: 2 in, 2 out]
                    }
                  }
                  frame True {
                    n411 = for {
                      shift-right: [w1172] -> w1170
                      shift-left: w1168 -> [w1173]
                      tunnel: string[] ["ARDUINO - ULTRASONIC", "READ ULTRASONIC", ""] -> [w1171] mode=indexing
                      n412 = Enqueue Element(queue=w1173, element=w1171) -> (queue out=w1172:refnum<queue>)  [unwired: 2 in, 2 out]
                    }
                  }
                }
                n413 = Or(x=w1156, y=w1155) -> (x .or. y?=w1158:bool)
                n414 = Select(t=State_Type_Definitions."True Stop" ("Enum"), s=w1155, f=State_Type_Definitions."True Stop" ("Enum")) -> (s? t:f=w1152:T6)
                n415 = Select(t=w1152, s=w1158, f=State_Type_Definitions."Task 5H: RAISE ARM" ("Enum")) -> (s? t:f=w1157:T6)
              }
              frame "Exit" {
                n416 = for {
                  shift-right: [w1180] -> w1177
                  shift-left: w1174 -> [w1181]
                  tunnel: string[] ["STOP", "RESET ENCODERS", "RESET YAW", "ARDUINO MODE 0"] -> [w1179] mode=indexing
                  n417 = Enqueue Element(queue=w1181, element=w1179) -> (queue out=w1180:refnum<queue>)  [unwired: 2 in, 2 out]
                }
              }
            }
          }
          frame 24 {
            # ">>> yStepper command>>>"
            n418 = Dequeue Element(queue=w1190, timeout in ms (-1)=w1189, error in (no error)=w1188) -> (element=w1195:T7)  [unwired: 3 out]
            n419 = Equal?(x=w1186, y=u8 60) -> (x = y?=w1185:bool)
            n420 = case shown="\"None\", Default" w1195 {
              tunnel: [w1202 State_Type_Definitions."True Stop" ("Enum")] -> w1193
              tunnel: [w1201 w1219] -> w1192
              tunnel: [State_Type_Definitions."Idle" ("Enum") State_Type_Definitions."Shutdown" ("Enum")] -> w1194
              tunnel: w1191 -> [w1197 _]
              tunnel: w1187 -> [w1199 _]
              tunnel: w1185 -> [w1196 _]
              frame "None", Default {
                n421 = case shown="False" w1196 {
                  tunnel: [w1207 w1213] -> w1201
                  tunnel: w1199 -> [w1205 w1211]
                  frame False {
                    n422 = for {
                      tunnel: string[] ["Z STEPPER CAM HEIGHT", "READ STEPPER VALUES"] ("element") -> [w1208] mode=indexing
                      shift-right: [w1210] -> w1207
                      shift-left: w1205 -> [w1209]
                      n423 = Enqueue Element(queue=w1209, element=w1208) -> (queue out=w1210:refnum<queue>)  [unwired: 2 in, 2 out]
                    }
                  }
                  frame True {
                    n424 = for {
                      shift-right: [w1215] -> w1213
                      shift-left: w1211 -> [w1216]
                      tunnel: string[] ["CAM ACQ", "OPEN LOG CAM"] -> [w1214] mode=indexing
                      n425 = Enqueue Element(queue=w1216, element=w1214) -> (queue out=w1215:refnum<queue>)  [unwired: 2 in, 2 out]
                    }
                  }
                }
                n426 = Or(x=w1196, y=w1197) -> (x .or. y?=w1198:bool)
                n427 = Select(t=State_Type_Definitions."Task 6_B" ("Enum"), s=w1198, f=State_Type_Definitions."Task 6_A" ("Enum")) -> (s? t:f=w1202:T6)
              }
              frame "Exit" {
                n428 = for {
                  shift-right: [w1222] -> w1219
                  shift-left: _ -> [w1223]
                  tunnel: string[] ["STOP", "RESET ENCODERS", "RESET YAW", "ARDUINO MODE 0"] -> [w1221] mode=indexing
                  n429 = Enqueue Element(queue=w1223, element=w1221) -> (queue out=w1222:refnum<queue>)  [unwired: 2 in, 2 out]
                }
              }
            }
          }
          frame 25 {
            # ">>> yStepper command>>>"
            n430 = Dequeue Element(queue=w1234, timeout in ms (-1)=w1232, error in (no error)=w1233) -> (element=w1231:T7)  [unwired: 3 out]
            n431 = case shown="\"None\", Default" w1231 {
              tunnel: [w1241 State_Type_Definitions."True Stop" ("Enum")] -> w1227
              tunnel: [w1240 w1259] -> w1235
              tunnel: [State_Type_Definitions."Idle" ("Enum") State_Type_Definitions."Shutdown" ("Enum")] -> w1228
              tunnel: w1230 -> [w1236 _]
              tunnel: w1229 -> [w1238 _]
              tunnel: w1226 -> [w1237 w1256]
              frame "None", Default {
                # ">> Manual override >>"
                n432 = case shown="True" w1238 {
                  tunnel: [w1246 w1252] -> w1240
                  tunnel: w1237 -> [w1245 w1250]
                  frame False {
                    n433 = for {
                      shift-right: [w1249] -> w1246
                      shift-left: w1245 -> [w1248]
                      tunnel: string[] ["CAM ACQ", "PROCESS IMAGE", "OPEN CLAW"] -> [w1247] mode=indexing
                      n434 = Enqueue Element(queue=w1248, element=w1247) -> (queue out=w1249:refnum<queue>)  [unwired: 2 in, 2 out]
                    }
                  }
                  frame True {
                    n435 = for {
                      shift-right: [w1254] -> w1252
                      shift-left: w1250 -> [w1255]
                      tunnel: string[] ["CAM ACQ", "PROCESS IMAGE", "CLOSE CLAW"] -> [w1253] mode=indexing
                      n436 = Enqueue Element(queue=w1255, element=w1253) -> (queue out=w1254:refnum<queue>)  [unwired: 2 in, 2 out]
                    }
                  }
                }
                n437 = Select(t=State_Type_Definitions."True Stop" ("Enum"), s=w1236, f=State_Type_Definitions."Task 6_B" ("Enum")) -> (s? t:f=w1241:T6)
              }
              frame "Exit" {
                # ">> State after true stop >>"
                # ">> Goes to true stop >>"
                n438 = for {
                  shift-right: [w1262] -> w1259
                  shift-left: w1256 -> [w1263]
                  tunnel: string[] ["STOP", "RESET ENCODERS", "RESET YAW", ""] -> [w1261] mode=indexing
                  n439 = Enqueue Element(queue=w1263, element=w1261) -> (queue out=w1262:refnum<queue>)  [unwired: 2 in, 2 out]
                }
              }
            }
          }
          frame 38 {
            # ">> Stepper height reeached >>"
            # ">>> yStepper command>>>"
            # ">> Manual override >>"
            n440 = Dequeue Element(queue=w1274, timeout in ms (-1)=w1269, error in (no error)=w1273) -> (element=w1277:T7)  [unwired: 3 out]
            n441 = Equal?(x=w1271, y=u8 60) -> (x = y?=w1275:bool)
            n442 = case shown="\"None\", Default" w1277 {
              tunnel: [w1288 State_Type_Definitions."True Stop" ("Enum")] -> w1267
              tunnel: [w1286 w1303] -> w1266
              tunnel: w1270 -> [w1285 _]
              tunnel: w1272 -> [w1279 _]
              tunnel: [State_Type_Definitions."Idle" ("Enum") State_Type_Definitions."Shutdown" ("Enum")] -> w1268
              tunnel: w1275 -> [w1278 _]
              frame "None", Default {
                # ">> WIill proceed to part ii if not manual override >>"
                # ">>If ENABLE or Trigger is set to true>>"
                n443 = Or(x=w1278, y=w1279) -> (x .or. y?=w1280:bool)
                n444 = case shown="True" w1278 {
                  tunnel: [w1291 w1297] -> w1286
                  tunnel: w1285 -> [w1290 w1296]
                  frame False {
                    n445 = for {
                      shift-right: [w1293] -> w1291
                      shift-left: w1290 -> [w1294]
                      tunnel: string[] ["Z STEPPER CAM HEIGHT", "READ STEPPER VALUES"] ("element") -> [w1292] mode=indexing
                      n446 = Enqueue Element(queue=w1294, element=w1292) -> (queue out=w1293:refnum<queue>)  [unwired: 2 in, 2 out]
                    }
                  }
                  frame True {
                    n447 = for {
                      shift-right: [w1299] -> w1297
                      shift-left: w1296 -> [w1300]
                      tunnel: string[] ["ARDUINO - ULTRASONIC", "READ ULTRASONIC", "", "", "", ""] -> [w1298] mode=indexing
                      n448 = Enqueue Element(queue=w1300, element=w1298) -> (queue out=w1299:refnum<queue>)  [unwired: 2 in, 2 out]
                    }
                  }
                }
                n449 = Select(t=State_Type_Definitions."True Stop" ("Enum"), s=w1279, f=State_Type_Definitions."Task 9B: Rotate to Angle" ("Enum")) -> (s? t:f=w1282:T6)
                n450 = Select(t=w1282, s=w1280, f=State_Type_Definitions."Task 9A: Raise Arm" ("Enum")) -> (s? t:f=w1288:T6)
              }
              frame "Exit" {
                n451 = for {
                  shift-right: [w1306] -> w1303
                  shift-left: _ -> [w1307]
                  tunnel: string[] ["STOP", "RESET ENCODERS", "RESET YAW", ""] -> [w1305] mode=indexing
                  n452 = Enqueue Element(queue=w1307, element=w1305) -> (queue out=w1306:refnum<queue>)  [unwired: 2 in, 2 out]
                }
              }
            }
          }
          frame 39 {
            # ">>> yStepper command>>>"
            n453 = Dequeue Element(queue=w1320, timeout in ms (-1)=w1319, error in (no error)=w1318) -> (element=w1322:T7)  [unwired: 3 out]
            n454 = In Range and Coerce(upper limit=305.0, x=w1312, lower limit=295.0) -> (In Range?=w1309:bool)  [unwired: 1 out]
            n455 = case shown="\"None\", Default" w1322 {
              tunnel: w1313 -> [w1325 _]
              tunnel: [w1333 State_Type_Definitions."True Stop" ("Enum")] -> w1315
              tunnel: w1321 -> [w1331 w1349]
              tunnel: [w1330 w1348] -> w1314
              tunnel: [State_Type_Definitions."Idle" ("Enum") State_Type_Definitions."Shutdown" ("Enum")] -> w1316
              tunnel: w1309 -> [w1323 _]
              frame "None", Default {
                n456 = Or(x=w1323, y=w1325) -> (x .or. y?=w1324:bool)
                n457 = case shown="True" w1323 {
                  tunnel: w1331 -> [w1336 w1342]
                  tunnel: [w1335 w1340] -> w1330
                  frame False {
                    n458 = for {
                      shift-right: [w1338] -> w1335
                      shift-left: w1336 -> [w1339]
                      tunnel: string[] ["READ NAVX", "R-ACW"] ("element") -> [w1337] mode=indexing
                      n459 = Enqueue Element(queue=w1339, element=w1337) -> (queue out=w1338:refnum<queue>)  [unwired: 2 in, 2 out]
                    }
                  }
                  frame True {
                    n460 = for {
                      shift-right: [w1344] -> w1340
                      shift-left: w1342 -> [w1345]
                      tunnel: string[] ["STOP", "RESET ENCODERS", "RESET YAW", ""] -> [w1343] mode=indexing
                      n461 = Enqueue Element(queue=w1345, element=w1343) -> (queue out=w1344:refnum<queue>)  [unwired: 2 in, 2 out]
                    }
                  }
                }
                n462 = Select(t=State_Type_Definitions."True Stop" ("Enum"), s=w1325, f=State_Type_Definitions."Task 9C: Rotation alignmnet") -> (s? t:f=w1327:u16)
                n463 = Select(t=w1327, s=w1324, f=State_Type_Definitions."Task 9B: Rotate to Angle" ("Enum")) -> (s? t:f=w1333:u16)
              }
              frame "Exit" {
                n464 = for {
                  shift-right: [w1352] -> w1348
                  shift-left: w1349 -> [w1353]
                  tunnel: string[] ["STOP", "RESET ENCODERS", "RESET YAW", ""] -> [w1351] mode=indexing
                  n465 = Enqueue Element(queue=w1353, element=w1351) -> (queue out=w1352:refnum<queue>)  [unwired: 2 in, 2 out]
                }
              }
            }
          }
          frame 33 {
            # ">>> yStepper command>>>"
            n466 = Dequeue Element(queue=w1363, timeout in ms (-1)=w1362, error in (no error)=w1361) -> (element=w1364:T7)  [unwired: 3 out]
            n467 = case shown="\"None\", Default" w1364 {
              tunnel: w1359 -> [w1365 _]
              tunnel: [w1373 State_Type_Definitions."True Stop" ("Enum")] -> w1356
              tunnel: w1360 -> [w1371 w1389]
              tunnel: [w1370 w1388] -> w1355
              tunnel: [State_Type_Definitions."Idle" ("Enum") State_Type_Definitions."Shutdown" ("Enum")] -> w1358
              frame "None", Default {
                n468 = case shown="True" w1365 {
                  tunnel: w1371 -> [w1376 w1382]
                  tunnel: [w1375 w1380] -> w1370
                  frame False {
                    n469 = for {
                      shift-right: [w1378] -> w1375
                      shift-left: w1376 -> [w1379]
                      tunnel: string[] ["READ IR", "FORWARD - IR ASSIST"] ("element") -> [w1377] mode=indexing
                      n470 = Enqueue Element(queue=w1379, element=w1377) -> (queue out=w1378:refnum<queue>)  [unwired: 2 in, 2 out]
                    }
                  }
                  frame True {
                    n471 = for {
                      shift-right: [w1384] -> w1380
                      shift-left: w1382 -> [w1385]
                      tunnel: string[] ["STOP", "RESET ENCODERS", "RESET YAW", ""] -> [w1383] mode=indexing
                      n472 = Enqueue Element(queue=w1385, element=w1383) -> (queue out=w1384:refnum<queue>)  [unwired: 2 in, 2 out]
                    }
                  }
                }
                n473 = Select(t=State_Type_Definitions."True Stop" ("Enum"), s=w1365, f=State_Type_Definitions."True Stop") -> (s? t:f=w1367:T6)
                n474 = Select(t=w1367, s=w1365, f=State_Type_Definitions."Task 9C: Rotation alignmnet" ("Enum")) -> (s? t:f=w1373:u16)
              }
              frame "Exit" {
                n475 = for {
                  shift-right: [w1392] -> w1388
                  shift-left: w1389 -> [w1393]
                  tunnel: string[] ["STOP", "RESET ENCODERS", "RESET YAW", ""] -> [w1391] mode=indexing
                  n476 = Enqueue Element(queue=w1393, element=w1391) -> (queue out=w1392:refnum<queue>)  [unwired: 2 in, 2 out]
                }
              }
            }
          }
          frame 27 {
            # ">>> yStepper command>>>"
            # ">> Manual override >>"
            n477 = Dequeue Element(queue=w1403, timeout in ms (-1)=w1402, error in (no error)=w1404) -> (element=w1401:T7)  [unwired: 3 out]
            n478 = Equal?(x=w1400, y=u8 60) -> (x = y?=w1398:bool)
            n479 = case shown="\"None\", Default" w1401 {
              tunnel: [w1414 State_Type_Definitions."True Stop" ("Enum")] -> w1405
              tunnel: [w1417 w1434] -> w1406
              tunnel: [State_Type_Definitions."Idle" ("Enum") State_Type_Definitions."Shutdown" ("Enum")] -> w1407
              tunnel: w1398 -> [w1413 _]
              tunnel: w1397 -> [w1412 _]
              tunnel: w1396 -> [w1408 w1431]
              frame "None", Default {
                # "Stays in Task 5_A until stepper reaches desired \nheight"
                # "T: Go back to idle, F: Continue with task\""
                # ">> Manual override >>"
                n480 = case shown="True" w1413 {
                  tunnel: [w1421 w1427] -> w1417
                  tunnel: w1408 -> [w1419 w1425]
                  frame False {
                    n481 = for {
                      tunnel: string[] ["Z STEPPER CAM HEIGHT", "READ STEPPER VALUES"] ("element") -> [w1422] mode=indexing
                      shift-right: [w1424] -> w1421
                      shift-left: w1419 -> [w1423]
                      n482 = Enqueue Element(queue=w1423, element=w1422) -> (queue out=w1424:refnum<queue>)  [unwired: 2 in, 2 out]
                    }
                  }
                  frame True {
                    n483 = for {
                      shift-right: [w1429] -> w1427
                      shift-left: w1425 -> [w1430]
                      tunnel: string[] ["ARDUINO - ULTRASONIC", "READ ULTRASONIC", ""] -> [w1428] mode=indexing
                      n484 = Enqueue Element(queue=w1430, element=w1428) -> (queue out=w1429:refnum<queue>)  [unwired: 2 in, 2 out]
                    }
                  }
                }
                n485 = Or(x=w1413, y=w1412) -> (x .or. y?=w1415:bool)
                n486 = Select(t=State_Type_Definitions."True Stop" ("Enum"), s=w1412, f=State_Type_Definitions."Task 8B: MOVE TO BOX" ("Enum")) -> (s? t:f=w1409:T6)
                n487 = Select(t=w1409, s=w1415, f=State_Type_Definitions."Task 8A: RAISE ARM" ("Enum")) -> (s? t:f=w1414:T6)
              }
              frame "Exit" {
                n488 = for {
                  shift-right: [w1437] -> w1434
                  shift-left: w1431 -> [w1438]
                  tunnel: string[] ["STOP", "RESET ENCODERS", "RESET YAW", "ARDUINO MODE 0"] -> [w1436] mode=indexing
                  n489 = Enqueue Element(queue=w1438, element=w1436) -> (queue out=w1437:refnum<queue>)  [unwired: 2 in, 2 out]
                }
              }
            }
          }
          frame 28 {
            w1445 = u8 20 ("y")
            # ">>> yStepper command>>>"
            n490 = Less?(x=w1442, y=w1445) -> (x < y?=w1443:bool)
            n491 = Dequeue Element(queue=w1449, timeout in ms (-1)=w1448, error in (no error)=w1450) -> (element=w1447:T7)  [unwired: 3 out]
            n492 = Less?(x=w1441, y=w1445) -> (x < y?=w1444:bool)
            n493 = And(x=w1444, y=w1443) -> (x .and. y?=w1440:bool)
            n494 = case shown="\"None\", Default" w1447 {
              tunnel: [w1462 State_Type_Definitions."True Stop" ("Enum")] -> w1452
              tunnel: [w1465 w1482] -> w1451
              tunnel: [State_Type_Definitions."Idle" ("Enum") State_Type_Definitions."Shutdown" ("Enum")] -> w1453
              tunnel: w1455 -> [w1461 _]
              tunnel: w1454 -> [w1457 w1479]
              tunnel: w1440 -> [w1456 _]
              frame "None", Default {
                # "Stays in Task 5_B to capture image over 5 seconds"
                # "T: Go back to idle, F: Continue with task\""
                # ">> Manual override >>"
                n495 = case shown="True" w1456 {
                  tunnel: [w1469 w1475] -> w1465
                  tunnel: w1457 -> [w1467 w1473]
                  frame False {
                    n496 = for {
                      tunnel: string[] ["FORWARD", "READ ULTRASONIC", "READ NAVX"] ("element") -> [w1470] mode=indexing
                      shift-right: [w1472] -> w1469
                      shift-left: w1467 -> [w1471]
                      n497 = Enqueue Element(queue=w1471, element=w1470) -> (queue out=w1472:refnum<queue>)  [unwired: 2 in, 2 out]
                    }
                  }
                  frame True {
                    n498 = for {
                      shift-right: [w1477] -> w1475
                      shift-left: w1473 -> [w1478]
                      tunnel: string[] ["STOP", "RESET ENCODERS", "OPEN LOG CAM", "SET TIMER 5"] -> [w1476] mode=indexing
                      n499 = Enqueue Element(queue=w1478, element=w1476) -> (queue out=w1477:refnum<queue>)  [unwired: 2 in, 2 out]
                    }
                  }
                }
                n500 = Or(x=w1456, y=w1461) -> (x .or. y?=w1463:bool)
                n501 = Select(t=State_Type_Definitions."True Stop" ("Enum"), s=w1461, f=State_Type_Definitions."Task 8C: CAM BURST" ("Enum")) -> (s? t:f=w1458:T6)
                n502 = Select(t=w1458, s=w1463, f=State_Type_Definitions."Task 8B: MOVE TO BOX" ("Enum")) -> (s? t:f=w1462:T6)
              }
              frame "Exit" {
                n503 = for {
                  shift-right: [w1485] -> w1482
                  shift-left: w1479 -> [w1486]
                  tunnel: string[] ["STOP", "RESET ENCODERS", "RESET YAW", "ARDUINO MODE 0"] -> [w1484] mode=indexing
                  n504 = Enqueue Element(queue=w1486, element=w1484) -> (queue out=w1485:refnum<queue>)  [unwired: 2 in, 2 out]
                }
              }
            }
          }
          frame 29 {
            # ">>> yStepper command>>>"
            # ">> Manual override >>"
            n505 = Dequeue Element(queue=w1496, timeout in ms (-1)=w1495, error in (no error)=w1494) -> (element=w1493:T7)  [unwired: 3 out]
            n506 = case shown="\"None\", Default" w1493 {
              tunnel: [w1505 State_Type_Definitions."True Stop" ("Enum")] -> w1498
              tunnel: [w1508 w1525] -> w1491
              tunnel: [State_Type_Definitions."Idle" ("Enum") State_Type_Definitions."Shutdown" ("Enum")] -> w1490
              tunnel: w1492 -> [w1499 _]
              tunnel: w1497 -> [w1504 w1522]
              tunnel: w1488 -> [w1503 _]
              frame "None", Default {
                # ">> Is time up? >>"
                # "Determines if object is in range to pick up"
                # ">> Manual override >>"
                n507 = case shown="True" w1503 {
                  tunnel: [w1512 w1518] -> w1508
                  tunnel: w1504 -> [w1510 w1516]
                  frame False {
                    n508 = for {
                      tunnel: string[] ["CAM ACQ", "START TIMER"] ("element") -> [w1513] mode=indexing
                      shift-right: [w1515] -> w1512
                      shift-left: w1510 -> [w1514]
                      n509 = Enqueue Element(queue=w1514, element=w1513) -> (queue out=w1515:refnum<queue>)  [unwired: 2 in, 2 out]
                    }
                  }
                  frame True {
                    n510 = for {
                      shift-right: [w1520] -> w1518
                      shift-left: w1516 -> [w1521]
                      tunnel: string[] ["CAM CLOSE", "PROCESS IMAGE", "SET TIMER 5"] -> [w1519] mode=indexing
                      n511 = Enqueue Element(queue=w1521, element=w1519) -> (queue out=w1520:refnum<queue>)  [unwired: 2 in, 2 out]
                    }
                  }
                }
                n512 = Or(x=w1503, y=w1499) -> (x .or. y?=w1506:bool)
                n513 = Select(t=State_Type_Definitions."True Stop" ("Enum"), s=w1499, f=State_Type_Definitions."Task 8D: PROCESS IMAGE" ("Enum")) -> (s? t:f=w1501:T6)
                n514 = Select(t=w1501, s=w1506, f=State_Type_Definitions."Task 8C: CAM BURST" ("Enum")) -> (s? t:f=w1505:T6)
              }
              frame "Exit" {
                n515 = for {
                  shift-right: [w1528] -> w1525
                  shift-left: w1522 -> [w1529]
                  tunnel: string[] ["STOP", "RESET ENCODERS", "RESET YAW", "ARDUINO MODE 0"] -> [w1527] mode=indexing
                  n516 = Enqueue Element(queue=w1529, element=w1527) -> (queue out=w1528:refnum<queue>)  [unwired: 2 in, 2 out]
                }
              }
            }
          }
          frame 30 {
            # ">>> yStepper command>>>"
            n517 = Dequeue Element(queue=w1536, timeout in ms (-1)=w1535, error in (no error)=w1534) -> (element=w1533:T7)  [unwired: 3 out]
            n518 = case shown="\"None\", Default" w1533 {
              tunnel: [w1548 State_Type_Definitions."True Stop" ("Enum")] -> w1540
              tunnel: [w1551 w1568] -> w1539
              tunnel: [State_Type_Definitions."Idle" ("Enum") State_Type_Definitions."Shutdown" ("Enum")] -> w1541
              tunnel: w1537 -> [w1547 _]
              tunnel: w1538 -> [w1543 w1565]
              tunnel: w1531 -> [w1542 _]
              frame "None", Default {
                # ">> T: Breaks out of state loop; F: Stays in loop>>"
                # ">> Manual override >>"
                # ">> Checks if time is up>>"
                # "Stays in Task 5D until the object is detected"
                # "T: Go back to idle, F: Continue with task\""
                # ">> Manual override >>"
                n519 = case shown="True" w1542 {
                  tunnel: [w1555 w1561] -> w1551
                  tunnel: w1543 -> [w1553 w1559]
                  frame False {
                    n520 = for {
                      tunnel: string[] ["START TIMER", "PROCESS IMAGE", ""] ("element") -> [w1556] mode=indexing
                      shift-right: [w1558] -> w1555
                      shift-left: w1553 -> [w1557]
                      n521 = Enqueue Element(queue=w1557, element=w1556) -> (queue out=w1558:refnum<queue>)  [unwired: 2 in, 2 out]
                    }
                  }
                  frame True {
                    n522 = for {
                      shift-right: [w1563] -> w1561
                      shift-left: w1559 -> [w1564]
                      tunnel: string[] ["CAM CLOSE", "RESET ENCODERS", ""] -> [w1562] mode=indexing
                      n523 = Enqueue Element(queue=w1564, element=w1562) -> (queue out=w1563:refnum<queue>)  [unwired: 2 in, 2 out]
                    }
                  }
                }
                n524 = Or(x=w1542, y=w1547) -> (x .or. y?=w1549:bool)
                n525 = Select(t=State_Type_Definitions."True Stop" ("Enum"), s=w1547, f=State_Type_Definitions."Task 8E: ROBOT ADJUST" ("Enum")) -> (s? t:f=w1544:T6)
                n526 = Select(t=w1544, s=w1549, f=State_Type_Definitions."Task 8D: PROCESS IMAGE" ("Enum")) -> (s? t:f=w1548:T6)
              }
              frame "Exit" {
                n527 = for {
                  shift-right: [w1571] -> w1568
                  shift-left: w1565 -> [w1572]
                  tunnel: string[] ["STOP", "RESET ENCODERS", "RESET YAW", "ARDUINO MODE 0"] -> [w1570] mode=indexing
                  n528 = Enqueue Element(queue=w1572, element=w1570) -> (queue out=w1571:refnum<queue>)  [unwired: 2 in, 2 out]
                }
              }
            }
          }
          frame 31 {
            # ">>> Motor control cluster >>>"
            # ">>> yStepper command>>>"
            n529 = Dequeue Element(queue=w1589, timeout in ms (-1)=w1588, error in (no error)=w1587) -> (element=w1586:T7)  [unwired: 3 out]
            n530 = Subtract(x=w1584, y=300.0) -> (x-y=w1582:dbl)
            "x-y" <- w1582
            n531 = formula code="if (error < -80 && error >-300){\ndistance = -20;\nxSpeed = -30;\n}\n\nelse if (error <= 61&&error >= -80){\ndistance = -15;\nxSpeed = -30;\n}\n\nelse if (error <= -51 && error >= -60){\ndistance = -10;\nxSpeed = -30;\n}\n\nelse if (error >= -50 && error <= 50){\ndistance = 0;\nxSpeed = 0;\n}\n\nelse if (error >= 51 && error <= 80){\ndistance = 10;\nxSpeed = 30;\n}\n\nelse if (error >= 81 && error <= 100){\ndistance = 25;\nxSpeed = 30;\n}\n\nelse if (error >= 101){\ndistance = 30;\nxSpeed = 30;\n}\n\nelse{\ndistance = 0;\nxSpeed = 0;\n}"("error"=w1582) -> ("distance"=w1576:dbl, "xSpeed"=w1579:dbl)
            n532 = Greater Or Equal?(x=w1575, y=w1576) -> (x >= y?=w1577:bool)
            n533 = Greater Than 0?(x=w1576) -> (x > 0?=w1578:bool)
            n534 = Less Or Equal?(x=w1575, y=w1576) -> (x <= y?=w1574:bool)
            n535 = Select(t=w1577, s=w1578, f=w1574) -> (s? t:f=w1573:bool)
            n536 = case shown="\"None\", Default" w1586 {
              tunnel: [w1601 State_Type_Definitions."True Stop" ("Enum")] -> w1593
              tunnel: [w1604 w1621] -> w1592
              tunnel: [State_Type_Definitions."Idle" ("Enum") State_Type_Definitions."Shutdown" ("Enum")] -> w1594
              tunnel: w1590 -> [w1600 _]
              tunnel: w1591 -> [w1596 w1618]
              tunnel: w1573 -> [w1595 _]
              frame "None", Default {
                # ">> T: Breaks out of state loop; F: Stays in loop>>"
                # ">> Manual override >>"
                # ">> Checks if time is up>>"
                # "Stays in Task 5D until the object is detected"
                # "T: Go back to idle, F: Continue with task\""
                # ">> Manual override >>"
                n537 = case shown="True" w1595 {
                  tunnel: [w1608 w1614] -> w1604
                  tunnel: w1596 -> [w1606 w1612]
                  frame False {
                    n538 = for {
                      tunnel: string[] ["X AXIS - SLOW", "READ ENCODERS", "READ YAW"] ("element") -> [w1609] mode=indexing
                      shift-right: [w1611] -> w1608
                      shift-left: w1606 -> [w1610]
                      n539 = Enqueue Element(queue=w1610, element=w1609) -> (queue out=w1611:refnum<queue>)  [unwired: 2 in, 2 out]
                    }
                  }
                  frame True {
                    n540 = for {
                      shift-right: [w1616] -> w1614
                      shift-left: w1612 -> [w1617]
                      tunnel: string[] ["CAM CLOSE", "DISPOSE BUFFERS", ""] -> [w1615] mode=indexing
                      n541 = Enqueue Element(queue=w1617, element=w1615) -> (queue out=w1616:refnum<queue>)  [unwired: 2 in, 2 out]
                    }
                  }
                }
                n542 = Or(x=w1595, y=w1600) -> (x .or. y?=w1602:bool)
                n543 = Select(t=State_Type_Definitions."True Stop" ("Enum"), s=w1600, f=State_Type_Definitions."True Stop" ("Enum")) -> (s? t:f=w1597:T6)
                n544 = Select(t=w1597, s=w1602, f=State_Type_Definitions."Task 8E: ROBOT ADJUST" ("Enum")) -> (s? t:f=w1601:T6)
              }
              frame "Exit" {
                n545 = for {
                  shift-right: [w1624] -> w1621
                  shift-left: w1618 -> [w1625]
                  tunnel: string[] ["STOP", "RESET ENCODERS", "RESET YAW", "ARDUINO MODE 0"] -> [w1623] mode=indexing
                  n546 = Enqueue Element(queue=w1625, element=w1623) -> (queue out=w1624:refnum<queue>)  [unwired: 2 in, 2 out]
                }
              }
            }
            n547 = Bundle By Name(cluster=w1581, "xSpeed"=w1579) -> (w1580:T8)
          }
        }
      }
    }
    n548 = local write "Green LED"(w189) -> ()
  }
  n549 = while {
    tunnel: w48 -> [w2194]
    tunnel: w47 -> [w2191]
    stop <- w2188 stop-if-true
    # "Status Loop for Action Queues"
    n550 = Get Queue Status(queue=w2194, return elements? (F)=TRUE) -> (error out=w2190:errorcluster, # elements in queue=→"Action Queue Items":i32, elements=→"Action Queues items":string[])  [unwired: 1 in, 5 out]
    n551 = Get Queue Status(queue=w2191, return elements? (F)=TRUE) -> (# pending remove=→"State Logic Queue Items":i32, error out=w2189:errorcluster, elements=→"elements":T7[])  [unwired: 1 in, 5 out]
    n552 = Merge Errors(w2190, w2189) -> (w2188:errorcluster)
    n553 = Wait (ms)(milliseconds to wait=u32 500) -> ()  [unwired: 1 out]
  }
  n554 = call <vilib>:"DIO Close.vi"("error in (no error)"=w24, "DIO Info In"=w27) -> ()  [unwired: 9 in, 1 out]
  n555 = call <vilib>:"DIO Close.vi"("error in (no error)"=w34, "DIO Info In"=w36) -> ()  [unwired: 9 in, 1 out]
  n556 = call <vilib>:"NavX Close.vi"("error in (no error)"=w8, "NavX Info In"=w7) -> ()  [unwired: 9 in, 1 out]
  n557 = call <vilib>:"DIO Close.vi"("error in (no error)"=w29, "DIO Info In"=w31) -> ()  [unwired: 9 in, 1 out]
  n558 = call <vilib>:"DIO Close.vi"("error in (no error)"=w15, "DIO Info In"=w16) -> ()  [unwired: 9 in, 1 out]
  n559 = call <vilib>:"DIO Close.vi"("error in (no error)"=w10, "DIO Info In"=w11) -> ()  [unwired: 9 in, 1 out]
  n560 = while {
    stop <- w2198 stop-if-true
    n561 = call <vilib>:"RT Get CPU Loads.vi"() -> ("CPU loads"=→"CPU loads":T5[])  [unwired: 10 in, 1 out]
    n562 = Wait (ms)(milliseconds to wait=u32 100) -> ()  [unwired: 1 out]
    n563 = call "FGV Bool.vi"("Init/Read/Write State"=States_for_Action_Engine."Read") -> ("Output node"=w2198:bool)  [unwired: 2 in, 1 out]
  }
  n564 = while {
    stop <- w2202 stop-if-true
    n565 = call "MOTOR CONTROL WITH PID AE.vi"("AE Mode"=MOTOR_CONTROL_WITH_PID_AE_DATA_MODE_TYPE_DEF."Read from AE") -> ("Speed & distance"=→"Speed & distance":T1)  [unwired: 3 in]
    n566 = call "FGV Bool.vi"("Init/Read/Write State"=States_for_Action_Engine."Read") -> ("Output node"=w2202:bool)  [unwired: 2 in, 1 out]
    n567 = Wait (ms)(milliseconds to wait=u32 5) -> ()  [unwired: 1 out]
  }
  n568 = Merge Errors "Merge Errors"(w64, w63) -> (w46:errorcluster)
  n569 = Merge Errors(w50, w46) -> (w45:errorcluster)
  n570 = Destroy User Event(user event=w67, error in=w45) -> ()  [unwired: 1 out]
  n571 = Destroy User Event(user event=w68, error in=w45) -> ()  [unwired: 1 out]
  n572 = Unregister For Events(event registration refnum=w59, error in=w45) -> ()  [unwired: 1 out]
  n573 = Release Queue(queue=w41, error in (no error)=w45) -> (error out=→"error out":errorcluster)  [unwired: 1 in, 2 out]
  n574 = Release Queue(queue=w58, error in (no error)=w45) -> ()  [unwired: 1 in, 3 out]
